vi "Main.vi"() -> ()   [LabVIEW 2014]
uses:
  <vilib>/Utility/config.llb/Write Key (String).vi
  <vilib>/Utility/config.llb/Write Key (Path).vi
  <vilib>/Utility/file.llb/Write To Spreadsheet File (string).vi
  <vilib>/Utility/config.llb/Read Key (String).vi
  <vilib>/Utility/config.llb/Read Key (Path).vi
  <vilib>/Utility/config.llb/NI_LVConfig.lvlib
panel:
  out "错误输出 2":errorcluster caption="错误输出"
  out "B结果信号":bool
  out "A结果信号":bool
  in  "scan A":bool
  in  "scan B":bool
  out "error out 4":errorcluster caption="错误输出"
  out "error out":errorcluster caption="错误输出"
  in  "打印标签路径B/Print label path B/Imprimer le chemin d’accès de l’étiquette B":path=path "D:/序列号B.txt"
  in  "打印标签路径A/Print label path A/Imprimer le chemin d’accès de l’étiquette A":path=path "D:/岚图A.btw"
  in  "3th Shift":timestamp format="%<%H:%M>T"
  in  "2nd Shift":timestamp format="%<%H:%M>T"
  in  "A启动信号":bool
  in  "B启动信号":bool
  in  "扫码在线过程":dbl
  in  "校准时间过程":i8
  out "错误输出  2":errorcluster caption="错误输出"
  out "error out 3":errorcluster
  out "error out 2":errorcluster
  in  "B复位":bool
  in  "A复位":bool
  out "Scan OK B":bool
  out "Scan OK A":bool
  out "错误输出":errorcluster
  in  "错误输入（无错误）":errorcluster
  out "结果 2":string
  in  "合格次数B":u16
  out "泄漏单位 2":string
  out "压力单位 2":string
  in  "检测次数B":u16
  in  "合格状态右":u16
  out "结果压力 B":dbl
  out "结果漏率 B":dbl
  out "合格 2":bool
  out "StepCode 2":u16
  out "Ready 2":bool
  out "StatusResults 2":u16 format="%b"
  out "实时漏率B":dbl
  out "LeakUnit 2":u16(ring) items=["ml/min"=51000, "cm3/s"=0, "cm3/min"=1000, "cm3/h"=2000, "mm3/h"=3000, "CalibartedPascal"=4000, "Pa"=6000, "Bar"=11000, "Kpa"=12000, "PSI"=13000, "Mbar"=14000, "Mpa"=15000, "Inch3/s"=46000, "Inch3/min"=47000, "Inch3/hour"=48000]
  out "PressureUnit 2":u16(ring) items=["cm3/s"=0, "cm3/min"=1000, "cm3/h"=2000, "mm3/h"=3000, "CalibartedPascal"=4000, "Pa"=6000, "Bar"=11000, "Kpa"=12000, "PSI"=13000, "Mbar"=14000, "Mpa"=15000, "Inch3/s"=46000, "Inch3/min"=47000, "Inch3/hour"=48000]
  out "ProgramNumber 2":u16
  out "实时压力B":dbl
  out "读取程序号B":bool
  out "读取程序号A":bool
  out "合格":bool
  out "StepCode":u16
  out "Ready":bool
  out "结果":string
  in  "合格次数A":u16
  out "泄漏单位":string
  out "压力单位":string
  in  "检测次数A":u16
  in  "合格状态左":u16
  out "StatusResults":u16 format="%b"
  out "实时漏率A":dbl
  out "LeakUnit":u16(ring) items=["ml/min"=51000, "cm3/s"=0, "cm3/min"=1000, "cm3/h"=2000, "mm3/h"=3000, "CalibartedPascal"=4000, "Pa"=6000, "Bar"=11000, "Kpa"=12000, "PSI"=13000, "Mbar"=14000, "Mpa"=15000, "Inch3/s"=46000, "Inch3/min"=47000, "Inch3/hour"=48000]
  out "PressureUnit":u16(ring) items=["cm3/s"=0, "cm3/min"=1000, "cm3/h"=2000, "mm3/h"=3000, "CalibartedPascal"=4000, "Pa"=6000, "Bar"=11000, "Kpa"=12000, "PSI"=13000, "Mbar"=14000, "Mpa"=15000, "Inch3/s"=46000, "Inch3/min"=47000, "Inch3/hour"=48000]
  out "ProgramNumber":u16
  out "实时压力A":dbl
  out "结果压力":dbl
  out "结果漏率":dbl
  in  "选项卡控件":T1(tab)
  out "校准倒计时":string
  out "B OK/NG":bool
  out "A OK/NG":bool
  in  "B标签重打":bool
  in  "A标签重打":bool
  in  "扫描枪重连":bool
  out "数字不跳动，表示软件死机 A":i32
  out "Scanner":bool
  out "ATEQ No. B":string
  out "ATEQ No. A":string
  in  "2D Code_B":string
  in  "Single/Dual B":bool
  in  "Total Today B":dbl
  in  "OK Today B":dbl
  in  "Staff B":u16(ring) items=["", "System", "复检", "谌春花", "辛飞琴", "周太珍", "周莎", "焦艳", "李腾", "吴有芳", "", "", "", "", "", "", "", "", "", "", "", "", "", "", ""]
  in  "Part No. B":u16(ring) items=["", "E113015200", "E113015300", "E122015400", "", "", "", "", "", "", "", "", "", "", "", "", "", "", "", "", "", "", "", "", ""]
  in  "B List":string[][](table)
  in  "2D Code_A":string
  in  "Single/Dual A":bool
  in  "Total Today A":dbl
  in  "OK Today A":dbl
  in  "Staff A":u16(ring) items=["", "System", "复检", "谌春花", "辛飞琴", "周太珍", "周莎", "焦艳", "李腾", "吴有芳", "", "", "", "", "", "", "", "", "", "", "", "", "", "", ""]
  in  "Part No. A":u16(ring) items=["", "E113015200", "E113015300", "E122015400", "", "", "", "", "", "", "", "", "", "", "", "", "", "", "", "", "", "", "", "", ""]
  in  "A List":string[][](table)
  out "数字不跳动，表示软件死机B":i32
  out "A Cal. Time":bool caption="A校准时间到"
  out "A OK Sample Req. (2nd)":bool caption="A校准时间到"
  out "A NG Sample Req.（1st)":bool caption="A校准时间到"
  in  "A Start Validation":bool
  out "B Cal. Time":bool caption="A校准时间到"
  out "B OK Sample Req. (2nd)":bool caption="A校准时间到"
  out "B NG Sample Req.（1st)":bool caption="A校准时间到"
  in  "B Start Validation":bool
  in  "密码":string
  in  "Confirm":bool
  in  "Cancel":bool
  in  "登录":u16(ring) items=["管理员", "作业员"]
  in  "A Cancel Validation":bool
  in  "B Cancel Validation":bool
  in  "Calitration Period (Hours)":timestamp format="%<%H:%M>T"
  in  "ATEQ F620 B (Restart Software to Active)":refnum<visa-resource-name>="COM6"
  in  "Language":u16(ring) items=["中文", "English", "Francais"]
  in  "保存确定":bool
  in  "参数设置/Setup/Coup monté":string[][](table) caption="参数设置"
  in  "ATEQ F620 A (Restart Software to Active)":refnum<visa-resource-name>="COM4"
  out "Scanner":bool
  in  "Download B":bool
  in  "Search B":bool
  in  "Finish Time B":timestamp format="%<%H:%M:%S\n%Y/%m/%d>T"
  in  "Result B":u16(ring) items=["", "OK", "NG"]
  in  "2D Code B":string
  in  "Start Time B":timestamp format="%<%H:%M:%S\n%Y/%m/%d>T"
  in  "Download A":bool
  in  "Search A":bool
  in  "Finish Time A":timestamp format="%<%H:%M:%S\n%Y/%m/%d>T"
  in  "Result A":u16(ring) items=["", "OK", "NG"]
  in  "2D Code A":string
  in  "Start Time A":timestamp format="%<%H:%M:%S\n%Y/%m/%d>T"
  in  "A List Search":string[][](table)
  in  "B List Search":string[][](table)
  in  "B自动/手动_Automatic/Manual_Automatique/Manual":bool
  in  "A自动/手动_Automatic/Manual_Automatique/Manual":bool
  in  "B门_Door_Porte：使能_Active_Activer/禁用_Deactive_Désactiver":bool
  in  "B盖章_Stamp_Timbre：后退_Back_Arrière/前进_forward_avant":bool
  in  "B封堵_Blocking_Bloquant：后退_Back_Arrière/前进_forward_avant":bool
  in  "B移载_Transfer_Transfert：后退_Back_Arrière/前进_forward_avant":bool
  in  "B夹紧_Clamping_Serrage：后退_Back_Arrière/前进_forward_avant":bool
  in  "A门_Door_Porte：使能_Active_Activer/禁用_Deactive_Désactiver":bool
  in  "A盖章_Stamp_Timbre：后退_Back_Arrière/前进_forward_avant":bool
  in  "A封堵_Blocking_Bloquant：后退_Back_Arrière/前进_forward_avant":bool
  in  "A移载_Transfer_Transfert：后退_Back_Arrière/前进_forward_avant":bool
  in  "A夹紧_Clamping_Serrage：后退_Back_Arrière/前进_forward_avant":bool
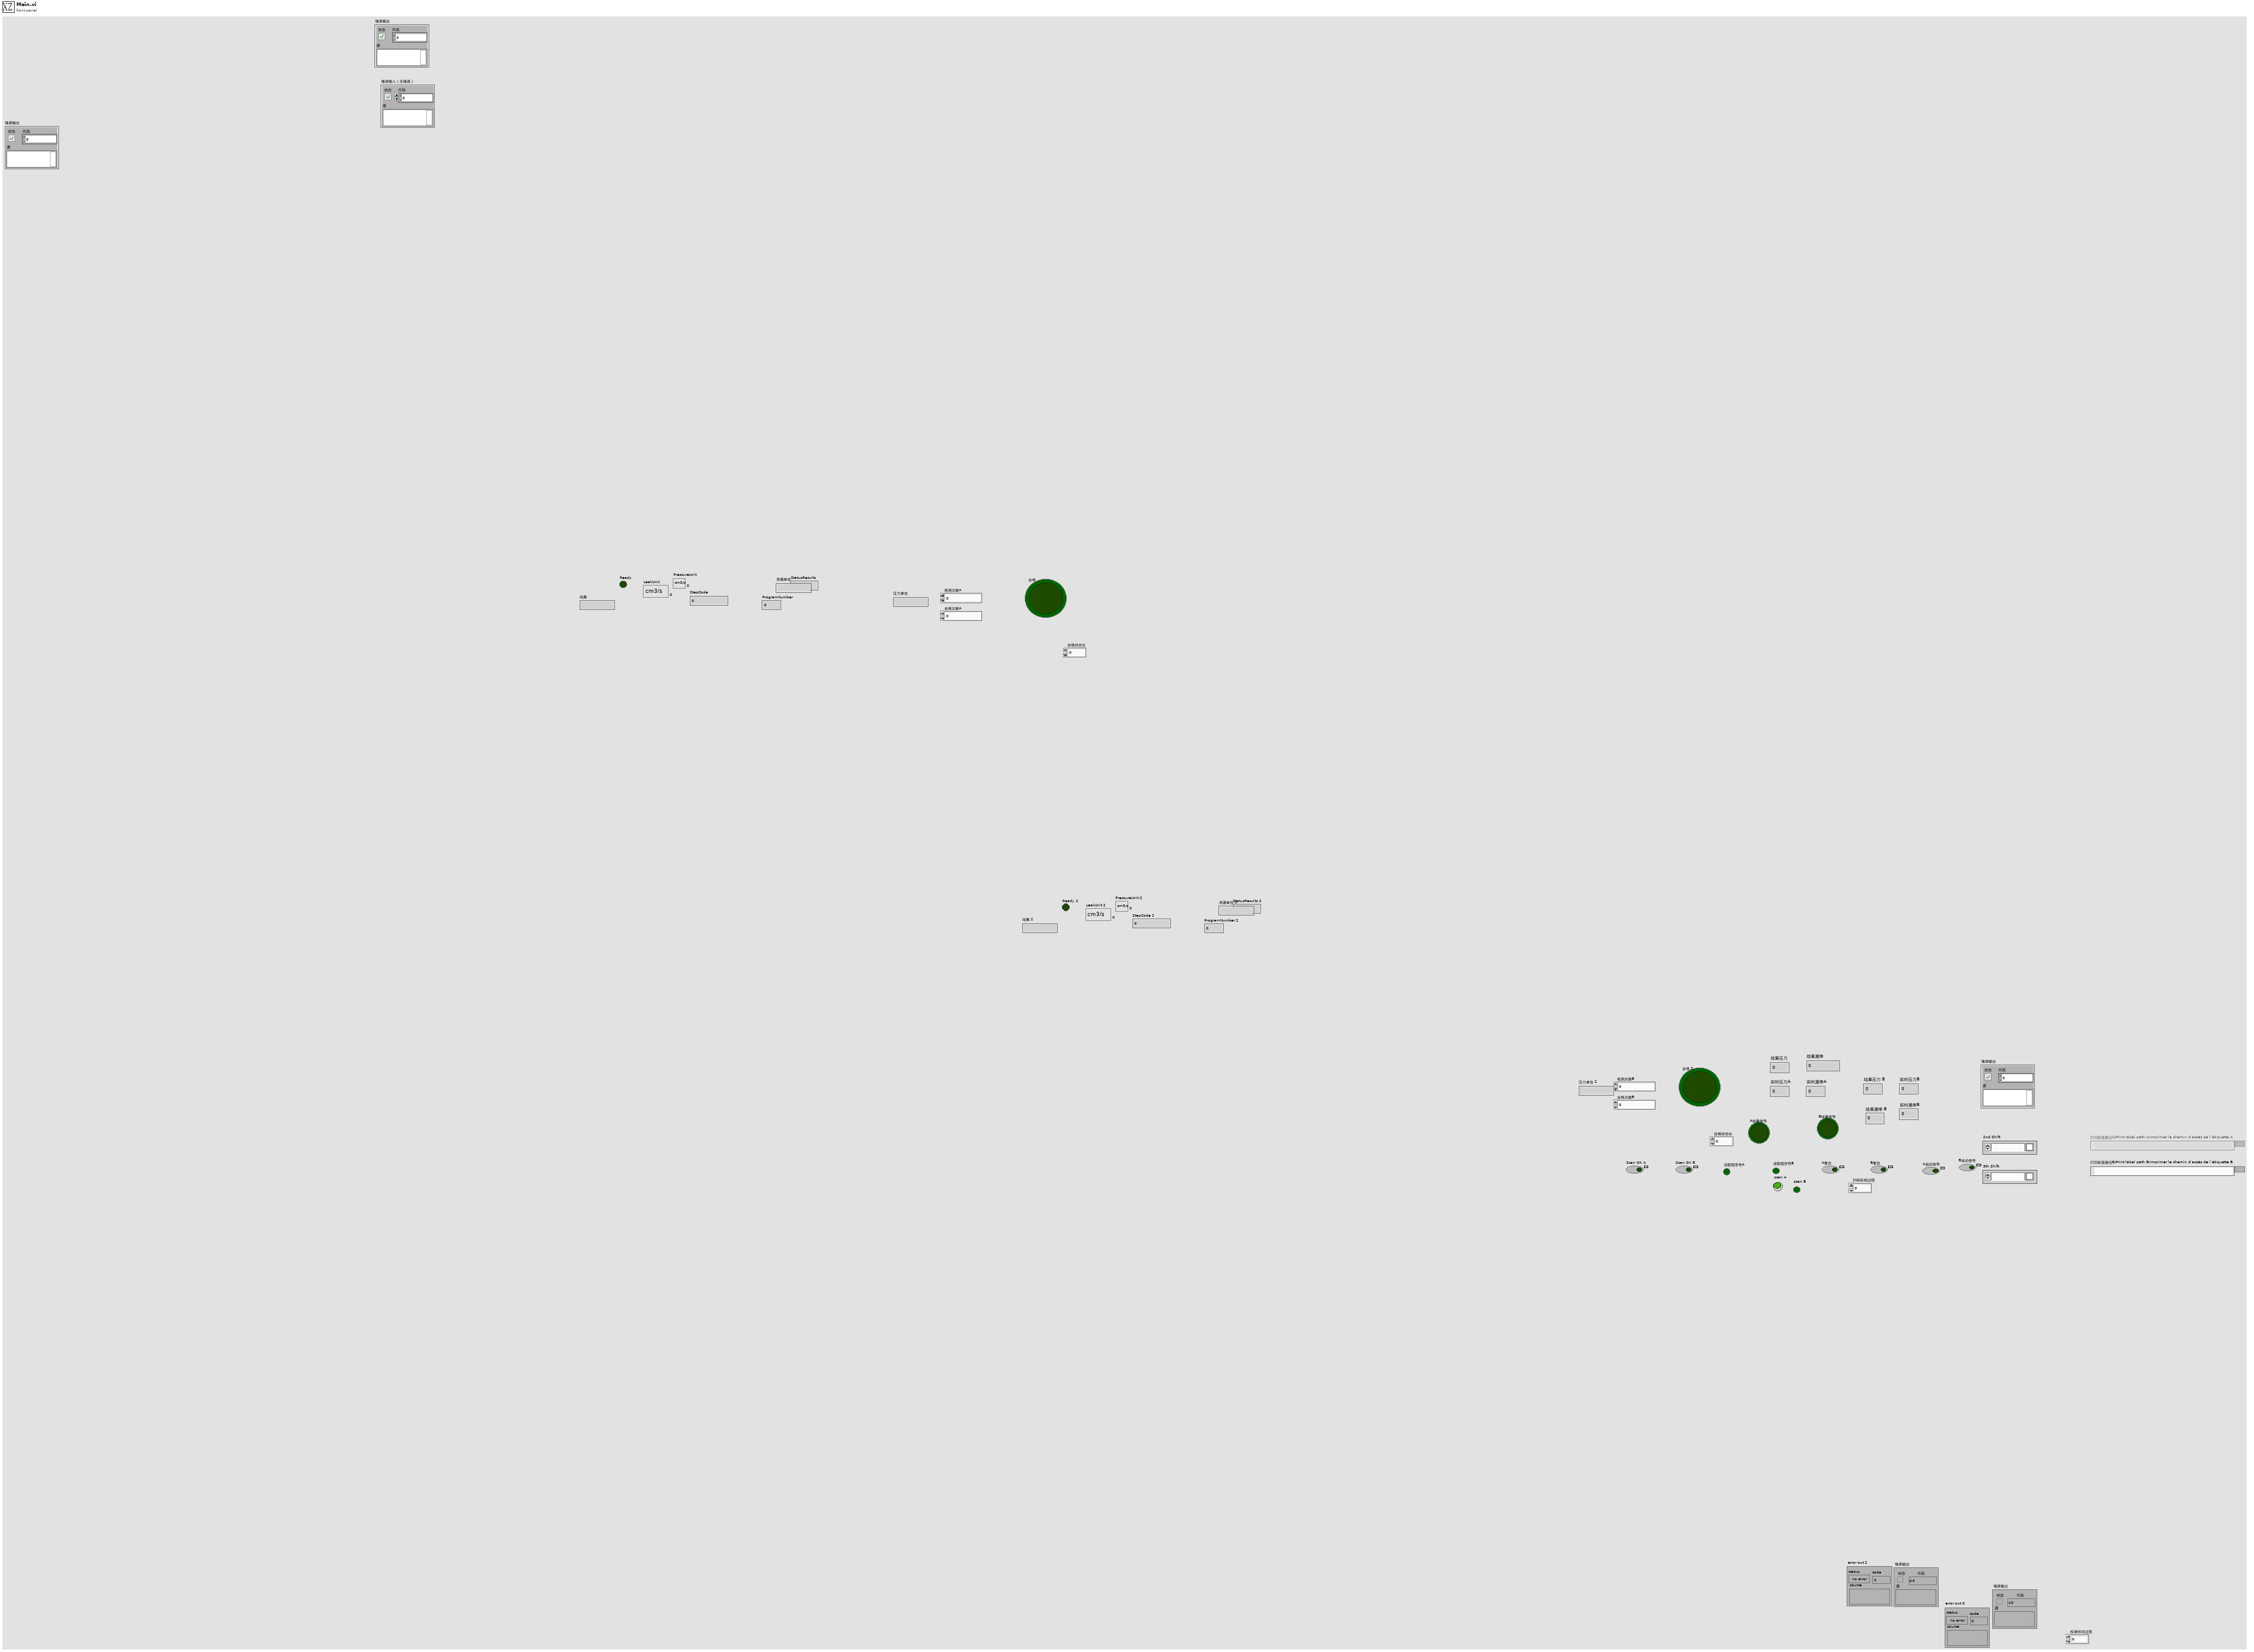
[diagram p1: front panel]
types:
  T1 = enum32{"测试/Main/Principale", "设置/Setup/Coup Monté", "查询/Query/Requête", "手动/Manual/Manuelle"}
  T2 = enum8{"Enabled", "Disabled", "Disabled and Grayed Out"}
  T3 = typedef "NI_LVConfig.lvlib/Config Data RefNum.ctl" = refnum<k1>
  T4 = enum16{"Init", "Loop", "Write LOFF", "Write LON", "Read", "Exit", "Open", "Close"}
  T5 = enum16{"Standard", "Buffered", "CRLF", "Immediate"}
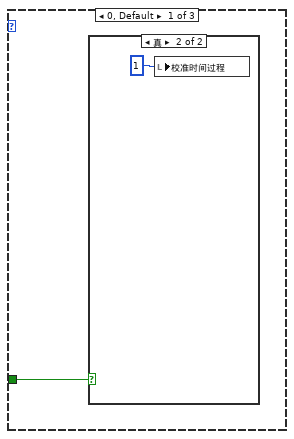
[diagram p3: hidden frame]
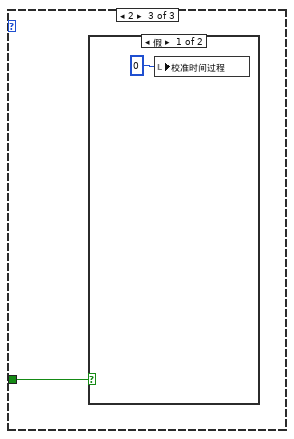
[diagram p6: hidden frame]
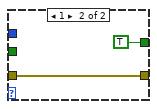
[diagram p8: hidden frame]
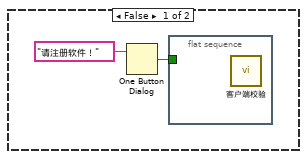
[diagram p9: hidden frame]
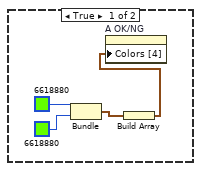
[diagram p10: hidden frame]
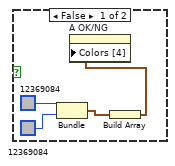
[diagram p11: hidden frame]
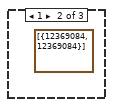
[diagram p13: hidden frame]
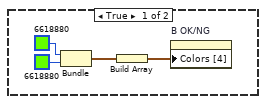
[diagram p15: hidden frame]
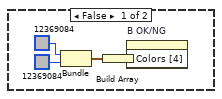
[diagram p16: hidden frame]
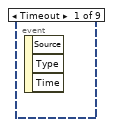
[diagram p20: hidden frame]
diagram:
  n1 = call "读写注册表.vi"("键名称"="license", "读/写"=enum16{"读", "写"}."读") -> ("error out"=w13:errorcluster, "键内容"=w10:string)  [unwired: 8 in]
  n2 = call "校验license.vi"("error in (no error)"=w13, "license"=w10) -> ("error out"=w9:errorcluster, "license正确"=w4:bool, "授权类型"=w8:i32, "T"=w7:u32)  [unwired: 6 in]
  n3 = call "判断时间正常.vi"("error in (no error)"=w9) -> ("error out"=w6:errorcluster, "时间正常"=w3:bool)  [unwired: 9 in]
  n4 = case shown="0, 默认" w8 {
    tunnel: w7 -> [w38 _]
    tunnel: [w33 TRUE ("试用期内")] -> w5
    tunnel: w6 -> [w37 w39]
    tunnel: w3 -> [w36 _]
    tunnel: [w32 w39] -> w2
    frame 0, Default {
      n5 = call "判断试用期.vi"("error in (no error)"=w37, "T"=w38) -> ("error out"=w32:errorcluster, "试用期内"=w35:bool)  [unwired: 8 in]
      n6 = Select(t=w35, s=w36, f=FALSE) -> (s? t:f=w33:bool)
    }
    frame 1 {
    }
  }
  n7 = flat-sequence {
    frame #0 {
      n8 = call <vilib>:"System Exec.vi"("run minimized? (F)"=TRUE, "wait until completion? (T)"=FALSE, "command line"="taskkill /f /im python.exe") -> ()  [unwired: 5 in, 4 out]
    }
    frame #1 {
      n9 = Wait (ms)(milliseconds to wait=u32 1000 ("等待时间（毫秒）")) -> ()  [unwired: 1 out]
    }
    frame #2 {
      n10 = call <vilib>:"System Exec.vi"("run minimized? (F)"=TRUE, "wait until completion? (T)"=TRUE, "command line"="\"d:\\miniconda3\\python.exe\" D:\\Data\\calibration.py ") -> ()  [unwired: 5 in, 4 out]
    }
  }
  n11 = And(x=w4, y=w5) -> (x .and. y?=w1:bool)
  n12 = call <vilib>:"Clear Errors.vi"("error in (no error)"=w2) -> ()  [unwired: 5 in, 2 out]
  n13 = case shown="真" w1 {
    frame False {
      n14 = One Button Dialog(message="请注册软件！" ("消息")) -> (true=w48:bool)  [unwired: 1 in]
      n15 = flat-sequence {
        tunnel: w48 -> [_]
        frame #0 {
          n16 = call "客户端校验.vi"() -> ()  [unwired: 12 in]
        }
      }
    }
    frame True {
      n17 = while {
        stop <- FALSE stop-if-true
        n18 = local read "读取程序号B"() -> (w89:bool)
        n19 = Wait (ms)(milliseconds to wait=u32 10 ("等待时间（毫秒）")) -> ()  [unwired: 1 out]
        n20 = case shown="假" w89 {
          tunnel: [w108 _] -> w87
          frame False {
            n21 = call "ReadRealStatus气密机一.vi"("从站地址"=u8 255, "VISA"="ATEQ F620 B (Restart Software to Active)", "baud rate"=u32 9600) -> ("Ready"=w91:bool, "Pass"=w92:bool, "StepCode"=w103:u16, "ProgramNumber"=→"ProgramNumber 2":u16, "Pressure"=w101:dbl, "PressureUnit"=→"PressureUnit 2":u16, "AL"=w105:bool, "Leak"=w102:dbl, "PressureAL"=w106:bool, "RD"=w107:bool, "TD"=w104:bool, "StatusResults"=→"StatusResults 2":u16, "LeakUnit"=→"LeakUnit 2":u16)
            "合格 2" <- w92
            "StepCode 2" <- w103
            "Ready 2" <- w91
            "实时漏率B" <- w102
            "实时压力B" <- w101
            n22 = And(x=w92, y=w91) -> (x .and. y?=w93:bool)
            n23 = case shown="6" w103 {
              tunnel: w102 -> [_ _ w123]
              tunnel: w101 -> [_ _ w122]
              frame 0, Default {
              }
              frame 1 {
              }
              frame 6 {
                "结果压力 B" <- w122
                "结果漏率 B" <- w123
              }
            }
            n24 = Compound Arithmetic op=OR ("复合运算")(w104, w107, w106, w105, w92) -> (w108:bool)
            n25 = case shown="假" w93 {
              tunnel: w91 -> [_ w113]
              frame True {
                n26 = Bundle(u32 6618880, u32 6618880) -> (w110:cluster{u32, u32})  [unwired: 1 in]
                n27 = Build Array(w110) -> (w109:cluster{u32, u32}[])
                n28 = property on="B OK/NG" class="Bool (严格)"("Colors [4]"=w109) -> ()  [unwired: 2 in, 2 out]
              }
              frame False {
                n29 = case shown="真" w113 {
                  frame False {
                    n30 = Bundle(u32 12369084, u32 12369084) -> (w115:cluster{u32, u32})  [unwired: 1 in]
                    n31 = Build Array(w115) -> (w114:cluster{u32, u32}[])
                    n32 = property on="B OK/NG" class="Bool (严格)"("Colors [4]"=w114) -> ()  [unwired: 2 in, 2 out]
                  }
                  frame True {
                    n33 = Bundle(u32 16711680, u32 16711680) -> (w119:cluster{u32, u32})  [unwired: 1 in]
                    n34 = Build Array(w119) -> (w118:cluster{u32, u32}[])
                    n35 = property on="B OK/NG" class="Bool (严格)"("Colors [4]"=w118) -> ()  [unwired: 2 in, 2 out]
                  }
                }
              }
            }
          }
          frame True {
          }
        }
        "B结果信号" <- w87
      }
      n36 = while {
        stop <- FALSE stop-if-true
        n37 = local read "读取程序号A"() -> (w51:bool)
        n38 = Wait (ms)(milliseconds to wait=u32 10 ("等待时间（毫秒）")) -> ()  [unwired: 1 out]
        n39 = case shown="假" w51 {
          tunnel: [w71 _] -> w50
          frame False {
            n40 = call "ReadRealStatus气密机一.vi"("从站地址"=u8 1, "VISA"="ATEQ F620 A (Restart Software to Active)", "baud rate"=u32 9600) -> ("Ready"=w54:bool, "Pass"=w56:bool, "StepCode"=w66:u16, "ProgramNumber"=→"ProgramNumber":u16, "Pressure"=w64:dbl, "PressureUnit"=→"PressureUnit":u16, "AL"=w68:bool, "Leak"=w65:dbl, "PressureAL"=w69:bool, "RD"=w70:bool, "TD"=w67:bool, "StatusResults"=→"StatusResults":u16, "LeakUnit"=→"LeakUnit":u16)
            "合格" <- w56
            "StepCode" <- w66
            "Ready" <- w54
            "实时漏率A" <- w65
            "实时压力A" <- w64
            n41 = And(x=w54, y=w56) -> (x .and. y?=w55:bool)
            n42 = case shown="假" w55 {
              tunnel: w54 -> [_ w76]
              frame True {
                n43 = Bundle(u32 6618880, u32 6618880) -> (w73:cluster{u32, u32})  [unwired: 1 in]
                n44 = Build Array(w73) -> (w72:cluster{u32, u32}[])
                n45 = property on="A OK/NG" class="Bool (严格)"("Colors [4]"=w72) -> ()  [unwired: 2 in, 2 out]
              }
              frame False {
                n46 = case shown="真" w76 {
                  frame False {
                    n47 = Bundle(u32 12369084, u32 12369084) -> (w78:cluster{u32, u32})  [unwired: 1 in]
                    n48 = Build Array(w78) -> (w77:cluster{u32, u32}[])
                    n49 = property on="A OK/NG" class="Bool (严格)"("Colors [4]"=w77) -> ()  [unwired: 2 in, 2 out]
                  }
                  frame True {
                    n50 = Bundle(u32 16711680, u32 16711680) -> (w82:cluster{u32, u32})  [unwired: 1 in]
                    n51 = Build Array(w82) -> (w81:cluster{u32, u32}[])
                    n52 = property on="A OK/NG" class="Bool (严格)"("Colors [4]"=w81) -> ()  [unwired: 2 in, 2 out]
                  }
                }
              }
            }
            n53 = case shown="6" w66 {
              tunnel: w65 -> [_ _ w86]
              tunnel: w64 -> [_ _ w85]
              frame 0, Default {
              }
              frame 1 {
                (unwired) cluster{u32, u32}[] [{12369084, 12369084}] ("颜色[4]")
              }
              frame 6 {
                "结果压力" <- w85
                "结果漏率" <- w86
              }
            }
            n54 = Compound Arithmetic op=OR ("复合运算")(w67, w70, w69, w68, w56) -> (w71:bool)
          }
          frame True {
          }
        }
        "A结果信号" <- w50
      }
    }
  }
  n55 = flat-sequence {
    frame #0 {
    }
    frame #1 {
    }
    frame #2 {
      n56 = Wait (ms)(milliseconds to wait=u32 1000 ("等待时间（毫秒）")) -> ()  [unwired: 1 out]
    }
    frame #3 {
      n57 = while {
        stop <- FALSE stop-if-true
        n58 = disable-structure shown="禁用" {
          frame Disabled {
            n59 = Format Date/Time String(time format string (%c)="%H:%M" ("时间格式字符串(%c)")) -> (date/time string=w163:string)  [unwired: 2 in]
            n60 = Get Date/Time String() -> (time string=w165:string)  [unwired: 3 in, 1 out]
            n61 = Format Date/Time String(time format string (%c)="%H:%M" ("时间格式字符串(%c)")) -> (date/time string=w160:string)  [unwired: 2 in]
            n62 = Get Date/Time String(seconds (now)="2nd Shift") -> (time string=w158:string)  [unwired: 2 in, 1 out]
            n63 = Format Date/Time String(time format string (%c)="%H:%M" ("时间格式字符串(%c)")) -> (date/time string=w153:string)  [unwired: 2 in]
            n64 = Get Date/Time String(seconds (now)="3th Shift") -> (time string=w155:string)  [unwired: 2 in, 1 out]
            n65 = Search and Replace String(input string=w163, search string=w165) -> (number of replacements=w162:i32)  [unwired: 6 in, 3 out]
            n66 = Search and Replace String(input string=w160, search string=w158) -> (number of replacements=w161:i32)  [unwired: 6 in, 3 out]
            n67 = Search and Replace String(input string=w153, search string=w155) -> (number of replacements=w152:i32)  [unwired: 6 in, 3 out]
            n68 = Equal?(x=w162, y=1) -> (x = y?=w151:bool)
            n69 = Equal?(x=w161, y=1) -> (x = y?=w150:bool)
            n70 = Equal?(x=w152, y=1) -> (x = y?=w149:bool)
            n71 = Compound Arithmetic op=OR(w151, w150, w149) -> ()  [unwired: 1 out]
          }
          frame Enabled {
          }
        }
        n72 = Read from Text File(file (use dialog)=path "D:/data/开始校准1.txt" ("文件（使用对话框）")) -> (text=w136:string)  [unwired: 3 in, 3 out]
        n73 = Format Date/Time String(time format string (%c)="%H:%M:%S" ("时间格式字符串(%c)"), seconds (now)="Calitration Period (Hours)") -> (date/time string=w130:string)  [unwired: 1 in]
        n74 = local read "合格状态右"() -> (w138:u16)
        n75 = local read "合格状态左"() -> (w144:u16)
        n76 = Decimal String To Number(string=w136) -> (number=w135:i32)  [unwired: 2 in, 1 out]
        n77 = Write to Text File(file (use dialog)=path "D:/data/校准间隔.txt" ("文件（使用对话框）"), text=w130) -> ()  [unwired: 2 in, 3 out]
        n78 = Equal?(x=w135, y=1) -> (x = y?=w133:bool)
        n79 = Not Equal?(x=w138, y=u16 1) -> (x != y?=w137:bool)
        n80 = Not Equal?(x=w144, y=u16 1) -> (x != y?=w142:bool)
        n81 = Read from Text File(file (use dialog)=path "D:/data/Time_Count.txt" ("文件（使用对话框）")) -> (text=→"校准倒计时":string, error out=→"错误输出 2":errorcluster)  [unwired: 3 in, 2 out]
        n82 = Compound Arithmetic op=AND(w133, w137, w142) -> (w141:bool)
        n83 = case shown="1" "校准时间过程" {
          tunnel: w141 -> [w167 _ w175]
          frame 0, Default {
            n84 = case shown="真" w167 {
              frame False {
              }
              frame True {
                n85 = local write "校准时间过程"(i8 1 ("校准时间过程")) -> ()
              }
            }
          }
          frame 1 {
            n86 = flat-sequence {
              frame #0 {
                w169 = TRUE ("确定")
                n87 = call "显示对话框信息"() -> ("OK"=w170:bool)  [unwired: 10 in, 1 out]
                n88 = case shown="真" w170 {
                  frame False {
                  }
                  frame True {
                    n89 = property on="选项卡控件" class="TabCtl (严格)"("Value"=T1."测试/Main/Principale" ("选项卡控件")) -> ()  [unwired: 2 in, 2 out]
                  }
                }
                "A Cal. Time" <- w169
                "B Cal. Time" <- w169
              }
              frame #1 {
                n90 = Write to Text File(file (use dialog)=path "D:/data/开始校准1.txt" ("文件（使用对话框）"), text="0" ("文本")) -> ()  [unwired: 2 in, 3 out]
              }
              frame #2 {
                n91 = local write "校准时间过程"(i8 2 ("校准时间过程")) -> ()
              }
            }
          }
          frame 2 {
            n92 = case shown="假" w175 {
              frame False {
                n93 = local write "校准时间过程"(i8 0 ("校准时间过程")) -> ()
              }
              frame True {
              }
            }
          }
        }
        n94 = Wait (ms)(milliseconds to wait=u32 100 ("等待时间（毫秒）")) -> ()  [unwired: 1 out]
      }
    }
  }
  n95 = flat-sequence {
    frame #0 {
      n96 = local write "读取程序号B"(TRUE ("读取程序号A")) -> ()
    }
    frame #1 {
      n97 = Wait (ms)(milliseconds to wait=u32 1000 ("等待时间（毫秒）")) -> ()  [unwired: 1 out]
    }
    frame #2 {
      n98 = property on="参数设置/Setup/Coup monté" class="Tbl (严格)"() -> ("Value"=w184:string[][])  [unwired: 2 in, 2 out]
      n99 = property on="ATEQ F620 B (Restart Software to Active)" class="VISAName"() -> ("Value"=w186:refnum<visa-resource-name>)  [unwired: 2 in, 2 out]
      n100 = property on="Part No. B" class="Ring (严格)"() -> ("Value"=w185:u16)  [unwired: 2 in, 2 out]
      n101 = Index Array(array=w184, index (row)=w185, index (col)=2 ("禁用的索引 (列)")) -> (element=w187:string)
      n102 = local write "ATEQ No. B"(w187) -> ()
      n103 = Decimal String To Number(string=w187) -> (number=w181:i32)  [unwired: 2 in, 1 out]
      n104 = Decrement(x=w181) -> (x-1=w191:i32)
      n105 = Quotient & Remainder(x=w181, y=2) -> (floor(x/y)=w179:i32)  [unwired: 1 out]
      n106 = case shown="1" w179 {
        frame 0, Default {
          n107 = local write "Single/Dual B"(FALSE) -> ()
        }
        frame 1 {
          n108 = local write "Single/Dual B"(FALSE) -> ()
        }
      }
      n109 = call "ATEQwrite程序选择.vi"("VISA resource name"=w186, "从站地址"=u8 255, "baud rate (9600)"=u32 9600, "The number of write"=u16 1, "实际程序号-1"=w191, "Write Address"=u16 2) -> ()  [unwired: 5 in, 1 out]
    }
    frame #3 {
      n110 = Wait (ms)(milliseconds to wait=u32 200 ("等待时间（毫秒）")) -> ()  [unwired: 1 out]
    }
    frame #4 {
      n111 = local write "读取程序号B"(FALSE ("读取程序号A")) -> ()
    }
  }
  n112 = flat-sequence {
    frame #0 {
      n113 = local write "读取程序号A"(TRUE ("读取程序号A")) -> ()
    }
    frame #1 {
      n114 = Wait (ms)(milliseconds to wait=u32 1010 ("等待时间（毫秒）")) -> ()  [unwired: 1 out]
    }
    frame #2 {
      n115 = property on="参数设置/Setup/Coup monté" class="Tbl (严格)"() -> ("Value"=w203:string[][])  [unwired: 2 in, 2 out]
      n116 = property on="ATEQ F620 A (Restart Software to Active)" class="VISAName"() -> ("Value"=w205:refnum<visa-resource-name>)  [unwired: 2 in, 2 out]
      n117 = property on="Part No. A" class="Ring (严格)"() -> ("Value"=w204:u16)  [unwired: 2 in, 2 out]
      n118 = Index Array(array=w203, index (row)=w204, index (col)=2 ("禁用的索引 (列)")) -> (element=w206:string)
      n119 = local write "ATEQ No. A"(w206) -> ()
      n120 = Decimal String To Number(string=w206) -> (number=w199:i32)  [unwired: 2 in, 1 out]
      n121 = Decrement(x=w199) -> (x-1=w210:i32)
      n122 = Quotient & Remainder(x=w199, y=2) -> (floor(x/y)=w198:i32)  [unwired: 1 out]
      n123 = case shown="1" w198 {
        frame 0, Default {
          n124 = local write "Single/Dual A"(FALSE) -> ()
        }
        frame 1 {
          n125 = local write "Single/Dual A"(FALSE) -> ()
        }
      }
      n126 = call "ATEQwrite程序选择.vi"("VISA resource name"=w205, "从站地址"=u8 1, "baud rate (9600)"=u32 9600, "The number of write"=u16 1, "实际程序号-1"=w210, "Write Address"=u16 2) -> ()  [unwired: 5 in, 1 out]
    }
    frame #3 {
      n127 = Wait (ms)(milliseconds to wait=u32 200 ("等待时间（毫秒）")) -> ()  [unwired: 1 out]
    }
    frame #4 {
      n128 = local write "读取程序号A"(FALSE ("读取程序号A")) -> ()
    }
  }
  n129 = while {
    stop <- FALSE stop-if-true
    n130 = event shown="[2] \"Part No. B\": 值改变" {
      selector: _ -> [_ _ _ _ _]
      dyn-events: _ -> [_ _ _ _ _]
      timeout: _ -> [_ _ _ _ _]
      event Timeout {
        n131 = event-data() -> ()  [unwired: 1 in, 3 out]
      }
      event "Part No. A": Value Change {
        n132 = event-data() -> ()  [unwired: 1 in, 6 out]
        n133 = flat-sequence {
          frame #0 {
            "读取程序号A" <- TRUE ("读取程序号A")
          }
          frame #1 {
            n134 = Wait (ms)(milliseconds to wait=u32 200 ("等待时间（毫秒）")) -> ()  [unwired: 1 out]
          }
          frame #2 {
            n135 = local write "合格次数A"(u16 0 ("检测次数B")) -> ()
            n136 = local write "检测次数A"(u16 0 ("检测次数B")) -> ()
            n137 = local write "A Cal. Time"(TRUE ("确定")) -> ()
            n138 = property on="参数设置/Setup/Coup monté" class="Tbl (严格)"() -> ("Value"=w227:string[][])  [unwired: 2 in, 2 out]
            n139 = call "显示对话框信息4"() -> ("OK"=w230:bool)  [unwired: 10 in, 1 out]
            n140 = property on="Part No. A" class="Ring (严格)"() -> ("Value"=w226:u16, "Strings []"=w228:string[])  [unwired: 2 in, 2 out]
            n141 = property on="ATEQ F620 A (Restart Software to Active)" class="VISAName"() -> ("Value"=w237:refnum<visa-resource-name>)  [unwired: 2 in, 2 out]
            n142 = case shown="真" w230 {
              frame False {
              }
              frame True {
                n143 = property on="选项卡控件" class="TabCtl (严格)"("Value"=T1."测试/Main/Principale" ("选项卡控件")) -> ()  [unwired: 2 in, 2 out]
              }
            }
            n144 = Index Array(array=w228, index=w226) -> (element=w224:string)
            n145 = Index Array(array=w227, index (row)=w226, index (col)=2 ("禁用的索引 (列)")) -> (element=w236:string)
            "ATEQ No. A" <- w236
            n146 = Index Array(array=w227, index (row)=w226, index (col)=1 ("禁用的索引 (列)")) -> (element=w221:string)
            n147 = Decimal String To Number(string=w236) -> (number=w233:i32)  [unwired: 2 in, 1 out]
            n148 = Write to Text File(file (use dialog)=path "d:/data/客户产品号A.txt" ("文件（使用对话框）"), text=w221) -> ()  [unwired: 2 in, 3 out]
            n149 = Write to Text File(file (use dialog)=path "d:/data/协众产品号A.txt" ("文件（使用对话框）"), text=w224) -> ()  [unwired: 2 in, 3 out]
            n150 = Decrement(x=w233) -> (x-1=w241:i32)
            n151 = Quotient & Remainder(x=w233, y=2) -> (x-y*floor(x/y)=w234:i32)  [unwired: 1 out]
            n152 = case shown="10, 默认" w234 {
              frame 1 {
                n153 = local write "Single/Dual A"(TRUE ("读取程序号A")) -> ()
              }
              frame 10, Default {
                n154 = local write "Single/Dual A"(FALSE ("读取程序号A")) -> ()
              }
            }
            n155 = call "ATEQwrite程序选择.vi"("VISA resource name"=w237, "从站地址"=u8 1, "baud rate (9600)"=u32 9600, "The number of write"=u16 1, "实际程序号-1"=w241, "Write Address"=u16 2) -> ()  [unwired: 5 in, 1 out]
          }
          frame #3 {
            n156 = Wait (ms)(milliseconds to wait=u32 200 ("等待时间（毫秒）")) -> ()  [unwired: 1 out]
          }
          frame #4 {
            n157 = local write "读取程序号A"(FALSE ("读取程序号A")) -> ()
          }
        }
      }
      event "Part No. B": Value Change {
        n158 = event-data() -> ()  [unwired: 1 in, 6 out]
        n159 = flat-sequence {
          frame #0 {
            "读取程序号B" <- TRUE ("读取程序号A")
          }
          frame #1 {
            n160 = Wait (ms)(milliseconds to wait=u32 200 ("等待时间（毫秒）")) -> ()  [unwired: 1 out]
          }
          frame #2 {
            n161 = local write "合格次数B"(u16 0 ("检测次数B")) -> ()
            n162 = local write "检测次数B"(u16 0 ("检测次数B")) -> ()
            n163 = local write "B Cal. Time"(TRUE ("确定")) -> ()
            n164 = property on="参数设置/Setup/Coup monté" class="Tbl (严格)"() -> ("Value"=w253:string[][])  [unwired: 2 in, 2 out]
            n165 = call "显示对话框信息3"() -> ("OK"=w260:bool)  [unwired: 10 in, 1 out]
            n166 = case shown="真" w260 {
              frame False {
              }
              frame True {
                n167 = property on="选项卡控件" class="TabCtl (严格)"("Value"=T1."测试/Main/Principale" ("选项卡控件")) -> ()  [unwired: 2 in, 2 out]
              }
            }
            n168 = property on="Part No. B" class="Ring (严格)"() -> ("Value"=w252:u16, "Strings []"=w257:string[])  [unwired: 2 in, 2 out]
            n169 = property on="ATEQ F620 B (Restart Software to Active)" class="VISAName"() -> ("Value"=w267:refnum<visa-resource-name>)  [unwired: 2 in, 2 out]
            n170 = Index Array(array=w257, index=w252) -> (element=w256:string)
            n171 = Index Array(array=w253, index (row)=w252, index (col)=2 ("禁用的索引 (列)")) -> (element=w265:string)
            "ATEQ No. B" <- w265
            n172 = Index Array(array=w253, index (row)=w252, index (col)=1 ("禁用的索引 (列)")) -> (element=w255:string)
            n173 = Decimal String To Number(string=w265) -> (number=w263:i32)  [unwired: 2 in, 1 out]
            n174 = Write to Text File(file (use dialog)=path "d:/data/客户产品号B.txt" ("文件（使用对话框）"), text=w255) -> ()  [unwired: 2 in, 3 out]
            n175 = Write to Text File(file (use dialog)=path "d:/data/协众产品号B.txt" ("文件（使用对话框）"), text=w256) -> ()  [unwired: 2 in, 3 out]
            n176 = Decrement(x=w263) -> (x-1=w271:i32)
            n177 = Quotient & Remainder(x=w263, y=2) -> (x-y*floor(x/y)=w264:i32)  [unwired: 1 out]
            n178 = case shown="10, 默认" w264 {
              frame 1 {
                n179 = local write "Single/Dual B"(TRUE ("读取程序号A")) -> ()
              }
              frame 10, Default {
                n180 = local write "Single/Dual B"(FALSE ("读取程序号A")) -> ()
              }
            }
            n181 = call "ATEQwrite程序选择.vi"("VISA resource name"=w267, "从站地址"=u8 255, "baud rate (9600)"=u32 9600, "The number of write"=u16 1, "实际程序号-1"=w271, "Write Address"=u16 2) -> ()  [unwired: 5 in, 1 out]
          }
          frame #3 {
            n182 = Wait (ms)(milliseconds to wait=u32 200 ("等待时间（毫秒）")) -> ()  [unwired: 1 out]
          }
          frame #4 {
            n183 = local write "读取程序号B"(FALSE ("读取程序号A")) -> ()
          }
        }
      }
      event "Single/Dual A": Value Change {
        n184 = event-data() -> ()  [unwired: 1 in, 6 out]
        n185 = local read "Single/Dual A"() -> (w279:bool)
        n186 = local write "检测次数A"(u16 0 ("检测次数B")) -> ()
        n187 = local write "合格次数A"(u16 0 ("检测次数B")) -> ()
        n188 = case shown="假" w279 {
          frame True {
            n189 = property on="Language" class="Ring (严格)"() -> ("Value"=w280:u16)  [unwired: 2 in, 2 out]
            n190 = case shown="2" w280 {
              frame 0, Default {
                n191 = property on="Single/Dual A" class="Bool (严格)"("BoolText.Text"="双腔测试" ("布尔文本.文本")) -> ()  [unwired: 2 in, 2 out]
              }
              frame 1 {
                n192 = property on="Single/Dual A" class="Bool (严格)"("BoolText.Text"="Dual Tests" ("布尔文本.文本")) -> ()  [unwired: 2 in, 2 out]
              }
              frame 2 {
                n193 = property on="Single/Dual A" class="Bool (严格)"("BoolText.Text"="Double Tests" ("布尔文本.文本")) -> ()  [unwired: 2 in, 2 out]
              }
            }
          }
          frame False {
            n194 = property on="Language" class="Ring (严格)"() -> ("Value"=w284:u16)  [unwired: 2 in, 2 out]
            n195 = case shown="1" w284 {
              frame 0, Default {
                n196 = property on="Single/Dual A" class="Bool (严格)"("BoolText.Text"="单腔测试" ("布尔文本.文本")) -> ()  [unwired: 2 in, 2 out]
              }
              frame 1 {
                n197 = property on="Single/Dual A" class="Bool (严格)"("BoolText.Text"="Single Test" ("布尔文本.文本")) -> ()  [unwired: 2 in, 2 out]
              }
              frame 2 {
                n198 = property on="Single/Dual A" class="Bool (严格)"("BoolText.Text"="Unique Test" ("布尔文本.文本")) -> ()  [unwired: 2 in, 2 out]
              }
            }
          }
        }
      }
      event "Single/Dual B": Value Change {
        n199 = event-data() -> ()  [unwired: 1 in, 6 out]
        n200 = local read "Single/Dual B"() -> (w290:bool)
        n201 = local write "检测次数B"(u16 0 ("检测次数B")) -> ()
        n202 = local write "合格次数B"(u16 0 ("检测次数B")) -> ()
        n203 = case shown="真" w290 {
          frame True {
            n204 = property on="Language" class="Ring (严格)"() -> ("Value"=w291:u16)  [unwired: 2 in, 2 out]
            n205 = case shown="1" w291 {
              frame 0, Default {
                n206 = property on="Single/Dual B" class="Bool (严格)"("BoolText.Text"="双腔测试" ("布尔文本.文本")) -> ()  [unwired: 2 in, 2 out]
              }
              frame 1 {
                n207 = property on="Single/Dual B" class="Bool (严格)"("BoolText.Text"="Dual Tests" ("布尔文本.文本")) -> ()  [unwired: 2 in, 2 out]
              }
              frame 2 {
                n208 = property on="Single/Dual B" class="Bool (严格)"("BoolText.Text"="Double Tests" ("布尔文本.文本")) -> ()  [unwired: 2 in, 2 out]
              }
            }
          }
          frame False {
            n209 = property on="Language" class="Ring (严格)"() -> ("Value"=w295:u16)  [unwired: 2 in, 2 out]
            n210 = case shown="2" w295 {
              frame 0, Default {
                n211 = property on="Single/Dual B" class="Bool (严格)"("BoolText.Text"="单腔测试" ("布尔文本.文本")) -> ()  [unwired: 2 in, 2 out]
              }
              frame 1 {
                n212 = property on="Single/Dual B" class="Bool (严格)"("BoolText.Text"="Single Test" ("布尔文本.文本")) -> ()  [unwired: 2 in, 2 out]
              }
              frame 2 {
                n213 = property on="Single/Dual B" class="Bool (严格)"("BoolText.Text"="Unique Test" ("布尔文本.文本")) -> ()  [unwired: 2 in, 2 out]
              }
            }
          }
        }
      }
    }
    n214 = Wait (ms)(milliseconds to wait=u32 100 ("等待时间（毫秒）")) -> ()  [unwired: 1 out]
  }
  n215 = while {
    stop <- FALSE stop-if-true
    n216 = event shown="[4] \"Cancel\": 鼠标释放" {
      selector: _ -> [_ _ _ _ _ _ _ _ _]
      dyn-events: _ -> [_ _ _ _ _ _ _ _ _]
      timeout: _ -> [_ _ _ _ _ _ _ _ _]
      event Timeout {
        n217 = event-data() -> ()  [unwired: 1 in, 3 out]
      }
      event "A Start Validation": Mouse Up {
        w303 = TRUE
        n218 = event-data() -> ()  [unwired: 1 in, 8 out]
        n219 = local write "检测次数A"(u16 0 ("检测次数B")) -> ()
        n220 = local write "合格次数A"(u16 0 ("检测次数B")) -> ()
        n221 = local write "A NG Sample Req.（1st)"(w303) -> ()
        n222 = local write "A OK Sample Req. (2nd)"(w303) -> ()
        n223 = local write "A Cal. Time"(w303) -> ()
      }
      event "B Start Validation": Mouse Up {
        w306 = TRUE
        n224 = event-data() -> ()  [unwired: 1 in, 8 out]
        n225 = local write "检测次数B"(u16 0 ("检测次数B")) -> ()
        n226 = local write "合格次数B"(u16 0 ("检测次数B")) -> ()
        n227 = local write "B NG Sample Req.（1st)"(w306) -> ()
        n228 = local write "B Cal. Time"(w306) -> ()
        n229 = local write "B OK Sample Req. (2nd)"(w306) -> ()
      }
      event "Confirm": Mouse Up {
        n230 = property on="密码" class="Str"() -> ("Value"=w320:string)  [unwired: 2 in, 2 out]
        n231 = event-data() -> ()  [unwired: 1 in, 8 out]
        n232 = property on="登录" class="Ring (严格)"() -> ("Strings []"=w330:string[], "Value"=w329:u16)  [unwired: 2 in, 2 out]
        n233 = Index Array(array=w330, index=w329) -> (element=w322:string)
        n234 = Search and Replace String(input string=w322, search string="管理员") -> (number of replacements=w327:i32)  [unwired: 6 in, 3 out]
        n235 = Search and Replace String(input string=w322, search string="作业员") -> (number of replacements=w324:i32)  [unwired: 6 in, 3 out]
        n236 = Equal?(x=w324, y=1) -> (x = y?=w313:bool)
        n237 = Read from Text File(file (use dialog)=path "d:/data/管理员.txt" ("文件（使用对话框）")) -> (text=w308:string)  [unwired: 3 in, 3 out]
        n238 = Read from Text File(file (use dialog)=path "d:/data/作业员.txt" ("文件（使用对话框）")) -> (text=w307:string)  [unwired: 3 in, 3 out]
        n239 = Equal?(x=w327, y=1) -> (x = y?=w315:bool)
        n240 = Search and Replace String(input string=w320, search string=w308) -> (number of replacements=w319:i32)  [unwired: 6 in, 3 out]
        n241 = Search and Replace String(input string=w320, search string=w307) -> (number of replacements=w317:i32)  [unwired: 6 in, 3 out]
        n242 = Equal?(x=w319, y=1) -> (x = y?=w316:bool)
        n243 = Equal?(x=w317, y=1) -> (x = y?=w314:bool)
        n244 = And(x=w316, y=w315) -> (x .and. y?=w312:bool)
        n245 = And(x=w314, y=w313) -> (x .and. y?=w311:bool)
        n246 = case shown="真" w312 {
          frame False {
          }
          frame True {
            w336 = TRUE
            w334 = T2."Enabled" ("禁用")
            n247 = property on="A Cancel Validation" class="Bool"("Visible"=w336) -> ()  [unwired: 2 in, 2 out]
            n248 = property on="B Cancel Validation" class="Bool"("Visible"=w336) -> ()  [unwired: 2 in, 2 out]
            n249 = local write "密码"("") -> ()
            n250 = property on="Staff B" class="Ring (严格)"("DisabledEnum"=w334) -> ()  [unwired: 2 in, 2 out]
            n251 = property on="A Cancel Validation" class="Bool"("DisabledEnum"=w334) -> ()  [unwired: 2 in, 2 out]
            n252 = property on="2nd Shift" class="AbsTime (严格)"("DisabledEnum"=w334) -> ()  [unwired: 2 in, 2 out]
            n253 = property on="Part No. B" class="Ring (严格)"("DisabledEnum"=w334) -> ()  [unwired: 2 in, 2 out]
            n254 = property on="参数设置/Setup/Coup monté" class="Tbl (严格)"("DisabledEnum"=w334) -> ()  [unwired: 2 in, 2 out]
            n255 = property on="Staff A" class="Ring (严格)"("DisabledEnum"=w334) -> ()  [unwired: 2 in, 2 out]
            n256 = property on="打印标签路径B/Print label path B/Imprimer le chemin d’accès de l’étiquette B" class="Path"("DisabledEnum"=w334) -> ()  [unwired: 2 in, 2 out]
            n257 = property on="Part No. A" class="Ring (严格)"("DisabledEnum"=w334) -> ()  [unwired: 2 in, 2 out]
            n258 = property on="Calitration Period (Hours)" class="AbsTime (严格)"("DisabledEnum"=w334) -> ()  [unwired: 2 in, 2 out]
            n259 = property on="B Cancel Validation" class="Bool"("DisabledEnum"=w334) -> ()  [unwired: 2 in, 2 out]
            n260 = property on="3th Shift" class="AbsTime (严格)"("DisabledEnum"=w334) -> ()  [unwired: 2 in, 2 out]
            n261 = property on="打印标签路径A/Print label path A/Imprimer le chemin d’accès de l’étiquette A" class="Path"("DisabledEnum"=w334) -> ()  [unwired: 2 in, 2 out]
            n262 = property on="ATEQ F620 A (Restart Software to Active)" class="VISAName"("DisabledEnum"=w334) -> ()  [unwired: 2 in, 2 out]
            n263 = property on="ATEQ F620 B (Restart Software to Active)" class="VISAName"("DisabledEnum"=w334) -> ()  [unwired: 2 in, 2 out]
            n264 = property on="保存确定" class="Bool"("DisabledEnum"=w334) -> ()  [unwired: 2 in, 2 out]
          }
        }
        n265 = case shown="真" w311 {
          frame False {
          }
          frame True {
            n266 = disable-structure shown="禁用" {
              frame Disabled {
                w332 = TRUE
                w333 = T2."Enabled" ("禁用")
                n267 = property on="A Cancel Validation" class="Bool"("Visible"=w332) -> ()  [unwired: 2 in, 2 out]
                n268 = property on="B Cancel Validation" class="Bool"("Visible"=w332) -> ()  [unwired: 2 in, 2 out]
                n269 = property on="Staff B" class="Ring (严格)"("DisabledEnum"=w333) -> ()  [unwired: 2 in, 2 out]
                n270 = property on="A Cancel Validation" class="Bool"("DisabledEnum"=w333) -> ()  [unwired: 2 in, 2 out]
                n271 = property on="Part No. B" class="Ring (严格)"("DisabledEnum"=w333) -> ()  [unwired: 2 in, 2 out]
                n272 = property on="Staff A" class="Ring (严格)"("DisabledEnum"=w333) -> ()  [unwired: 2 in, 2 out]
                n273 = property on="打印标签路径B/Print label path B/Imprimer le chemin d’accès de l’étiquette B" class="Path"("DisabledEnum"=w333) -> ()  [unwired: 2 in, 2 out]
                n274 = property on="Part No. A" class="Ring (严格)"("DisabledEnum"=w333) -> ()  [unwired: 2 in, 2 out]
                n275 = property on="Calitration Period (Hours)" class="AbsTime (严格)"("DisabledEnum"=w333) -> ()  [unwired: 2 in, 2 out]
                n276 = property on="B Cancel Validation" class="Bool"("DisabledEnum"=w333) -> ()  [unwired: 2 in, 2 out]
                n277 = property on="3th Shift" class="AbsTime (严格)"("DisabledEnum"=w333) -> ()  [unwired: 2 in, 2 out]
                n278 = property on="2nd Shift" class="AbsTime (严格)"("DisabledEnum"=w333) -> ()  [unwired: 2 in, 2 out]
                n279 = property on="打印标签路径A/Print label path A/Imprimer le chemin d’accès de l’étiquette A" class="Path"("DisabledEnum"=w333) -> ()  [unwired: 2 in, 2 out]
              }
              frame Enabled {
              }
            }
            n280 = local write "密码"("") -> ()
          }
        }
      }
      event "Cancel": Mouse Up {
        w338 = FALSE
        w337 = T2."Disabled and Grayed Out" ("禁用")
        n281 = event-data() -> ()  [unwired: 1 in, 8 out]
        n282 = local write "密码"("") -> ()
        n283 = property on="A Cancel Validation" class="Bool"("Visible"=w338) -> ()  [unwired: 2 in, 2 out]
        n284 = property on="B Cancel Validation" class="Bool"("Visible"=w338) -> ()  [unwired: 2 in, 2 out]
        n285 = property on="A Cancel Validation" class="Bool"("DisabledEnum"=w337) -> ()  [unwired: 2 in, 2 out]
        n286 = property on="参数设置/Setup/Coup monté" class="Tbl (严格)"("DisabledEnum"=w337) -> ()  [unwired: 2 in, 2 out]
        n287 = property on="2nd Shift" class="AbsTime (严格)"("DisabledEnum"=w337) -> ()  [unwired: 2 in, 2 out]
        n288 = property on="打印标签路径B/Print label path B/Imprimer le chemin d’accès de l’étiquette B" class="Path"("DisabledEnum"=w337) -> ()  [unwired: 2 in, 2 out]
        n289 = property on="Calitration Period (Hours)" class="AbsTime (严格)"("DisabledEnum"=w337) -> ()  [unwired: 2 in, 2 out]
        n290 = property on="B Cancel Validation" class="Bool"("DisabledEnum"=w337) -> ()  [unwired: 2 in, 2 out]
        n291 = property on="打印标签路径A/Print label path A/Imprimer le chemin d’accès de l’étiquette A" class="Path"("DisabledEnum"=w337) -> ()  [unwired: 2 in, 2 out]
        n292 = property on="3th Shift" class="AbsTime (严格)"("DisabledEnum"=w337) -> ()  [unwired: 2 in, 2 out]
        n293 = property on="ATEQ F620 A (Restart Software to Active)" class="VISAName"("DisabledEnum"=w337) -> ()  [unwired: 2 in, 2 out]
        n294 = property on="ATEQ F620 B (Restart Software to Active)" class="VISAName"("DisabledEnum"=w337) -> ()  [unwired: 2 in, 2 out]
        n295 = property on="保存确定" class="Bool"("DisabledEnum"=w337) -> ()  [unwired: 2 in, 2 out]
      }
      event "A标签重打": Mouse Up {
        n296 = event-data() -> ()  [unwired: 1 in, 8 out]
        n297 = Read from Text File(file (use dialog)=path "d:/data/打印路径A.txt" ("文件（使用对话框）")) -> (text=w345:string)  [unwired: 3 in, 3 out]
        n298 = Concatenate Strings("\"C:\\Program Files\\Seagull\\BarTender Suite\\bartend.exe\" " ("command line"), w345, " /P/min=SystemTray" ("command line")) -> (w342:string)
        n299 = call <vilib>:"System Exec.vi"("run minimized? (F)"=TRUE, "wait until completion? (T)"=FALSE, "command line"=w342) -> ()  [unwired: 5 in, 4 out]
      }
      event "B标签重打": Mouse Up {
        n300 = event-data() -> ()  [unwired: 1 in, 8 out]
        n301 = Read from Text File(file (use dialog)=path "d:/data/打印路径B.txt" ("文件（使用对话框）")) -> (text=w352:string)  [unwired: 3 in, 3 out]
        n302 = Concatenate Strings("\"C:\\Program Files\\Seagull\\BarTender Suite\\bartend.exe\" " ("command line"), w352, " /P/min=SystemTray" ("command line")) -> (w349:string)
        n303 = call <vilib>:"System Exec.vi"("run minimized? (F)"=TRUE, "wait until completion? (T)"=FALSE, "command line"=w349) -> ()  [unwired: 5 in, 4 out]
      }
      event "A Cancel Validation": Value Change {
        w356 = FALSE
        n304 = event-data() -> ()  [unwired: 1 in, 6 out]
        n305 = local write "检测次数A"(u16 0 ("检测次数B")) -> ()
        n306 = local write "合格次数A"(u16 0 ("检测次数B")) -> ()
        n307 = local write "A Cal. Time"(w356) -> ()
        n308 = local write "A OK Sample Req. (2nd)"(w356) -> ()
        n309 = local write "A NG Sample Req.（1st)"(w356) -> ()
      }
      event "B Cancel Validation": Value Change {
        w359 = FALSE
        n310 = event-data() -> ()  [unwired: 1 in, 6 out]
        n311 = local write "检测次数B"(u16 0 ("检测次数B")) -> ()
        n312 = local write "合格次数B"(u16 0 ("检测次数B")) -> ()
        n313 = local write "B Cal. Time"(w359) -> ()
        n314 = local write "B OK Sample Req. (2nd)"(w359) -> ()
        n315 = local write "B NG Sample Req.（1st)"(w359) -> ()
      }
    }
    n316 = Wait (ms)(milliseconds to wait=u32 100 ("等待时间（毫秒）")) -> ()  [unwired: 1 out]
  }
  n317 = while {
    stop <- FALSE stop-if-true
    n318 = event shown="[2] \"A Start Validation\": 鼠标释放" {
      selector: _ -> [_ _ _ _]
      dyn-events: _ -> [_ _ _ _]
      timeout: _ -> [_ _ _ _]
      event Timeout {
        n319 = event-data() -> ()  [unwired: 1 in, 3 out]
      }
      event "Language": Value Change {
        n320 = event-data() -> ("NewVal"=w361:u16)  [unwired: 1 in, 5 out]
        n321 = case shown="2" w361 {
          frame 0, Default {
            n322 = for {
              N: 1000 -> [_]
              shift-right: [w419] -> _
              shift-left: _ -> [_]
              tunnel: [w418] -> w363 mode=indexing
              i -> [w420]
              n323 = Add(x=1, y=w420) -> (x+y=w419:i32)
              n324 = Number To Decimal String(number=w419) -> (decimal integer string=w418:string)  [unwired: 1 in]
            }
            n325 = Build Array("时间", "序列号", "二维码", "#1 压力", "#1 漏率", "#2 压力", "#2 漏率", "结果", "产品型号" ("元素"), "人员") -> (w362:string[])
            n326 = property on="A List" class="Tbl (严格)"("Number of Rows"=u32 1000 ("行数"), "Number of Columns"=u32 10 ("列数"), "Row Headers[]"=w363, "Column Headers[]"=w362, "Height"=u32 840 ("大小:高度"), "Width"=u32 900 ("大小:宽度")) -> ("Number of Rows"=w389:u32, "Number of Columns"=w386:u32, "Value"=w391:string[][])  [unwired: 2 in, 2 out]
            n327 = property on="B List" class="Tbl (严格)"("Number of Rows"=u32 1000 ("行数"), "Number of Columns"=u32 10 ("列数"), "Row Headers[]"=w363, "Column Headers[]"=w362, "Height"=u32 840 ("大小:高度"), "Width"=u32 900 ("大小:宽度")) -> ("Number of Rows"=w368:u32, "Number of Columns"=w371:u32, "Value"=w366:string[][])  [unwired: 2 in, 2 out]
            n328 = Array Size(array=w391) -> (size(s)=w390:i32[])
            n329 = Array Size(array=w366) -> (size(s)=w367:i32[])
            n330 = Index Array(array=w390) -> (element #1=w388:i32, element #2=w387:i32)  [unwired: 2 in]
            n331 = Index Array(array=w367) -> (element #1=w369:i32, element #2=w370:i32)  [unwired: 2 in]
            n332 = Max & Min(x=w389, y=w388) -> (max(x,y)=w385:u32)  [unwired: 1 out]
            n333 = Max & Min(x=w386, y=w387) -> (max(x,y)=w384:u32)  [unwired: 1 out]
            n334 = Max & Min(x=w368, y=w369) -> (max(x,y)=w372:u32)  [unwired: 1 out]
            n335 = Max & Min(x=w371, y=w370) -> (max(x,y)=w373:u32)  [unwired: 1 out]
            n336 = for {
              N: w385 -> [_]
              tunnel: w384 -> [w406]
              tunnel: u32 16448250 -> [w405]
              tunnel: u32 13816530 -> [w404]
              i -> [w403]
              n337 = for {
                N: w406 -> [_]
                tunnel: w403 -> [w417]
                tunnel: w405 -> [w411]
                tunnel: w404 -> [w410]
                tunnel: w403 -> [w408]
                i -> [w416]
                n338 = Quotient & Remainder(x=w408, y=u32 2) -> (x-y*floor(x/y)=w414:u32)  [unwired: 1 out]
                n339 = Equal?(x=w414, y=u32 0) -> (x = y?=w412:bool)
                n340 = Select(t=w411, s=w412, f=w410) -> (s? t:f=w409:u32)
                n341 = Bundle(w417, w416) -> (w407:cluster{i32, i32})  [unwired: 1 in]
                n342 = property on="A List" class="Tbl (严格)"("Active Cell"=w407, "Cell BG Color"=w409) -> ()  [unwired: 2 in, 2 out]
              }
            }
            n343 = for {
              N: w372 -> [_]
              tunnel: w373 -> [w425]
              tunnel: u32 16448250 -> [w424]
              tunnel: u32 13816530 -> [w423]
              i -> [w422]
              n344 = for {
                N: w425 -> [_]
                tunnel: w422 -> [w436]
                tunnel: w424 -> [w430]
                tunnel: w423 -> [w429]
                tunnel: w422 -> [w427]
                i -> [w435]
                n345 = Quotient & Remainder(x=w427, y=u32 2) -> (x-y*floor(x/y)=w433:u32)  [unwired: 1 out]
                n346 = Equal?(x=w433, y=u32 0) -> (x = y?=w431:bool)
                n347 = Select(t=w430, s=w431, f=w429) -> (s? t:f=w428:u32)
                n348 = Bundle(w436, w435) -> (w426:cluster{i32, i32})  [unwired: 1 in]
                n349 = property on="B List" class="Tbl (严格)"("Active Cell"=w426, "Cell BG Color"=w428) -> ()  [unwired: 2 in, 2 out]
              }
            }
          }
          frame 1 {
            n350 = for {
              N: 1000 -> [_]
              shift-right: [w494] -> _
              shift-left: _ -> [_]
              tunnel: [w493] -> w438 mode=indexing
              i -> [w495]
              n351 = Add(x=1, y=w495) -> (x+y=w494:i32)
              n352 = Number To Decimal String(number=w494) -> (decimal integer string=w493:string)  [unwired: 1 in]
            }
            n353 = Build Array("Time", "Serial No.", "QR Code", "#1 Pressure", "#1 Leakage", "#2 Pressure", "#2 Leakage", "Result", "Part No." ("元素"), "Staff") -> (w437:string[])
            n354 = property on="A List" class="Tbl (严格)"("Number of Rows"=u32 1000 ("行数"), "Number of Columns"=u32 10 ("列数"), "Row Headers[]"=w438, "Column Headers[]"=w437, "Height"=u32 840 ("大小:高度"), "Width"=u32 900 ("大小:宽度")) -> ("Number of Rows"=w464:u32, "Number of Columns"=w461:u32, "Value"=w466:string[][])  [unwired: 2 in, 2 out]
            n355 = property on="B List" class="Tbl (严格)"("Number of Rows"=u32 1000 ("行数"), "Number of Columns"=u32 10 ("列数"), "Row Headers[]"=w438, "Column Headers[]"=w437, "Height"=u32 840 ("大小:高度"), "Width"=u32 900 ("大小:宽度")) -> ("Number of Rows"=w443:u32, "Number of Columns"=w446:u32, "Value"=w441:string[][])  [unwired: 2 in, 2 out]
            n356 = Array Size(array=w466) -> (size(s)=w465:i32[])
            n357 = Array Size(array=w441) -> (size(s)=w442:i32[])
            n358 = Index Array(array=w465) -> (element #1=w463:i32, element #2=w462:i32)  [unwired: 2 in]
            n359 = Index Array(array=w442) -> (element #1=w444:i32, element #2=w445:i32)  [unwired: 2 in]
            n360 = Max & Min(x=w464, y=w463) -> (max(x,y)=w460:u32)  [unwired: 1 out]
            n361 = Max & Min(x=w461, y=w462) -> (max(x,y)=w459:u32)  [unwired: 1 out]
            n362 = Max & Min(x=w443, y=w444) -> (max(x,y)=w447:u32)  [unwired: 1 out]
            n363 = Max & Min(x=w446, y=w445) -> (max(x,y)=w448:u32)  [unwired: 1 out]
            n364 = for {
              N: w460 -> [_]
              tunnel: w459 -> [w481]
              tunnel: u32 16448250 -> [w480]
              tunnel: u32 13816530 -> [w479]
              i -> [w478]
              n365 = for {
                N: w481 -> [_]
                tunnel: w478 -> [w492]
                tunnel: w480 -> [w486]
                tunnel: w479 -> [w485]
                tunnel: w478 -> [w483]
                i -> [w491]
                n366 = Quotient & Remainder(x=w483, y=u32 2) -> (x-y*floor(x/y)=w489:u32)  [unwired: 1 out]
                n367 = Equal?(x=w489, y=u32 0) -> (x = y?=w487:bool)
                n368 = Select(t=w486, s=w487, f=w485) -> (s? t:f=w484:u32)
                n369 = Bundle(w492, w491) -> (w482:cluster{i32, i32})  [unwired: 1 in]
                n370 = property on="A List" class="Tbl (严格)"("Active Cell"=w482, "Cell BG Color"=w484) -> ()  [unwired: 2 in, 2 out]
              }
            }
            n371 = for {
              N: w447 -> [_]
              tunnel: w448 -> [w500]
              tunnel: u32 16448250 -> [w499]
              tunnel: u32 13816530 -> [w498]
              i -> [w497]
              n372 = for {
                N: w500 -> [_]
                tunnel: w497 -> [w511]
                tunnel: w499 -> [w505]
                tunnel: w498 -> [w504]
                tunnel: w497 -> [w502]
                i -> [w510]
                n373 = Quotient & Remainder(x=w502, y=u32 2) -> (x-y*floor(x/y)=w508:u32)  [unwired: 1 out]
                n374 = Equal?(x=w508, y=u32 0) -> (x = y?=w506:bool)
                n375 = Select(t=w505, s=w506, f=w504) -> (s? t:f=w503:u32)
                n376 = Bundle(w511, w510) -> (w501:cluster{i32, i32})  [unwired: 1 in]
                n377 = property on="B List" class="Tbl (严格)"("Active Cell"=w501, "Cell BG Color"=w503) -> ()  [unwired: 2 in, 2 out]
              }
            }
          }
          frame 2 {
            n378 = for {
              N: 1000 -> [_]
              shift-right: [w569] -> _
              shift-left: _ -> [_]
              tunnel: [w568] -> w513 mode=indexing
              i -> [w570]
              n379 = Add(x=1, y=w570) -> (x+y=w569:i32)
              n380 = Number To Decimal String(number=w569) -> (decimal integer string=w568:string)  [unwired: 1 in]
            }
            n381 = Build Array("Heure", "Matricule", "Code QR", "#1 Pression", "#1 Fuite", "#2 Pression", "#2 Fuite", "Résultat", "N° de pièce" ("元素"), "Personnel") -> (w512:string[])
            n382 = property on="A List" class="Tbl (严格)"("Number of Rows"=u32 1000 ("行数"), "Number of Columns"=u32 10 ("列数"), "Row Headers[]"=w513, "Column Headers[]"=w512, "Height"=u32 840 ("大小:高度"), "Width"=u32 900 ("大小:宽度")) -> ("Number of Rows"=w539:u32, "Number of Columns"=w536:u32, "Value"=w541:string[][])  [unwired: 2 in, 2 out]
            n383 = property on="B List" class="Tbl (严格)"("Number of Rows"=u32 1000 ("行数"), "Number of Columns"=u32 10 ("列数"), "Row Headers[]"=w513, "Column Headers[]"=w512, "Height"=u32 840 ("大小:高度"), "Width"=u32 900 ("大小:宽度")) -> ("Number of Rows"=w518:u32, "Number of Columns"=w521:u32, "Value"=w516:string[][])  [unwired: 2 in, 2 out]
            n384 = Array Size(array=w541) -> (size(s)=w540:i32[])
            n385 = Array Size(array=w516) -> (size(s)=w517:i32[])
            n386 = Index Array(array=w540) -> (element #1=w538:i32, element #2=w537:i32)  [unwired: 2 in]
            n387 = Index Array(array=w517) -> (element #1=w519:i32, element #2=w520:i32)  [unwired: 2 in]
            n388 = Max & Min(x=w539, y=w538) -> (max(x,y)=w535:u32)  [unwired: 1 out]
            n389 = Max & Min(x=w536, y=w537) -> (max(x,y)=w534:u32)  [unwired: 1 out]
            n390 = Max & Min(x=w518, y=w519) -> (max(x,y)=w522:u32)  [unwired: 1 out]
            n391 = Max & Min(x=w521, y=w520) -> (max(x,y)=w523:u32)  [unwired: 1 out]
            n392 = for {
              N: w535 -> [_]
              tunnel: w534 -> [w556]
              tunnel: u32 16448250 -> [w555]
              tunnel: u32 13816530 -> [w554]
              i -> [w553]
              n393 = for {
                N: w556 -> [_]
                tunnel: w553 -> [w567]
                tunnel: w555 -> [w561]
                tunnel: w554 -> [w560]
                tunnel: w553 -> [w558]
                i -> [w566]
                n394 = Quotient & Remainder(x=w558, y=u32 2) -> (x-y*floor(x/y)=w564:u32)  [unwired: 1 out]
                n395 = Equal?(x=w564, y=u32 0) -> (x = y?=w562:bool)
                n396 = Select(t=w561, s=w562, f=w560) -> (s? t:f=w559:u32)
                n397 = Bundle(w567, w566) -> (w557:cluster{i32, i32})  [unwired: 1 in]
                n398 = property on="A List" class="Tbl (严格)"("Active Cell"=w557, "Cell BG Color"=w559) -> ()  [unwired: 2 in, 2 out]
              }
            }
            n399 = for {
              N: w522 -> [_]
              tunnel: w523 -> [w575]
              tunnel: u32 16448250 -> [w574]
              tunnel: u32 13816530 -> [w573]
              i -> [w572]
              n400 = for {
                N: w575 -> [_]
                tunnel: w572 -> [w586]
                tunnel: w574 -> [w580]
                tunnel: w573 -> [w579]
                tunnel: w572 -> [w577]
                i -> [w585]
                n401 = Quotient & Remainder(x=w577, y=u32 2) -> (x-y*floor(x/y)=w583:u32)  [unwired: 1 out]
                n402 = Equal?(x=w583, y=u32 0) -> (x = y?=w581:bool)
                n403 = Select(t=w580, s=w581, f=w579) -> (s? t:f=w578:u32)
                n404 = Bundle(w586, w585) -> (w576:cluster{i32, i32})  [unwired: 1 in]
                n405 = property on="B List" class="Tbl (严格)"("Active Cell"=w576, "Cell BG Color"=w578) -> ()  [unwired: 2 in, 2 out]
              }
            }
          }
        }
      }
      event "A Start Validation": Mouse Up {
        n406 = event-data() -> ()  [unwired: 1 in, 8 out]
        n407 = property on="Part No. A" class="Ring (严格)"() -> ("Value"=w587:u16)  [unwired: 2 in, 2 out]
        n408 = case shown="1, 默认" w587 {
          frame 1, Default {
          }
          frame 0 {
            n409 = One Button Dialog(message="请确认产品型号！" ("消息")) -> ()  [unwired: 1 in, 1 out]
          }
        }
      }
      event "B Start Validation": Mouse Up {
        n410 = event-data() -> ()  [unwired: 1 in, 8 out]
        n411 = property on="Part No. B" class="Ring (严格)"() -> ("Value"=w589:u16)  [unwired: 2 in, 2 out]
        n412 = case shown="1, 默认" w589 {
          frame 1, Default {
          }
          frame 0 {
            n413 = One Button Dialog(message="请确认产品型号！" ("消息")) -> ()  [unwired: 1 in, 1 out]
          }
        }
      }
    }
  }
  n414 = while {
    stop <- FALSE stop-if-true
    n415 = event shown="[0] \"Language\": 值改变" {
      selector: _ -> [_]
      dyn-events: _ -> [_]
      timeout: _ -> [_]
      event "Language": Value Change {
        n416 = event-data() -> ("NewVal"=w592:u16)  [unwired: 1 in, 5 out]
        n417 = case shown="0, 默认" w592 {
          frame 0, Default {
            n418 = property on="Single/Dual B" class="Bool (严格)"() -> ("Value"=w594:bool)  [unwired: 2 in, 2 out]
            n419 = property on="Single/Dual A" class="Bool (严格)"() -> ("Value"=w595:bool)  [unwired: 2 in, 2 out]
            n420 = for {
              N: 50 -> [_]
              shift-right: [w633] -> _
              shift-left: _ -> [_]
              tunnel: [w632] -> w608 mode=indexing
              i -> [w634]
              n421 = Add(x=1, y=w634) -> (x+y=w633:i32)
              n422 = Number To Decimal String(number=w633) -> (decimal integer string=w632:string)  [unwired: 1 in]
            }
            n423 = property on="保存确定" class="Bool"("BoolText.Text"="保存参数" ("布尔文本.文本")) -> ()  [unwired: 2 in, 2 out]
            n424 = case shown="真" w594 {
              frame True {
                n425 = property on="Single/Dual B" class="Bool (严格)"("BoolText.Text"="双腔测试" ("布尔文本.文本")) -> ()  [unwired: 2 in, 2 out]
              }
              frame False {
                n426 = property on="Single/Dual B" class="Bool (严格)"("BoolText.Text"="单腔测试" ("布尔文本.文本")) -> ()  [unwired: 2 in, 2 out]
              }
            }
            n427 = case shown="真" w595 {
              frame True {
                n428 = property on="Single/Dual A" class="Bool (严格)"("BoolText.Text"="双腔测试" ("布尔文本.文本")) -> ()  [unwired: 2 in, 2 out]
              }
              frame False {
                n429 = property on="Single/Dual A" class="Bool (严格)"("BoolText.Text"="单腔测试" ("布尔文本.文本")) -> ()  [unwired: 2 in, 2 out]
              }
            }
            n430 = Build Array("产品型号", "客户型号", "ATEQ程序号", "人员" ("元素")) -> (w610:string[])
            n431 = property on="参数设置/Setup/Coup monté" class="Tbl (严格)"("Row Headers[]"=w608, "Column Headers[]"=w610) -> ("Number of Rows"=w599:u32, "Number of Columns"=w598:u32, "Value"=w597:string[][])  [unwired: 2 in, 2 out]
            n432 = Array Size(array=w597) -> (size(s)=w606:i32[])
            n433 = Index Array(array=w606) -> (element #1=w605:i32, element #2=w604:i32)  [unwired: 2 in]
            n434 = Max & Min(x=w599, y=w605) -> (max(x,y)=w603:u32)  [unwired: 1 out]
            n435 = Max & Min(x=w598, y=w604) -> (max(x,y)=w602:u32)  [unwired: 1 out]
            n436 = for {
              N: w603 -> [_]
              tunnel: w602 -> [w620]
              tunnel: u32 16448250 -> [w619]
              tunnel: u32 13816530 -> [w618]
              i -> [w617]
              n437 = for {
                N: w620 -> [_]
                tunnel: w617 -> [w631]
                tunnel: w619 -> [w625]
                tunnel: w618 -> [w624]
                tunnel: w617 -> [w622]
                i -> [w630]
                n438 = Quotient & Remainder(x=w622, y=u32 2) -> (x-y*floor(x/y)=w628:u32)  [unwired: 1 out]
                n439 = Equal?(x=w628, y=u32 0) -> (x = y?=w626:bool)
                n440 = Select(t=w625, s=w626, f=w624) -> (s? t:f=w623:u32)
                n441 = Bundle(w631, w630) -> (w621:cluster{i32, i32})  [unwired: 1 in]
                n442 = property on="参数设置/Setup/Coup monté" class="Tbl (严格)"("Active Cell"=w621, "Cell BG Color"=w623) -> ()  [unwired: 2 in, 2 out]
              }
            }
          }
          frame 1 {
            n443 = property on="Single/Dual A" class="Bool (严格)"() -> ("Value"=w639:bool)  [unwired: 2 in, 2 out]
            n444 = property on="Single/Dual B" class="Bool (严格)"() -> ("Value"=w638:bool)  [unwired: 2 in, 2 out]
            n445 = for {
              N: 50 -> [_]
              shift-right: [w676] -> _
              shift-left: _ -> [_]
              tunnel: [w675] -> w652 mode=indexing
              i -> [w677]
              n446 = Add(x=1, y=w677) -> (x+y=w676:i32)
              n447 = Number To Decimal String(number=w676) -> (decimal integer string=w675:string)  [unwired: 1 in]
            }
            n448 = case shown="假" w639 {
              frame True {
                n449 = property on="Single/Dual A" class="Bool (严格)"("BoolText.Text"="Dual Tests" ("布尔文本.文本")) -> ()  [unwired: 2 in, 2 out]
              }
              frame False {
                n450 = property on="Single/Dual A" class="Bool (严格)"("BoolText.Text"="Single Test" ("布尔文本.文本")) -> ()  [unwired: 2 in, 2 out]
              }
            }
            n451 = case shown="真" w638 {
              frame True {
                n452 = property on="Single/Dual B" class="Bool (严格)"("BoolText.Text"="Dual Tests" ("布尔文本.文本")) -> ()  [unwired: 2 in, 2 out]
              }
              frame False {
                n453 = property on="Single/Dual B" class="Bool (严格)"("BoolText.Text"="Single Test" ("布尔文本.文本")) -> ()  [unwired: 2 in, 2 out]
              }
            }
            n454 = property on="保存确定" class="Bool"("BoolText.Text"="Save Parameters" ("布尔文本.文本")) -> ()  [unwired: 2 in, 2 out]
            n455 = Build Array("Part No.", "Customer No." ("元素"), "ATEQ No.", "Staff" ("元素")) -> (w654:string[])
            n456 = property on="参数设置/Setup/Coup monté" class="Tbl (严格)"("Row Headers[]"=w652, "Column Headers[]"=w654) -> ("Number of Rows"=w643:u32, "Number of Columns"=w642:u32, "Value"=w641:string[][])  [unwired: 2 in, 2 out]
            n457 = Array Size(array=w641) -> (size(s)=w650:i32[])
            n458 = Index Array(array=w650) -> (element #1=w649:i32, element #2=w648:i32)  [unwired: 2 in]
            n459 = Max & Min(x=w643, y=w649) -> (max(x,y)=w647:u32)  [unwired: 1 out]
            n460 = Max & Min(x=w642, y=w648) -> (max(x,y)=w646:u32)  [unwired: 1 out]
            n461 = for {
              N: w647 -> [_]
              tunnel: w646 -> [w663]
              tunnel: u32 16448250 -> [w662]
              tunnel: u32 13816530 -> [w661]
              i -> [w660]
              n462 = for {
                N: w663 -> [_]
                tunnel: w660 -> [w674]
                tunnel: w662 -> [w668]
                tunnel: w661 -> [w667]
                tunnel: w660 -> [w665]
                i -> [w673]
                n463 = Quotient & Remainder(x=w665, y=u32 2) -> (x-y*floor(x/y)=w671:u32)  [unwired: 1 out]
                n464 = Equal?(x=w671, y=u32 0) -> (x = y?=w669:bool)
                n465 = Select(t=w668, s=w669, f=w667) -> (s? t:f=w666:u32)
                n466 = Bundle(w674, w673) -> (w664:cluster{i32, i32})  [unwired: 1 in]
                n467 = property on="参数设置/Setup/Coup monté" class="Tbl (严格)"("Active Cell"=w664, "Cell BG Color"=w666) -> ()  [unwired: 2 in, 2 out]
              }
            }
          }
          frame 2 {
            w679 = "N° de client"  # N° de client
            n468 = property on="Single/Dual A" class="Bool (严格)"() -> ("Value"=w681:bool)  [unwired: 2 in, 2 out]
            n469 = property on="Single/Dual B" class="Bool (严格)"() -> ("Value"=w680:bool)  [unwired: 2 in, 2 out]
            n470 = for {
              N: 50 -> [_]
              shift-right: [w718] -> _
              shift-left: _ -> [_]
              tunnel: [w717] -> w693 mode=indexing
              i -> [w719]
              n471 = Add(x=1, y=w719) -> (x+y=w718:i32)
              n472 = Number To Decimal String(number=w718) -> (decimal integer string=w717:string)  [unwired: 1 in]
            }
            n473 = case shown="假" w681 {
              frame True {
                n474 = property on="Single/Dual A" class="Bool (严格)"("BoolText.Text"="Double Tests" ("布尔文本.文本")) -> ()  [unwired: 2 in, 2 out]
              }
              frame False {
                n475 = property on="Single/Dual A" class="Bool (严格)"("BoolText.Text"="Unique Test" ("布尔文本.文本")) -> ()  [unwired: 2 in, 2 out]
              }
            }
            n476 = case shown="真" w680 {
              frame True {
                n477 = property on="Single/Dual B" class="Bool (严格)"("BoolText.Text"="Double Tests" ("布尔文本.文本")) -> ()  [unwired: 2 in, 2 out]
              }
              frame False {
                n478 = property on="Single/Dual B" class="Bool (严格)"("BoolText.Text"="Unique Test" ("布尔文本.文本")) -> ()  [unwired: 2 in, 2 out]
              }
            }
            n479 = Build Array("N° de pièce", w679, "N° de ATEQ", "Personnel" ("元素")) -> (w695:string[])
            n480 = property on="参数设置/Setup/Coup monté" class="Tbl (严格)"("Row Headers[]"=w693, "Column Headers[]"=w695) -> ("Number of Rows"=w684:u32, "Number of Columns"=w683:u32, "Value"=w682:string[][])  [unwired: 2 in, 2 out]
            n481 = Array Size(array=w682) -> (size(s)=w691:i32[])
            n482 = Index Array(array=w691) -> (element #1=w690:i32, element #2=w689:i32)  [unwired: 2 in]
            n483 = Max & Min(x=w684, y=w690) -> (max(x,y)=w688:u32)  [unwired: 1 out]
            n484 = Max & Min(x=w683, y=w689) -> (max(x,y)=w687:u32)  [unwired: 1 out]
            n485 = for {
              N: w688 -> [_]
              tunnel: w687 -> [w705]
              tunnel: u32 16448250 -> [w704]
              tunnel: u32 13816530 -> [w703]
              i -> [w702]
              n486 = for {
                N: w705 -> [_]
                tunnel: w702 -> [w716]
                tunnel: w704 -> [w710]
                tunnel: w703 -> [w709]
                tunnel: w702 -> [w707]
                i -> [w715]
                n487 = Quotient & Remainder(x=w707, y=u32 2) -> (x-y*floor(x/y)=w713:u32)  [unwired: 1 out]
                n488 = Equal?(x=w713, y=u32 0) -> (x = y?=w711:bool)
                n489 = Select(t=w710, s=w711, f=w709) -> (s? t:f=w708:u32)
                n490 = Bundle(w716, w715) -> (w706:cluster{i32, i32})  [unwired: 1 in]
                n491 = property on="参数设置/Setup/Coup monté" class="Tbl (严格)"("Active Cell"=w706, "Cell BG Color"=w708) -> ()  [unwired: 2 in, 2 out]
              }
            }
          }
        }
      }
    }
  }
  n492 = while {
    stop <- FALSE stop-if-true
    n493 = property on="打印标签路径B/Print label path B/Imprimer le chemin d’accès de l’étiquette B" class="Path"() -> ("Value"=w735:path)  [unwired: 2 in, 2 out]
    n494 = property on="打印标签路径A/Print label path A/Imprimer le chemin d’accès de l’étiquette A" class="Path"() -> ("Value"=w733:path)  [unwired: 2 in, 2 out]
    n495 = Wait (ms)(milliseconds to wait=u32 100 ("等待时间（毫秒）")) -> ()  [unwired: 1 out]
    n496 = Path To String(path=w735) -> (string=w736:string)
    n497 = Path To String(path=w733) -> (string=w734:string)
    n498 = Match Pattern(string=w736, regular expression="\\") -> (after substring=w726:string)  [unwired: 1 in, 3 out]
    n499 = Match Pattern(string=w734, regular expression="\\") -> (after substring=w727:string)  [unwired: 1 in, 3 out]
    n500 = Concatenate Strings("BarTender Enterprise Automation - [" ("lpszWindowName"), w726, "]" ("lpszWindowName")) -> (w732:string)
    n501 = Concatenate Strings("BarTender Enterprise Automation - [" ("lpszWindowName"), w727, "]" ("lpszWindowName")) -> (w731:string)
    n502 = call "Move Window to Bottom v1.vi"("window name (\"\")"=w732) -> ("error out"=→"error out 3":errorcluster)  [unwired: 5 in, 1 out]
    n503 = call "Move Window to Bottom v1.vi"("window name (\"\")"=w731) -> ("error out"=→"error out 2":errorcluster)  [unwired: 5 in, 1 out]
  }
  n504 = while {
    stop <- FALSE stop-if-true
    n505 = event shown="[3] \"Download A\": 鼠标按下" {
      selector: _ -> [_ _ _ _ _]
      dyn-events: _ -> [_ _ _ _ _]
      timeout: _ -> [_ _ _ _ _]
      event Timeout {
        n506 = event-data() -> ()  [unwired: 1 in, 3 out]
      }
      event "Search A": Mouse Down {
        n507 = event-data() -> ()  [unwired: 1 in, 8 out]
        n508 = property on="Result A" class="Ring (严格)"() -> ("Strings []"=w744:string[], "Value"=w743:u16)  [unwired: 2 in, 2 out]
        n509 = Index Array(array=w744, index=w743) -> (element=w742:string)
        n510 = call "数据查询.vi"("Result"=w742, "2D_Code"="2D Code A", "结束时间"="Finish Time A", "开始时间"="Start Time A") -> ("Data"=w741:string[][])  [unwired: 7 in]
        n511 = property on="A List Search" class="Tbl (严格)"("Value"=w741) -> ()  [unwired: 2 in, 2 out]
      }
      event "Search B": Mouse Down {
        n512 = event-data() -> ()  [unwired: 1 in, 8 out]
        n513 = property on="Result B" class="Ring (严格)"() -> ("Strings []"=w754:string[], "Value"=w753:u16)  [unwired: 2 in, 2 out]
        n514 = Index Array(array=w754, index=w753) -> (element=w752:string)
        n515 = call "数据查询B.vi"("Result"=w752, "2D_Code"="2D Code B", "结束时间"="Finish Time B", "开始时间"="Start Time B") -> ("Data"=w751:string[][])  [unwired: 7 in]
        n516 = property on="B List Search" class="Tbl (严格)"("Value"=w751) -> ()  [unwired: 2 in, 2 out]
      }
      event "Download A": Mouse Down {
        n517 = event-data() -> ()  [unwired: 1 in, 8 out]
        n518 = property on="A List Search" class="Tbl (严格)"() -> ("Value"=w755:string[][])  [unwired: 2 in, 2 out]
        n519 = call-poly <vilib>:"Write To Spreadsheet File.vi"("2D data"=w755) -> ()  [unwired: 7 in, 1 out]
      }
      event "Download B": Mouse Down {
        n520 = event-data() -> ()  [unwired: 1 in, 8 out]
        n521 = property on="B List Search" class="Tbl (严格)"() -> ("Value"=w756:string[][])  [unwired: 2 in, 2 out]
        n522 = call-poly <vilib>:"Write To Spreadsheet File.vi"("2D data"=w756) -> ()  [unwired: 7 in, 1 out]
      }
    }
    n523 = Wait (ms)(milliseconds to wait=u32 100 ("等待时间（毫秒）")) -> ()  [unwired: 1 out]
  }
  n524 = flat-sequence {
    frame #0 {
      w757 = u16 2 ("合格状态左")
      w759 = ""
      w766 = FALSE
      w772 = "1"
      n525 = call "数据库读取.vi"() -> ("当日合格数"=w770:i32, "当天总数"=w769:i32, "Data"=w783:string[][])  [unwired: 9 in]
      n526 = call "数据库读取B.vi"() -> ("当日合格数"=w768:i32, "当天总数"=w767:i32, "Data"=w771:string[][])  [unwired: 9 in]
      n527 = Build Array("", "OK", "NG") -> (w774:string[])
      n528 = Initialize Array("", 50 ("维数大小"), 4 ("维数大小")) -> (w775:string[][])
      n529 = Initialize Array("", 1000 ("维数大小"), 25 ("维数大小")) -> (w773:string[][])
      n530 = property on="B List" class="Tbl (严格)"("Value"=w771) -> ()  [unwired: 2 in, 2 out]
      n531 = local write "Total Today B"(w767) -> ()
      n532 = local write "OK Today B"(w768) -> ()
      n533 = local write "参数设置/Setup/Coup monté"(w775) -> ()
      n534 = property on="Result B" class="Ring (严格)"("Strings []"=w774) -> ()  [unwired: 2 in, 2 out]
      n535 = property on="Result A" class="Ring (严格)"("Strings []"=w774) -> ()  [unwired: 2 in, 2 out]
      n536 = property on="读取程序号A" class="Bool (严格)"("Value"=FALSE ("读取程序号A")) -> ()  [unwired: 2 in, 2 out]
      n537 = property on="A List" class="Tbl (严格)"("Value"=w783) -> ()  [unwired: 2 in, 2 out]
      n538 = local write "Total Today A"(w769) -> ()
      n539 = local write "OK Today A"(w770) -> ()
      n540 = property on="B List Search" class="Tbl (严格)"("Value"=w773) -> ()  [unwired: 2 in, 2 out]
      n541 = property on="A List Search" class="Tbl (严格)"("Value"=w773) -> ()  [unwired: 2 in, 2 out]
      n542 = local write "合格状态右"(w757) -> ()
      n543 = local write "合格状态左"(w757) -> ()
      n544 = local write "2D Code_B"(w759) -> ()
      n545 = local write "2D Code_A"(w759) -> ()
      n546 = local write "scan A"(w766) -> ()
      n547 = local write "scan B"(w766) -> ()
      n548 = local write "ATEQ No. B"(w772) -> ()
      n549 = local write "ATEQ No. A"(w772) -> ()
      n550 = Build Array("中文", "English", "Francais") -> (w781:string[])
      n551 = TCP Open Connection(address="192.168.2.2" ("IP"), remote port or service name=u16 9004 ("Port"), timeout ms (60000)=1000 ("超时毫秒(60000)")) -> (connection ID=w763:refnum<k5>, error out=w764:errorcluster)  [unwired: 2 in]
      n552 = property on="Language" class="Ring (严格)"("Strings []"=w781) -> ()  [unwired: 2 in, 2 out]
      n553 = TCP Close Connection(connection ID=w763, error in (no error)=w764) -> (error out=→"错误输出  2":errorcluster)  [unwired: 1 in, 1 out]
      n554 = local write "密码"("") -> ()
    }
    frame #1 {
      w833 = T2."Enabled" ("禁用")
      w834 = FALSE
      w791 = T2."Disabled and Grayed Out" ("禁用")
      w839 = FALSE
      w838 = TRUE ("校准时间到")
      n555 = disable-structure shown="禁用" {
        frame Disabled {
          n556 = call "显示对话框信息2"() -> ("OK"=w876:bool)  [unwired: 10 in, 1 out]
          n557 = case shown="真" w876 {
            frame False {
            }
            frame True {
              n558 = property on="选项卡控件" class="TabCtl (严格)"("Value"=T1."测试/Main/Principale" ("选项卡控件")) -> ()  [unwired: 2 in, 2 out]
            }
          }
        }
        frame Enabled {
        }
      }
      n559 = property on="Part No. B" class="Ring (严格)"("DisabledEnum"=w833) -> ()  [unwired: 2 in, 2 out]
      n560 = property on="Staff A" class="Ring (严格)"("DisabledEnum"=w833) -> ()  [unwired: 2 in, 2 out]
      n561 = property on="Staff B" class="Ring (严格)"("DisabledEnum"=w833) -> ()  [unwired: 2 in, 2 out]
      n562 = property on="Part No. A" class="Ring (严格)"("DisabledEnum"=w833) -> ()  [unwired: 2 in, 2 out]
      n563 = property on="A Cancel Validation" class="Bool"("DisabledEnum"=w791) -> ()  [unwired: 2 in, 2 out]
      n564 = property on="B Cancel Validation" class="Bool"("DisabledEnum"=w791) -> ()  [unwired: 2 in, 2 out]
      n565 = property on="B Cancel Validation" class="Bool"("Visible"=w834) -> ()  [unwired: 2 in, 2 out]
      n566 = property on="A Cancel Validation" class="Bool"("Visible"=w834) -> ()  [unwired: 2 in, 2 out]
      n567 = property on="选项卡控件" class="TabCtl (严格)"("Value"=T1."测试/Main/Principale" ("选项卡控件")) -> ()  [unwired: 2 in, 2 out]
      n568 = local write "B NG Sample Req.（1st)"(w839) -> ()
      n569 = local write "B OK Sample Req. (2nd)"(w839) -> ()
      n570 = local write "A OK Sample Req. (2nd)"(w839) -> ()
      n571 = local write "A NG Sample Req.（1st)"(w839) -> ()
      n572 = for {
        N: 1000 -> [_]
        shift-right: [w858] -> _
        shift-left: _ -> [_]
        tunnel: [w857] -> w831 mode=indexing
        i -> [w859]
        n573 = Add(x=1, y=w859) -> (x+y=w858:i32)
        n574 = Number To Decimal String(number=w858) -> (decimal integer string=w857:string)  [unwired: 1 in]
      }
      n575 = local write "B Cal. Time"(w838) -> ()
      n576 = local write "A Cal. Time"(w838) -> ()
      n577 = Build Array("管理员", "作业员") -> (w837:string[])
      n578 = property on="参数设置/Setup/Coup monté" class="Tbl (严格)"("DisabledEnum"=w791) -> ()  [unwired: 2 in, 2 out]
      n579 = property on="打印标签路径A/Print label path A/Imprimer le chemin d’accès de l’étiquette A" class="Path"("DisabledEnum"=w791) -> ()  [unwired: 2 in, 2 out]
      n580 = property on="Calitration Period (Hours)" class="AbsTime (严格)"("DisabledEnum"=w791) -> ()  [unwired: 2 in, 2 out]
      n581 = property on="登录" class="Ring (严格)"("Strings []"=w837) -> ()  [unwired: 2 in, 2 out]
      n582 = property on="ATEQ F620 A (Restart Software to Active)" class="VISAName"("DisabledEnum"=w791) -> ()  [unwired: 2 in, 2 out]
      n583 = property on="ATEQ F620 B (Restart Software to Active)" class="VISAName"("DisabledEnum"=w791) -> ()  [unwired: 2 in, 2 out]
      n584 = Build Array("Heure", "Matricule", "Code QR", "#1 Pression", "#1 Fuite", "#2 Pression", "#2 Fuite", "Résultat", "N° de pièce" ("元素"), "Personnel") -> (w832:string[])
      n585 = property on="A List Search" class="Tbl (严格)"("Number of Rows"=u32 1000 ("行数"), "Number of Columns"=u32 10 ("列数"), "Row Headers[]"=w831, "Column Headers[]"=w832, "Height"=u32 840 ("大小:高度"), "Width"=u32 900 ("大小:宽度")) -> ("Number of Rows"=w805:u32, "Number of Columns"=w808:u32, "Value"=w803:string[][])  [unwired: 2 in, 2 out]
      n586 = property on="B List Search" class="Tbl (严格)"("Number of Rows"=u32 1000 ("行数"), "Number of Columns"=u32 10 ("列数"), "Row Headers[]"=w831, "Column Headers[]"=w832, "Height"=u32 840 ("大小:高度"), "Width"=u32 900 ("大小:宽度")) -> ("Number of Rows"=w826:u32, "Number of Columns"=w823:u32, "Value"=w828:string[][])  [unwired: 2 in, 2 out]
      n587 = Array Size(array=w803) -> (size(s)=w804:i32[])
      n588 = Array Size(array=w828) -> (size(s)=w827:i32[])
      n589 = Index Array(array=w804) -> (element #1=w806:i32, element #2=w807:i32)  [unwired: 2 in]
      n590 = Index Array(array=w827) -> (element #1=w825:i32, element #2=w824:i32)  [unwired: 2 in]
      n591 = Max & Min(x=w805, y=w806) -> (max(x,y)=w809:u32)  [unwired: 1 out]
      n592 = Max & Min(x=w808, y=w807) -> (max(x,y)=w810:u32)  [unwired: 1 out]
      n593 = Max & Min(x=w826, y=w825) -> (max(x,y)=w822:u32)  [unwired: 1 out]
      n594 = Max & Min(x=w823, y=w824) -> (max(x,y)=w821:u32)  [unwired: 1 out]
      n595 = for {
        N: w809 -> [_]
        tunnel: w810 -> [w845]
        tunnel: u32 16448250 -> [w844]
        tunnel: u32 13816530 -> [w843]
        i -> [w842]
        n596 = for {
          N: w845 -> [_]
          tunnel: w842 -> [w856]
          tunnel: w844 -> [w850]
          tunnel: w843 -> [w849]
          tunnel: w842 -> [w847]
          i -> [w855]
          n597 = Quotient & Remainder(x=w847, y=u32 2) -> (x-y*floor(x/y)=w853:u32)  [unwired: 1 out]
          n598 = Equal?(x=w853, y=u32 0) -> (x = y?=w851:bool)
          n599 = Select(t=w850, s=w851, f=w849) -> (s? t:f=w848:u32)
          n600 = Bundle(w856, w855) -> (w846:cluster{i32, i32})  [unwired: 1 in]
          n601 = property on="A List Search" class="Tbl (严格)"("Active Cell"=w846, "Cell BG Color"=w848) -> ()  [unwired: 2 in, 2 out]
        }
      }
      n602 = for {
        N: w822 -> [_]
        tunnel: w821 -> [w864]
        tunnel: u32 16448250 -> [w863]
        tunnel: u32 13816530 -> [w862]
        i -> [w861]
        n603 = for {
          N: w864 -> [_]
          tunnel: w861 -> [w875]
          tunnel: w863 -> [w869]
          tunnel: w862 -> [w868]
          tunnel: w861 -> [w866]
          i -> [w874]
          n604 = Quotient & Remainder(x=w866, y=u32 2) -> (x-y*floor(x/y)=w872:u32)  [unwired: 1 out]
          n605 = Equal?(x=w872, y=u32 0) -> (x = y?=w870:bool)
          n606 = Select(t=w869, s=w870, f=w868) -> (s? t:f=w867:u32)
          n607 = Bundle(w875, w874) -> (w865:cluster{i32, i32})  [unwired: 1 in]
          n608 = property on="B List Search" class="Tbl (严格)"("Active Cell"=w865, "Cell BG Color"=w867) -> ()  [unwired: 2 in, 2 out]
        }
      }
      n609 = Wait (ms)(milliseconds to wait=u32 5000 ("等待时间（毫秒）")) -> ()  [unwired: 1 out]
    }
    frame #2 {
      w879 = u16 0 ("合格次数")
      w878 = u16 0 ("合格次数")
      n610 = local write "检测次数B"(w879) -> ()
      n611 = local write "合格次数B"(w879) -> ()
      n612 = local write "合格次数A"(w878) -> ()
      n613 = local write "检测次数A"(w878) -> ()
    }
  }
  n614 = while {
    stop <- FALSE stop-if-true
    n615 = event shown="[1] \"保存确定\": 鼠标释放" {
      selector: _ -> [_ _]
      dyn-events: _ -> [_ _]
      timeout: _ -> [_ _]
      event Timeout {
        n616 = event-data() -> ()  [unwired: 1 in, 3 out]
      }
      event "保存确定": Mouse Up {
        w886 = "Setup" ("section")
        n617 = event-data() -> ()  [unwired: 1 in, 6 out]
        n618 = call <vilib>:"Open Config Data.vi"("create file if necessary (T)"=TRUE, "configuration file path"=path "D:/data/Setup.ini") -> ("error out"=w905:errorcluster, "refnum"=w902:T3)  [unwired: 7 in, 1 out]
        n619 = for {
          N: 50 -> [_]
          tunnel: w902 -> [w980]
          tunnel: [w976] -> w884
          tunnel: w905 -> [w975]
          tunnel: [w974] -> w883
          tunnel: [w968] -> w911 mode=indexing
          i -> [w973]
          n620 = property on="参数设置/Setup/Coup monté" class="Tbl (严格)"() -> ("Value"=w978:string[][])  [unwired: 2 in, 2 out]
          n621 = Increment(x=w973) -> (x+1=w971:i32)
          n622 = Number To Decimal String(number=w971) -> (decimal integer string=w970:string)  [unwired: 1 in]
          n623 = Concatenate Strings("产品型号" ("字符串"), w970) -> (w969:string)
          n624 = Index Array(array=w978, index (row)=w973, index (col)=0 ("Column")) -> (element=w968:string)
          n625 = call-poly <vilib>:"Write Key.vi"("section"="Setup", "error in (no error)"=w975, "value"=w968, "key"=w969, "refnum"=w980) -> ("error out"=w974:errorcluster, "refnum out"=w976:T3)  [unwired: 4 in, 1 out]
        }
        n626 = property on="Part No. A" class="Ring (严格)"("Strings []"=w911) -> ()  [unwired: 2 in, 2 out]
        n627 = property on="Part No. B" class="Ring (严格)"("Strings []"=w911) -> ()  [unwired: 2 in, 2 out]
        n628 = for {
          N: 50 -> [_]
          tunnel: w884 -> [w941]
          tunnel: [w937] -> w882
          tunnel: w883 -> [w936]
          tunnel: [w935] -> w881
          tunnel: [w929] -> _ mode=indexing
          i -> [w934]
          n629 = property on="参数设置/Setup/Coup monté" class="Tbl (严格)"() -> ("Value"=w939:string[][])  [unwired: 2 in, 2 out]
          n630 = Increment(x=w934) -> (x+1=w932:i32)
          n631 = Number To Decimal String(number=w932) -> (decimal integer string=w931:string)  [unwired: 1 in]
          n632 = Concatenate Strings("客户型号" ("字符串"), w931) -> (w930:string)
          n633 = Index Array(array=w939, index (row)=w934, index (col)=1 ("Column")) -> (element=w929:string)
          n634 = call-poly <vilib>:"Write Key.vi"("section"="Setup", "error in (no error)"=w936, "value"=w929, "key"=w930, "refnum"=w941) -> ("error out"=w935:errorcluster, "refnum out"=w937:T3)  [unwired: 4 in, 1 out]
        }
        n635 = for {
          N: 50 -> [_]
          tunnel: w882 -> [w967]
          tunnel: [w963] -> w908
          tunnel: [w962] -> w909
          tunnel: w881 -> [w955]
          i -> [w961]
          n636 = property on="参数设置/Setup/Coup monté" class="Tbl (严格)"() -> ("Value"=w965:string[][])  [unwired: 2 in, 2 out]
          n637 = Increment(x=w961) -> (x+1=w959:i32)
          n638 = Number To Decimal String(number=w959) -> (decimal integer string=w958:string)  [unwired: 1 in]
          n639 = Concatenate Strings("ATEQ程序号" ("字符串"), w958) -> (w957:string)
          n640 = Index Array(array=w965, index (row)=w961, index (col)=2 ("Column")) -> (element=w956:string)
          n641 = call-poly <vilib>:"Write Key.vi"("section"="Setup", "error in (no error)"=w955, "value"=w956, "key"=w957, "refnum"=w967) -> ("error out"=w962:errorcluster, "refnum out"=w963:T3)  [unwired: 4 in, 1 out]
        }
        n642 = for {
          N: 50 -> [_]
          tunnel: w908 -> [w954]
          tunnel: [w950] -> w920
          tunnel: w909 -> [w949]
          tunnel: [w948] -> w921
          tunnel: [w942] -> w910 mode=indexing
          i -> [w947]
          n643 = property on="参数设置/Setup/Coup monté" class="Tbl (严格)"() -> ("Value"=w952:string[][])  [unwired: 2 in, 2 out]
          n644 = Increment(x=w947) -> (x+1=w945:i32)
          n645 = Number To Decimal String(number=w945) -> (decimal integer string=w944:string)  [unwired: 1 in]
          n646 = Concatenate Strings("人员" ("字符串"), w944) -> (w943:string)
          n647 = Index Array(array=w952, index (row)=w947, index (col)=3 ("Column")) -> (element=w942:string)
          n648 = call-poly <vilib>:"Write Key.vi"("section"="Setup", "error in (no error)"=w949, "value"=w942, "key"=w943, "refnum"=w954) -> ("error out"=w948:errorcluster, "refnum out"=w950:T3)  [unwired: 4 in, 1 out]
        }
        n649 = property on="打印标签路径B/Print label path B/Imprimer le chemin d’accès de l’étiquette B" class="Path"() -> ("Label.Text"=w912:string)  [unwired: 2 in, 2 out]
        n650 = property on="打印标签路径B/Print label path B/Imprimer le chemin d’accès de l’étiquette B" class="Path"() -> ("Value"=w918:path)  [unwired: 2 in, 2 out]
        n651 = property on="ATEQ F620 A (Restart Software to Active)" class="VISAName"() -> ("Label.Text"=w915:string)  [unwired: 2 in, 2 out]
        n652 = property on="ATEQ F620 A (Restart Software to Active)" class="VISAName"() -> ("Value"=w917:refnum<visa-resource-name>)  [unwired: 2 in, 2 out]
        n653 = property on="打印标签路径A/Print label path A/Imprimer le chemin d’accès de l’étiquette A" class="Path"() -> ("Label.Text"=w913:string)  [unwired: 2 in, 2 out]
        n654 = property on="打印标签路径A/Print label path A/Imprimer le chemin d’accès de l’étiquette A" class="Path"() -> ("Value"=w919:path)  [unwired: 2 in, 2 out]
        n655 = property on="Staff A" class="Ring (严格)"("Strings []"=w910) -> ()  [unwired: 2 in, 2 out]
        n656 = property on="Staff B" class="Ring (严格)"("Strings []"=w910) -> ()  [unwired: 2 in, 2 out]
        n657 = property on="ATEQ F620 B (Restart Software to Active)" class="VISAName"() -> ("Label.Text"=w914:string)  [unwired: 2 in, 2 out]
        n658 = property on="ATEQ F620 B (Restart Software to Active)" class="VISAName"() -> ("Value"=w928:refnum<visa-resource-name>)  [unwired: 2 in, 2 out]
        n659 = call-poly <vilib>:"Write Key.vi"("section"="Setup", "error in (no error)"=w921, "value"=w917, "key"=w915, "refnum"=w920) -> ("error out"=w923:errorcluster, "refnum out"=w922:T3)  [unwired: 4 in, 1 out]
        n660 = call-poly <vilib>:"Write Key.vi"("section"=w886, "error in (no error)"=w923, "value"=w918, "key"=w912, "refnum"=w922) -> ("error out"=w925:errorcluster, "refnum out"=w924:T3)  [unwired: 4 in, 1 out]
        n661 = call-poly <vilib>:"Write Key.vi"("section"=w886, "error in (no error)"=w925, "value"=w919, "key"=w913, "refnum"=w924) -> ("error out"=w927:errorcluster, "refnum out"=w926:T3)  [unwired: 4 in, 1 out]
        n662 = property on="Calitration Period (Hours)" class="AbsTime (严格)"() -> ("Label.Text"=w892:string, "NumText.Text"=w891:string)  [unwired: 2 in, 2 out]
        n663 = call-poly <vilib>:"Write Key.vi"("section"=w886, "error in (no error)"=w927, "value"=w928, "key"=w914, "refnum"=w926) -> ("error out"=w896:errorcluster, "refnum out"=w900:T3)  [unwired: 4 in, 1 out]
        n664 = property on="2nd Shift" class="AbsTime (严格)"() -> ("Label.Text"=w890:string, "NumText.Text"=w889:string)  [unwired: 2 in, 2 out]
        n665 = call-poly <vilib>:"Write Key.vi"("section"=w886, "error in (no error)"=w896, "value"=w891, "key"=w892, "refnum"=w900) -> ("error out"=w895:errorcluster, "refnum out"=w899:T3)  [unwired: 4 in, 1 out]
        n666 = property on="3th Shift" class="AbsTime (严格)"() -> ("Label.Text"=w888:string, "NumText.Text"=w887:string)  [unwired: 2 in, 2 out]
        n667 = call-poly <vilib>:"Write Key.vi"("section"=w886, "error in (no error)"=w895, "value"=w889, "key"=w890, "refnum"=w899) -> ("error out"=w894:errorcluster, "refnum out"=w898:T3)  [unwired: 4 in, 1 out]
        n668 = call-poly <vilib>:"Write Key.vi"("section"=w886, "error in (no error)"=w894, "value"=w887, "key"=w888, "refnum"=w898) -> ("error out"=w893:errorcluster, "refnum out"=w897:T3)  [unwired: 4 in, 1 out]
        n669 = call <vilib>:"Close Config Data.vi"("error in (no error)"=w893, "refnum"=w897) -> ()  [unwired: 8 in, 2 out]
      }
    }
  }
  n670 = while {
    i -> [w982]
    stop <- FALSE stop-if-true
    n671 = local read "Single/Dual B"() -> (w985:bool)
    n672 = Wait (ms)(milliseconds to wait=u32 250 ("等待时间（毫秒）")) -> ()  [unwired: 1 out]
    n673 = case shown="真" "B启动信号" {
      frame False {
      }
      frame True {
        n674 = local write "2D Code_B"("") -> ()
      }
    }
    n675 = local read "B结果信号"() -> (w983:bool)
    n676 = case shown="1" "合格状态右" {
      tunnel: w983 -> [w989 _ w1370]
      tunnel: w985 -> [_ w997 _]
      tunnel: w985 -> [_ w996 _]
      frame 0 {
        n677 = case shown="真" w989 {
          frame False {
          }
          frame True {
            n678 = local write "合格状态右"(1.0 ("合格状态")) -> ()
          }
        }
      }
      frame 1 {
        n679 = local read "B NG Sample Req.（1st)"() -> (w992:bool)
        n680 = local read "B OK Sample Req. (2nd)"() -> (w993:bool)
        n681 = local read "B Cal. Time"() -> (w995:bool)
        n682 = Or(x=w992, y=w993) -> (x .or. y?=w994:bool)
        n683 = And(x=w995, y=w994) -> (x .and. y?=w991:bool)
        n684 = case shown="假" w991 {
          tunnel: w997 -> [w999 w1173]
          tunnel: w996 -> [w998 w1172]
          frame False {
            n685 = flat-sequence {
              tunnel: [w1006] -> w1004
              tunnel: [w1007] -> w1003
              tunnel: w999 -> [w1007]
              tunnel: w998 -> [w1006]
              tunnel: [w1009] -> w1002
              tunnel: [w1014] -> w1001
              tunnel: w1004 -> [w1014]
              tunnel: [w1013] -> w1000
              tunnel: w1003 -> [w1013]
              tunnel: w1002 -> [w1037]
              tunnel: w1001 -> [w1035]
              tunnel: w1000 -> [w1034]
              frame #0 {
                n686 = local read "检测次数B"() -> (w1005:u16)
                n687 = Increment(x=w1005) -> (x+1=w1008:u16)
                n688 = local write "检测次数B"(w1008) -> ()
              }
              frame #1 {
                n689 = local read "合格 2"() -> (w1010:bool)
                n690 = property on="PressureUnit 2" class="Ring (严格)"() -> ("Value"=w1016:u16)  [unwired: 2 in, 2 out]
                n691 = local read "结果压力 B"() -> (w1012:dbl)
                n692 = property on="LeakUnit 2" class="Ring (严格)"() -> ("Value"=w1015:u16)  [unwired: 2 in, 2 out]
                n693 = Wait (ms)(milliseconds to wait=u32 2000 ("等待时间（毫秒）")) -> ()  [unwired: 1 out]
                n694 = case shown="1000" w1015 {
                  frame 0, Default {
                  }
                  frame 1000 {
                    n695 = local write "泄漏单位 2"("cm3/min" ("压力单位")) -> ()
                  }
                  frame 2000 {
                    n696 = local write "泄漏单位 2"("ml/h" ("压力单位")) -> ()
                  }
                  frame 6000 {
                    "泄漏单位 2" <- "pa"
                  }
                  frame 7000 {
                    n697 = local write "泄漏单位 2"("pa") -> ()
                  }
                  frame 8000 {
                    n698 = local write "泄漏单位 2"("pa/s" ("泄漏单位")) -> ()
                  }
                  frame 9000 {
                    n699 = local write "泄漏单位 2"("pa/s" ("泄漏单位")) -> ()
                  }
                  frame 51000 {
                    n700 = local write "泄漏单位 2"("ml/min" ("压力单位")) -> ()
                  }
                }
                n701 = case shown="15000" w1016 {
                  frame 0, Default {
                  }
                  frame 11000 {
                    n702 = local write "压力单位 2"("Bar" ("压力单位")) -> ()
                  }
                  frame 12000 {
                    n703 = local write "压力单位 2"("Kpa" ("压力单位")) -> ()
                  }
                  frame 13000 {
                    n704 = local write "压力单位 2"("Psi" ("压力单位")) -> ()
                  }
                  frame 14000 {
                    n705 = local write "压力单位 2"("mbar" ("压力单位")) -> ()
                  }
                  frame 15000 {
                    n706 = local write "压力单位 2"("Mpa") -> ()
                  }
                }
                n707 = Not Equal To 0?(x=w1012) -> (x != 0?=w1011:bool)
                n708 = And(x=w1011, y=w1010) -> (x .and. y?=w1009:bool)
                n709 = case shown="假" w1009 {
                  frame False {
                    n710 = local write "结果 2"("NG" ("结果")) -> ()
                  }
                  frame True {
                    n711 = local read "合格次数B"() -> (w1032:u16)
                    n712 = local write "结果 2"("OK" ("结果")) -> ()
                    n713 = Increment(x=w1032) -> (x+1=w1033:u16)
                    n714 = local write "合格次数B"(w1033) -> ()
                  }
                }
              }
              frame #2 {
                n715 = local read "检测次数B"() -> (w1036:u16)
                n716 = case shown="1" w1036 {
                  tunnel: w1037 -> [_ w1045 w1124]
                  tunnel: w1035 -> [_ w1043 _]
                  tunnel: w1034 -> [_ w1042 _]
                  frame 0, Default {
                  }
                  frame 1 {
                    n717 = flat-sequence {
                      tunnel: [w1061] -> w1041
                      tunnel: w1045 -> [w1061]
                      tunnel: [w1048] -> w1039
                      tunnel: w1041 -> [w1067]
                      tunnel: [w1067] -> w1040
                      tunnel: w1039 -> [w1063]
                      tunnel: [w1063] -> w1038
                      tunnel: w1040 -> [w1083]
                      tunnel: [w1081] -> w1044
                      tunnel: w1043 -> [w1082]
                      tunnel: w1042 -> [w1081]
                      tunnel: w1038 -> [w1070]
                      tunnel: w1044 -> [w1122]
                      frame #0 {
                        w1056 = TRUE  # 忽略大小写？(F)
                        w1055 = TRUE  # 替换全部？(F)
                        w1054 = "0"  # 替换字符串("")
                        w1051 = i16 4  # 宽度(-)
                        n718 = call "数据库读取B.vi"() -> ("当天总数"=w1047:i32)  [unwired: 9 in, 2 out]
                        n719 = Increment(x=w1047) -> (x+1=w1046:i32)
                        n720 = Number To Decimal String "数值至十进制数字符串转换"(number=w1046, width (-)=w1051) -> (decimal integer string=w1052:string)
                        n721 = call <vilib>:"Space Constant.vi"() -> ("String"=w1053:string)
                        n722 = property on="参数设置/Setup/Coup monté" class="Tbl (严格)"() -> ("Value"=w1059:string[][])  [unwired: 2 in, 2 out]
                        n723 = Search and Replace String "搜索替换字符串"(replace all?=w1055, case sensitive?=w1056, input string=w1052, search string=w1053, replace string=w1054) -> (result string=w1049:string)  [unwired: 3 in, 3 out]
                        n724 = property on="Part No. B" class="Ring (严格)" props=["Strings []", "Value"]() -> ("Value"=w1058:u16)  [unwired: 2 in, 3 out]
                        n725 = Index Array "索引数组"(array=w1059, index (row)=w1058, index (col)=0 ("禁用的索引 (列)")) -> (element=w1048:string)
                        n726 = Write to Text File "写入文本文件"(file (use dialog)=path "d:/data/序列号B.txt" ("文件（使用对话框）"), text=w1049) -> ()  [unwired: 2 in, 3 out]
                        n727 = Write to Text File "写入文本文件"(file (use dialog)=path "d:/data/协众产品号B.txt" ("文件（使用对话框）"), text=w1048) -> ()  [unwired: 2 in, 3 out]
                      }
                      frame #1 {
                        n728 = call <vilib>:"System Exec.vi"("run minimized? (F)"=TRUE, "wait until completion? (T)"=TRUE, "command line"="d:\\miniconda3\\python.exe D:\\Data\\Barcode.py ") -> ("error out"=→"error out 4":errorcluster)  [unwired: 5 in, 3 out]
                      }
                      frame #2 {
                        n729 = case shown="真" w1083 {
                          tunnel: [w1105 w1111] -> w1084
                          tunnel: w1082 -> [w1104 w1110]
                          frame False {
                            n730 = case shown="真" w1104 {
                              tunnel: ["NG" ("结果") "NG" ("结果")] -> w1105
                              frame False {
                                w1106 = u16 0 ("合格次数")
                                n731 = local write "检测次数B"(w1106) -> ()
                                n732 = local write "合格次数B"(w1106) -> ()
                              }
                              frame True {
                                w1108 = u16 0 ("合格次数")
                                n733 = local write "检测次数B"(w1108) -> ()
                                n734 = local write "合格次数B"(w1108) -> ()
                              }
                            }
                          }
                          frame True {
                            n735 = case shown="假" w1110 {
                              tunnel: ["OK" ("结果") _] -> w1111
                              frame False {
                                n736 = local write "scan B"(TRUE ("Scan B")) -> ()
                                n737 = local write "2D Code_B"("") -> ()
                                n738 = Read from Text File(file (use dialog)=path "d:/data/打印路径B.txt" ("文件（使用对话框）")) -> (text=w1113:string)  [unwired: 3 in, 3 out]
                                n739 = Concatenate Strings("\"C:\\Program Files\\Seagull\\BarTender Suite\\bartend.exe\" " ("command line"), w1113, " /P/min=SystemTray" ("command line")) -> (w1116:string)
                                n740 = call <vilib>:"System Exec.vi"("run minimized? (F)"=TRUE, "wait until completion? (T)"=FALSE, "command line"=w1116) -> ()  [unwired: 5 in, 4 out]
                              }
                              frame True {
                              }
                            }
                          }
                        }
                        n741 = Read from Text File(file (use dialog)=path "d:/data/序列号B.txt" ("文件（使用对话框）")) -> (text=w1074:string)  [unwired: 3 in, 3 out]
                        n742 = case shown="假" w1083 {
                          tunnel: [w1097 w1102] -> w1069
                          tunnel: [w1094 w1103] -> w1068
                          frame False {
                            n743 = local read "实时漏率B"() -> (w1096:dbl)
                            n744 = Equal To 0?(x=w1096) -> (x = 0?=w1095:bool)
                            n745 = case shown="真" w1095 {
                              tunnel: [w1099 99999.0] -> w1097
                              tunnel: [w1098 w1100] -> w1094
                              frame False {
                                n746 = local read "结果压力 B"() -> (w1098:dbl)
                                n747 = local read "实时漏率B"() -> (w1099:dbl)
                              }
                              frame True {
                                n748 = local read "实时压力B"() -> (w1100:dbl)
                              }
                            }
                          }
                          frame True {
                            n749 = local read "结果压力 B"() -> (w1103:dbl)
                            n750 = local read "实时漏率B"() -> (w1102:dbl)
                          }
                        }
                        n751 = Read from Text File(file (use dialog)=path "d:/data/二维码B.txt" ("文件（使用对话框）")) -> (text=w1071:string)  [unwired: 3 in, 3 out]
                        n752 = Format Date/Time String "格式化日期/时间字符串"(time format string (%c)="%Y/%m/%d %H:%M:%S" ("时间格式字符串(%c)")) -> (date/time string=w1072:string)  [unwired: 2 in]
                        n753 = local read "泄漏单位 2"() -> (w1093:string)
                        n754 = local read "压力单位 2"() -> (w1092:string)
                        n755 = property on="Staff B" class="Ring (严格)"() -> ("Strings []"=w1080:string[], "Value"=w1079:u16)  [unwired: 2 in, 2 out]
                        n756 = Number To Fractional String(number=w1069, width (-)=i16 6 ("宽度(-)"), precision (6)=i16 3 ("精度(6)")) -> (F-format string=w1091:string)  [unwired: 1 in]
                        n757 = Number To Fractional String(number=w1068, width (-)=i16 7 ("宽度(-)"), precision (6)=i16 3 ("精度(6)")) -> (F-format string=w1090:string)  [unwired: 1 in]
                        n758 = Concatenate Strings(w1091, w1093) -> (w1077:string)
                        n759 = Index Array(array=w1080, index=w1079) -> (element=w1078:string)
                        n760 = Concatenate Strings(w1090, w1092) -> (w1085:string)
                        n761 = call "数据库保存子viB1.vi"("#1 Pressure"=w1085, "Part No."=w1070, "Result"=w1084, "2D Code"=w1071, "Person"=w1078, "#1 Leakage"=w1077, "Serial No."=w1074, "Time"=w1072) -> ()  [unwired: 4 in]
                      }
                      frame #3 {
                        n762 = case shown="假" w1122 {
                          frame False {
                            w1123 = u16 0 ("合格次数")
                            n763 = local write "检测次数B"(w1123) -> ()
                            n764 = local write "合格次数B"(w1123) -> ()
                          }
                          frame True {
                          }
                        }
                      }
                    }
                  }
                  frame 2 {
                    n765 = flat-sequence {
                      tunnel: w1124 -> [w1139]
                      frame #0 {
                        n766 = local read "合格次数B"() -> (w1132:u16)
                        n767 = Equal?(x=w1132, y=u16 2) -> (x = y?=w1130:bool)
                        n768 = case shown="真" w1130 {
                          tunnel: ["NG" "OK"] -> w1129
                          frame False {
                            n769 = local write "scan B"(TRUE ("Scan B")) -> ()
                            n770 = local write "2D Code_B"("") -> ()
                          }
                          frame True {
                            n771 = local write "scan B"(TRUE ("Scan B")) -> ()
                            n772 = local write "2D Code_B"("") -> ()
                            n773 = Read from Text File(file (use dialog)=path "d:/data/打印路径B.txt" ("文件（使用对话框）")) -> (text=w1158:string)  [unwired: 3 in, 3 out]
                            n774 = Concatenate Strings("\"C:\\Program Files\\Seagull\\BarTender Suite\\bartend.exe\" " ("command line"), w1158, " /P/min=SystemTray" ("command line")) -> (w1161:string)
                            n775 = call <vilib>:"System Exec.vi"("run minimized? (F)"=TRUE, "wait until completion? (T)"=FALSE, "command line"=w1161) -> ()  [unwired: 5 in, 4 out]
                          }
                        }
                        n776 = case shown="假" w1139 {
                          tunnel: [w1147 w1152] -> w1125
                          tunnel: [w1144 w1153] -> w1126
                          frame False {
                            n777 = local read "实时漏率B"() -> (w1146:dbl)
                            n778 = Equal To 0?(x=w1146) -> (x = 0?=w1145:bool)
                            n779 = case shown="假" w1145 {
                              tunnel: [w1149 99999.0] -> w1147
                              tunnel: [w1148 w1150] -> w1144
                              frame False {
                                n780 = local read "结果压力 B"() -> (w1148:dbl)
                                n781 = local read "实时漏率B"() -> (w1149:dbl)
                              }
                              frame True {
                                n782 = local read "实时压力B"() -> (w1150:dbl)
                              }
                            }
                          }
                          frame True {
                            n783 = local read "结果压力 B"() -> (w1153:dbl)
                            n784 = local read "实时漏率B"() -> (w1152:dbl)
                          }
                        }
                        n785 = local read "压力单位 2"() -> (w1142:string)
                        n786 = local read "泄漏单位 2"() -> (w1143:string)
                        n787 = Number To Fractional String(number=w1126, width (-)=i16 7 ("宽度(-)"), precision (6)=i16 3 ("精度(6)")) -> (F-format string=w1140:string)  [unwired: 1 in]
                        n788 = Number To Fractional String(number=w1125, width (-)=i16 6 ("宽度(-)"), precision (6)=i16 3 ("精度(6)")) -> (F-format string=w1141:string)  [unwired: 1 in]
                        n789 = Concatenate Strings(w1140, w1142) -> (w1134:string)
                        n790 = Concatenate Strings(w1141, w1143) -> (w1133:string)
                        n791 = Read from Text File(file (use dialog)=path "d:/data/序列号B.txt" ("文件（使用对话框）")) -> (text=w1127:string)  [unwired: 3 in, 3 out]
                        n792 = call "数据库插入子viB.vi"("result"=w1129, "2_Leakage"=w1133, "2_Pressure"=w1134, "Serial_No"=w1127) -> ()  [unwired: 8 in]
                      }
                      frame #1 {
                      }
                      frame #2 {
                        w1167 = u16 0 ("合格次数")
                        n793 = local write "检测次数B"(w1167) -> ()
                        n794 = local write "合格次数B"(w1167) -> ()
                      }
                    }
                  }
                }
              }
              frame #3 {
                n795 = call "数据库读取B.vi"() -> ("当日合格数"=w1168:i32, "当天总数"=w1169:i32, "Data"=w1170:string[][])  [unwired: 9 in]
                n796 = property on="B List" class="Tbl (严格)"("Value"=w1170) -> ()  [unwired: 2 in, 2 out]
                n797 = local write "Total Today B"(w1169) -> ()
                n798 = local write "OK Today B"(w1168) -> ()
              }
              frame #4 {
                n799 = local write "合格状态右"(2.0) -> ()
              }
            }
          }
          frame True {
            n800 = flat-sequence {
              tunnel: [w1180] -> w1178
              tunnel: [w1181] -> w1177
              tunnel: w1173 -> [w1181]
              tunnel: w1172 -> [w1180]
              tunnel: [w1183] -> w1176
              tunnel: [w1189] -> w1175
              tunnel: w1178 -> [w1189]
              tunnel: [w1188] -> w1174
              tunnel: w1177 -> [w1188]
              tunnel: w1176 -> [w1212]
              tunnel: w1175 -> [w1210]
              tunnel: w1174 -> [w1209]
              frame #0 {
                n801 = local read "检测次数B"() -> (w1179:u16)
                n802 = Increment(x=w1179) -> (x+1=w1182:u16)
                n803 = local write "检测次数B"(w1182) -> ()
              }
              frame #1 {
                n804 = local read "合格 2"() -> (w1184:bool)
                n805 = property on="PressureUnit 2" class="Ring (严格)"() -> ("Value"=w1191:u16)  [unwired: 2 in, 2 out]
                n806 = property on="LeakUnit 2" class="Ring (严格)"() -> ("Value"=w1190:u16)  [unwired: 2 in, 2 out]
                n807 = Wait (ms)(milliseconds to wait=u32 2000 ("等待时间（毫秒）")) -> ()  [unwired: 1 out]
                n808 = local read "结果压力 B"() -> (w1186:dbl)
                n809 = case shown="0, 默认" w1190 {
                  tunnel: [_ "cm3/min" ("压力单位") "ml/h" ("压力单位") "pa" "pa" "pa/s" ("泄漏单位") "pa/s" ("泄漏单位") "ml/min" ("压力单位")] -> w1187
                  frame 0, Default {
                  }
                  frame 1000 {
                  }
                  frame 2000 {
                  }
                  frame 6000 {
                  }
                  frame 7000 {
                  }
                  frame 8000 {
                  }
                  frame 9000 {
                  }
                  frame 51000 {
                  }
                }
                n810 = case shown="15000" w1191 {
                  frame 0, Default {
                  }
                  frame 11000 {
                    n811 = local write "压力单位 2"("Bar" ("压力单位")) -> ()
                  }
                  frame 12000 {
                    n812 = local write "压力单位 2"("Kpa" ("压力单位")) -> ()
                  }
                  frame 13000 {
                    n813 = local write "压力单位 2"("Psi" ("压力单位")) -> ()
                  }
                  frame 14000 {
                    n814 = local write "压力单位 2"("mbar" ("压力单位")) -> ()
                  }
                  frame 15000 {
                    n815 = local write "压力单位 2"("Mpa") -> ()
                  }
                }
                n816 = Not Equal To 0?(x=w1186) -> (x != 0?=w1185:bool)
                n817 = local write "泄漏单位 2"(w1187) -> ()
                n818 = And(x=w1185, y=w1184) -> (x .and. y?=w1183:bool)
                n819 = case shown="假" w1183 {
                  frame False {
                    n820 = local write "结果 2"("NG" ("结果")) -> ()
                  }
                  frame True {
                    n821 = local read "合格次数B"() -> (w1207:u16)
                    n822 = local write "结果 2"("OK" ("结果")) -> ()
                    n823 = Increment(x=w1207) -> (x+1=w1208:u16)
                    n824 = local write "合格次数B"(w1208) -> ()
                  }
                }
              }
              frame #2 {
                n825 = local read "检测次数B"() -> (w1211:u16)
                n826 = case shown="2" w1211 {
                  tunnel: w1212 -> [_ w1222 w1319]
                  tunnel: w1210 -> [_ w1220 _]
                  tunnel: w1209 -> [_ w1219 _]
                  frame 0, Default {
                  }
                  frame 1 {
                    n827 = flat-sequence {
                      tunnel: [w1238] -> w1218
                      tunnel: w1222 -> [w1238]
                      tunnel: [w1226] -> w1216
                      tunnel: [w1225] -> w1213
                      tunnel: w1218 -> [w1244]
                      tunnel: [w1244] -> w1217
                      tunnel: w1216 -> [w1243]
                      tunnel: [w1243] -> w1215
                      tunnel: [w1242] -> w1214
                      tunnel: w1213 -> [w1242]
                      tunnel: w1217 -> [w1258]
                      tunnel: [w1263] -> w1221
                      tunnel: w1220 -> [w1257]
                      tunnel: w1219 -> [w1263]
                      tunnel: w1215 -> [w1250]
                      tunnel: w1214 -> [w1247]
                      tunnel: w1221 -> [w1317]
                      frame #0 {
                        w1233 = TRUE  # 忽略大小写？(F)
                        w1232 = TRUE  # 替换全部？(F)
                        w1231 = "0"  # 替换字符串("")
                        w1228 = i16 4  # 宽度(-)
                        n828 = call "数据库读取B.vi"() -> ("当天总数"=w1224:i32)  [unwired: 9 in, 2 out]
                        n829 = Increment(x=w1224) -> (x+1=w1223:i32)
                        n830 = Number To Decimal String "数值至十进制数字符串转换"(number=w1223, width (-)=w1228) -> (decimal integer string=w1229:string)
                        n831 = call <vilib>:"Space Constant.vi"() -> ("String"=w1230:string)
                        n832 = property on="参数设置/Setup/Coup monté" class="Tbl (严格)"() -> ("Value"=w1236:string[][])  [unwired: 2 in, 2 out]
                        n833 = Search and Replace String "搜索替换字符串"(replace all?=w1232, case sensitive?=w1233, input string=w1229, search string=w1230, replace string=w1231) -> (result string=w1225:string)  [unwired: 3 in, 3 out]
                        n834 = property on="Part No. B" class="Ring (严格)" props=["Strings []", "Value"]() -> ("Value"=w1235:u16)  [unwired: 2 in, 3 out]
                        n835 = Index Array "索引数组"(array=w1236, index (row)=w1235, index (col)=0 ("禁用的索引 (列)")) -> (element=w1226:string)
                        n836 = Write to Text File "写入文本文件"(file (use dialog)=path "d:/data/序列号B.txt" ("文件（使用对话框）"), text=w1225) -> ()  [unwired: 2 in, 3 out]
                        n837 = Write to Text File "写入文本文件"(file (use dialog)=path "d:/data/协众产品号B.txt" ("文件（使用对话框）"), text=w1226) -> ()  [unwired: 2 in, 3 out]
                      }
                      frame #1 {
                        n838 = call <vilib>:"System Exec.vi"("run minimized? (F)"=TRUE, "wait until completion? (T)"=TRUE, "command line"="\"d:\\miniconda3\\python.exe\" D:\\Data\\Barcode_Cal.py ") -> ()  [unwired: 5 in, 4 out]
                      }
                      frame #2 {
                        n839 = case shown="真" w1258 {
                          tunnel: [w1274 w1294] -> w1259
                          tunnel: w1257 -> [w1273 w1293]
                          frame False {
                            n840 = case shown="假" w1273 {
                              tunnel: ["NG" ("结果") "NG" ("结果")] -> w1274
                              frame False {
                                w1281 = u16 0 ("合格次数")
                                n841 = local write "scan B"(TRUE ("Scan A")) -> ()
                                n842 = local write "2D Code_B"("") -> ()
                                n843 = local write "检测次数B"(w1281) -> ()
                                n844 = local write "合格次数B"(w1281) -> ()
                                n845 = local write "B NG Sample Req.（1st)"(FALSE ("A NG Sample")) -> ()
                                n846 = Read from Text File(file (use dialog)=path "D:/data/Print_Cal_NG_B.txt" ("文件（使用对话框）")) -> (text=w1277:string)  [unwired: 3 in, 3 out]
                                n847 = call <vilib>:"System Exec.vi"("run minimized? (F)"=TRUE, "wait until completion? (T)"=FALSE, "command line"=w1277) -> ()  [unwired: 5 in, 4 out]
                              }
                              frame True {
                                w1291 = u16 0 ("合格次数")
                                n848 = local write "scan B"(TRUE ("Scan A")) -> ()
                                n849 = local write "2D Code_B"("") -> ()
                                n850 = local write "检测次数B"(w1291) -> ()
                                n851 = local write "合格次数B"(w1291) -> ()
                                n852 = local write "B NG Sample Req.（1st)"(FALSE ("A NG Sample")) -> ()
                                n853 = Read from Text File(file (use dialog)=path "D:/data/Print_Cal_OK_B.txt" ("文件（使用对话框）")) -> (text=w1284:string)  [unwired: 3 in, 3 out]
                                n854 = call <vilib>:"System Exec.vi"("run minimized? (F)"=TRUE, "wait until completion? (T)"=FALSE, "command line"=w1284) -> ()  [unwired: 5 in, 4 out]
                              }
                            }
                          }
                          frame True {
                            n855 = case shown="假" w1293 {
                              tunnel: ["OK" ("结果") _] -> w1294
                              frame False {
                                w1300 = u16 0 ("合格次数")
                                n856 = flat-sequence {
                                frame #0 {
                                n857 = local write "B OK Sample Req. (2nd)"(FALSE ("A NG Sample")) -> ()
                                }
                                frame #1 {
                                n858 = local read "B NG Sample Req.（1st)"() -> (w1306:bool)
                                n859 = local read "B OK Sample Req. (2nd)"() -> (w1305:bool)
                                n860 = Or(x=w1306, y=w1305) -> (x .or. y?=w1304:bool)
                                n861 = local write "B Cal. Time"(w1304) -> ()
                                }
                                }
                                n862 = local write "scan B"(TRUE ("Scan A")) -> ()
                                n863 = local write "2D Code_B"("") -> ()
                                n864 = local write "检测次数B"(w1300) -> ()
                                n865 = local write "合格次数B"(w1300) -> ()
                                n866 = Read from Text File(file (use dialog)=path "D:/data/Print_Cal_OK_B.txt" ("文件（使用对话框）")) -> (text=w1296:string)  [unwired: 3 in, 3 out]
                                n867 = call <vilib>:"System Exec.vi"("run minimized? (F)"=TRUE, "wait until completion? (T)"=FALSE, "command line"=w1296) -> ()  [unwired: 5 in, 4 out]
                              }
                              frame True {
                              }
                            }
                          }
                        }
                        n868 = case shown="真" w1258 {
                          tunnel: [w1310 w1315] -> w1245
                          tunnel: [w1307 w1316] -> w1246
                          frame False {
                            n869 = local read "实时漏率B"() -> (w1309:dbl)
                            n870 = Equal To 0?(x=w1309) -> (x = 0?=w1308:bool)
                            n871 = case shown="假" w1308 {
                              tunnel: [w1312 99999.0] -> w1310
                              tunnel: [w1311 w1313] -> w1307
                              frame False {
                                n872 = local read "结果压力 B"() -> (w1311:dbl)
                                n873 = local read "实时漏率B"() -> (w1312:dbl)
                              }
                              frame True {
                                n874 = local read "实时压力B"() -> (w1313:dbl)
                              }
                            }
                          }
                          frame True {
                            n875 = local read "结果压力 B"() -> (w1316:dbl)
                            n876 = local read "实时漏率B"() -> (w1315:dbl)
                          }
                        }
                        n877 = Read from Text File(file (use dialog)=path "d:/data/二维码B.txt" ("文件（使用对话框）")) -> (text=w1248:string)  [unwired: 3 in, 3 out]
                        n878 = local read "压力单位 2"() -> (w1271:string)
                        n879 = local read "泄漏单位 2"() -> (w1272:string)
                        n880 = property on="Staff B" class="Ring (严格)"() -> ("Strings []"=w1262:string[], "Value"=w1261:u16)  [unwired: 2 in, 2 out]
                        n881 = Number To Fractional String(number=w1246, width (-)=i16 6 ("宽度(-)"), precision (6)=i16 3 ("精度(6)")) -> (F-format string=w1269:string)  [unwired: 1 in]
                        n882 = Number To Fractional String(number=w1245, width (-)=i16 7 ("宽度(-)"), precision (6)=i16 3 ("精度(6)")) -> (F-format string=w1270:string)  [unwired: 1 in]
                        n883 = Index Array(array=w1262, index=w1261) -> (element=w1260:string)
                        n884 = Concatenate Strings(w1269, w1271) -> (w1253:string)
                        n885 = Concatenate Strings(w1270, w1272) -> (w1252:string)
                        n886 = Format Date/Time String(time format string (%c)="%Y/%m/%d %H:%M:%S" ("时间格式字符串(%c)")) -> (date/time string=w1254:string)  [unwired: 2 in]
                        n887 = call "数据库保存子viB1.vi"("#1 Pressure"=w1253, "Part No."=w1250, "Result"=w1259, "2D Code"=w1248, "Person"=w1260, "#1 Leakage"=w1252, "Serial No."=w1247, "Time"=w1254) -> ()  [unwired: 4 in]
                        n888 = call <vilib>:"Space Constant.vi"() -> ("String"=w1251:string)
                        n889 = Concatenate Strings(w1254, w1251, w1253, w1251, w1252) -> (w1255:string)
                        n890 = Write to Text File(file (use dialog)=path "d:/data/负压值B.txt" ("文件（使用对话框）"), text=w1255) -> ()  [unwired: 2 in, 3 out]
                      }
                      frame #3 {
                        n891 = case shown="假" w1317 {
                          frame False {
                            w1318 = u16 0 ("合格次数")
                            n892 = local write "检测次数B"(w1318) -> ()
                            n893 = local write "合格次数B"(w1318) -> ()
                          }
                          frame True {
                          }
                        }
                      }
                    }
                  }
                  frame 2 {
                    n894 = flat-sequence {
                      tunnel: w1319 -> [w1329]
                      frame #0 {
                        n895 = case shown="假" w1329 {
                          tunnel: [w1345 w1357] -> w1320
                          tunnel: [w1342 w1358] -> w1321
                          frame False {
                            n896 = local read "实时漏率B"() -> (w1344:dbl)
                            n897 = Equal To 0?(x=w1344) -> (x = 0?=w1343:bool)
                            n898 = case shown="假" w1343 {
                              tunnel: [w1347 99999.0] -> w1345
                              tunnel: [w1346 w1348] -> w1342
                              frame False {
                                n899 = local read "结果漏率 B"() -> (w1346:dbl)
                                n900 = local read "实时漏率B"() -> (w1347:dbl)
                              }
                              frame True {
                                n901 = local read "实时压力B"() -> (w1348:dbl)
                              }
                            }
                          }
                          frame True {
                            w1354 = FALSE ("校准时间到")
                            n902 = local write "scan B"(TRUE ("Scan A")) -> ()
                            n903 = local write "2D Code_B"("") -> ()
                            n904 = local write "B OK Sample Req. (2nd)"(w1354) -> ()
                            n905 = local write "B Cal. Time"(w1354) -> ()
                            n906 = Read from Text File(file (use dialog)=path "D:/data/Print_Cal_OK_B.txt" ("文件（使用对话框）")) -> (text=w1350:string)  [unwired: 3 in, 3 out]
                            n907 = call <vilib>:"System Exec.vi"("run minimized? (F)"=TRUE, "wait until completion? (T)"=FALSE, "command line"=w1350) -> ()  [unwired: 5 in, 4 out]
                            n908 = local read "结果压力 B"() -> (w1358:dbl)
                            n909 = local read "实时漏率B"() -> (w1357:dbl)
                          }
                        }
                        n910 = local read "合格次数B"() -> (w1335:u16)
                        n911 = Equal?(x=w1335, y=u16 2) -> (x = y?=w1333:bool)
                        n912 = case shown="假" w1333 {
                          tunnel: ["NG" "OK"] -> w1332
                          frame False {
                          }
                          frame True {
                          }
                        }
                        n913 = local read "压力单位 2"() -> (w1325:string)
                        n914 = local read "泄漏单位 2"() -> (w1324:string)
                        n915 = Number To Fractional String(number=w1321, width (-)=i16 6 ("宽度(-)"), precision (6)=i16 3 ("精度(6)")) -> (F-format string=w1341:string)  [unwired: 1 in]
                        n916 = Number To Fractional String(number=w1320, width (-)=i16 7 ("宽度(-)"), precision (6)=i16 3 ("精度(6)")) -> (F-format string=w1340:string)  [unwired: 1 in]
                        n917 = Concatenate Strings(w1341, w1325) -> (w1323:string)
                        n918 = Concatenate Strings(w1340, w1324) -> (w1322:string)
                        n919 = Read from Text File(file (use dialog)=path "d:/data/序列号B.txt" ("文件（使用对话框）")) -> (text=w1330:string)  [unwired: 3 in, 3 out]
                        n920 = call "数据库插入子viB.vi"("result"=w1332, "2_Leakage"=w1322, "2_Pressure"=w1323, "Serial_No"=w1330) -> ()  [unwired: 8 in]
                        n921 = call <vilib>:"Space Constant.vi"() -> ("String"=w1327:string)
                        n922 = Concatenate Strings(w1323, w1327, w1322) -> (w1328:string)
                        n923 = Write to Text File "写入文本文件"(file (use dialog)=path "d:/data/正压值B.txt" ("文件（使用对话框）"), text=w1328) -> ()  [unwired: 2 in, 3 out]
                      }
                      frame #1 {
                        n924 = Wait (ms)(milliseconds to wait=u32 2000 ("等待时间（毫秒）")) -> ()  [unwired: 1 out]
                      }
                      frame #2 {
                        w1364 = u16 0 ("合格次数")
                        n925 = local write "合格次数B"(w1364) -> ()
                        n926 = local write "检测次数B"(w1364) -> ()
                        n927 = Write to Text File "写入文本文件"(file (use dialog)=path "d:/data/正压值B.txt" ("文件（使用对话框）"), text="") -> ()  [unwired: 2 in, 3 out]
                      }
                    }
                  }
                }
              }
              frame #3 {
                n928 = call "数据库读取B.vi"() -> ("当日合格数"=w1365:i32, "当天总数"=w1366:i32, "Data"=w1367:string[][])  [unwired: 9 in]
                n929 = property on="B List" class="Tbl (严格)"("Value"=w1367) -> ()  [unwired: 2 in, 2 out]
                n930 = local write "Total Today B"(w1366) -> ()
                n931 = local write "OK Today B"(w1365) -> ()
              }
              frame #4 {
                n932 = local write "合格状态右"(2.0) -> ()
              }
            }
          }
        }
      }
      frame 2, Default {
        n933 = flat-sequence {
          tunnel: w1370 -> [w1372]
          tunnel: [w1372] -> w1369
          tunnel: w1369 -> [w1373]
          frame #0 {
            n934 = Wait (ms)(milliseconds to wait=u32 3000 ("等待时间（毫秒）")) -> ()  [unwired: 1 out]
          }
          frame #1 {
            n935 = case shown="假" w1373 {
              frame False {
                n936 = local write "合格状态右"(0.0 ("合格状态")) -> ()
              }
              frame True {
              }
            }
          }
        }
      }
    }
    "数字不跳动，表示软件死机B" <- w982
  }
  n937 = while {
    i -> [w1376]
    stop <- FALSE stop-if-true
    n938 = local read "Single/Dual A"() -> (w1379:bool)
    n939 = Wait (ms)(milliseconds to wait=u32 250 ("等待时间（毫秒）")) -> ()  [unwired: 1 out]
    n940 = case shown="真" "A启动信号" {
      frame False {
      }
      frame True {
        n941 = local write "2D Code_A"("") -> ()
      }
    }
    n942 = local read "A结果信号"() -> (w1377:bool)
    n943 = case shown="1" "合格状态左" {
      tunnel: w1377 -> [w1383 _ w1781]
      tunnel: w1379 -> [_ w1391 _]
      tunnel: w1379 -> [_ w1390 _]
      frame 0 {
        n944 = case shown="真" w1383 {
          frame False {
          }
          frame True {
            n945 = local write "合格状态左"(1.0 ("合格状态")) -> ()
          }
        }
      }
      frame 1 {
        n946 = local read "A NG Sample Req.（1st)"() -> (w1389:bool)
        n947 = local read "A OK Sample Req. (2nd)"() -> (w1388:bool)
        n948 = local read "A Cal. Time"() -> (w1386:bool)
        n949 = Or(x=w1389, y=w1388) -> (x .or. y?=w1387:bool)
        n950 = And(x=w1386, y=w1387) -> (x .and. y?=w1385:bool)
        n951 = case shown="假" w1385 {
          tunnel: w1391 -> [w1393 w1580]
          tunnel: w1390 -> [w1392 w1579]
          frame False {
            n952 = flat-sequence {
              tunnel: [w1400] -> w1398
              tunnel: [w1401] -> w1397
              tunnel: w1393 -> [w1401]
              tunnel: w1392 -> [w1400]
              tunnel: [w1403] -> w1396
              tunnel: [w1408] -> w1395
              tunnel: w1398 -> [w1408]
              tunnel: [w1407] -> w1394
              tunnel: w1397 -> [w1407]
              tunnel: w1396 -> [w1431]
              tunnel: w1395 -> [w1429]
              tunnel: w1394 -> [w1428]
              frame #0 {
                n953 = local read "检测次数A"() -> (w1399:u16)
                n954 = Increment(x=w1399) -> (x+1=w1402:u16)
                n955 = local write "检测次数A"(w1402) -> ()
              }
              frame #1 {
                n956 = property on="LeakUnit" class="Ring (严格)"() -> ("Value"=w1409:u16)  [unwired: 2 in, 2 out]
                n957 = property on="PressureUnit" class="Ring (严格)"() -> ("Value"=w1410:u16)  [unwired: 2 in, 2 out]
                n958 = local read "合格"() -> (w1404:bool)
                n959 = case shown="6000" w1409 {
                  frame 0, Default {
                  }
                  frame 1000 {
                    n960 = local write "泄漏单位"("cm3/min" ("压力单位")) -> ()
                  }
                  frame 2000 {
                    n961 = local write "泄漏单位"("ml/h" ("压力单位")) -> ()
                  }
                  frame 6000 {
                    n962 = local write "泄漏单位"("pa") -> ()
                  }
                  frame 7000 {
                    n963 = local write "泄漏单位"("pa") -> ()
                  }
                  frame 8000 {
                    n964 = local write "泄漏单位"("pa/s" ("泄漏单位")) -> ()
                  }
                  frame 9000 {
                    n965 = local write "泄漏单位"("pa/s" ("泄漏单位")) -> ()
                  }
                  frame 51000 {
                    n966 = local write "泄漏单位"("ml/min" ("压力单位")) -> ()
                  }
                }
                n967 = Wait (ms)(milliseconds to wait=u32 2000 ("等待时间（毫秒）")) -> ()  [unwired: 1 out]
                n968 = case shown="15000" w1410 {
                  frame 0, Default {
                  }
                  frame 11000 {
                    n969 = local write "压力单位"("Bar" ("压力单位")) -> ()
                  }
                  frame 12000 {
                    n970 = local write "压力单位"("Kpa" ("压力单位")) -> ()
                  }
                  frame 13000 {
                    n971 = local write "压力单位"("Psi" ("压力单位")) -> ()
                  }
                  frame 14000 {
                    n972 = local write "压力单位"("mbar" ("压力单位")) -> ()
                  }
                  frame 15000 {
                    n973 = local write "压力单位"("Mpa") -> ()
                  }
                }
                n974 = local read "结果压力"() -> (w1406:dbl)
                n975 = Not Equal To 0?(x=w1406) -> (x != 0?=w1405:bool)
                n976 = And(x=w1404, y=w1405) -> (x .and. y?=w1403:bool)
                n977 = case shown="真" w1403 {
                  frame False {
                    n978 = local write "结果"("NG" ("结果")) -> ()
                  }
                  frame True {
                    n979 = local read "合格次数A"() -> (w1426:u16)
                    n980 = local write "结果"("OK" ("结果")) -> ()
                    n981 = Increment(x=w1426) -> (x+1=w1427:u16)
                    n982 = local write "合格次数A"(w1427) -> ()
                  }
                }
              }
              frame #2 {
                n983 = local read "检测次数A"() -> (w1430:u16)
                n984 = case shown="2" w1430 {
                  tunnel: w1431 -> [_ w1444 w1531]
                  tunnel: w1429 -> [_ w1443 _]
                  tunnel: w1428 -> [_ w1442 _]
                  frame 0, Default {
                  }
                  frame 1 {
                    n985 = flat-sequence {
                      tunnel: [w1460] -> w1435
                      tunnel: w1444 -> [w1460]
                      tunnel: [w1447] -> w1433
                      tunnel: w1435 -> [w1463]
                      tunnel: [w1463] -> w1434
                      tunnel: w1433 -> [w1462]
                      tunnel: [w1462] -> w1432
                      tunnel: w1434 -> [w1470]
                      tunnel: [w1470] -> w1439
                      tunnel: [w1466] -> w1437
                      tunnel: w1432 -> [w1466]
                      tunnel: w1439 -> [w1473]
                      tunnel: [w1473] -> w1438
                      tunnel: w1437 -> [w1472]
                      tunnel: [w1472] -> w1436
                      tunnel: w1438 -> [w1486]
                      tunnel: [w1484] -> w1441
                      tunnel: w1443 -> [w1485]
                      tunnel: w1442 -> [w1484]
                      tunnel: w1436 -> [w1476]
                      tunnel: w1441 -> [w1528]
                      tunnel: [w1528] -> w1440
                      tunnel: w1440 -> [w1529]
                      frame #0 {
                        w1455 = TRUE  # 忽略大小写？(F)
                        w1454 = TRUE  # 替换全部？(F)
                        w1453 = "0"  # 替换字符串("")
                        w1450 = i16 4  # 宽度(-)
                        n986 = call "数据库读取.vi"() -> ("当天总数"=w1446:i32)  [unwired: 9 in, 2 out]
                        n987 = Increment(x=w1446) -> (x+1=w1445:i32)
                        n988 = Number To Decimal String "数值至十进制数字符串转换"(number=w1445, width (-)=w1450) -> (decimal integer string=w1451:string)
                        n989 = property on="参数设置/Setup/Coup monté" class="Tbl (严格)"() -> ("Value"=w1458:string[][])  [unwired: 2 in, 2 out]
                        n990 = call <vilib>:"Space Constant.vi"() -> ("String"=w1452:string)
                        n991 = property on="Part No. A" class="Ring (严格)" props=["Strings []", "Value"]() -> ("Value"=w1457:u16)  [unwired: 2 in, 3 out]
                        n992 = Search and Replace String "搜索替换字符串"(replace all?=w1454, case sensitive?=w1455, input string=w1451, search string=w1452, replace string=w1453) -> (result string=w1448:string)  [unwired: 3 in, 3 out]
                        n993 = Index Array "索引数组"(array=w1458, index (row)=w1457, index (col)=0 ("禁用的索引 (列)")) -> (element=w1447:string)
                        n994 = Write to Text File "写入文本文件"(file (use dialog)=path "d:/data/序列号A.txt" ("文件（使用对话框）"), text=w1448) -> ()  [unwired: 2 in, 3 out]
                        n995 = Write to Text File "写入文本文件"(file (use dialog)=path "d:/data/协众产品号A.txt" ("文件（使用对话框）"), text=w1447) -> ()  [unwired: 2 in, 3 out]
                      }
                      frame #1 {
                        n996 = Wait (ms)(milliseconds to wait=u32 200 ("等待时间（毫秒）")) -> ()  [unwired: 1 out]
                      }
                      frame #2 {
                        n997 = Wait (ms)(milliseconds to wait=u32 500 ("等待时间（毫秒）")) -> ()  [unwired: 1 out]
                        n998 = call <vilib>:"System Exec.vi"("run minimized? (F)"=TRUE, "wait until completion? (T)"=FALSE, "command line"="d:\\miniconda3\\python.exe D:\\Data\\Barcode.py ") -> ("error out"=→"error out":errorcluster)  [unwired: 5 in, 3 out]
                      }
                      frame #3 {
                        n999 = Wait (ms)(milliseconds to wait=u32 100 ("等待时间（毫秒）")) -> ()  [unwired: 1 out]
                      }
                      frame #4 {
                        w1491 = i16 3  # 精度(6)
                        w1490 = i16 6  # 宽度(-)
                        w1493 = i16 3  # 精度(6)
                        w1492 = i16 7  # 宽度(-)
                        w1489 = "%Y/%m/%d %H:%M:%S"  # 时间格式字符串(%c)
                        n1000 = case shown="真" w1486 {
                          tunnel: [w1511 w1516] -> w1487
                          tunnel: w1485 -> [w1510 w1515]
                          frame False {
                            n1001 = case shown="真" w1510 {
                              tunnel: ["NG" ("结果") "NG" ("结果")] -> w1511
                              frame False {
                              }
                              frame True {
                                w1513 = u16 0 ("合格次数")
                                n1002 = local write "检测次数A"(w1513) -> ()
                                n1003 = local write "合格次数A"(w1513) -> ()
                              }
                            }
                          }
                          frame True {
                            n1004 = case shown="假" w1515 {
                              tunnel: ["OK" ("结果") _] -> w1516
                              frame False {
                                n1005 = local write "scan A"(TRUE ("Scan A")) -> ()
                                n1006 = local write "2D Code_A"("") -> ()
                                n1007 = Read from Text File(file (use dialog)=path "d:/data/打印路径A.txt" ("文件（使用对话框）")) -> (text=w1518:string)  [unwired: 3 in, 3 out]
                                n1008 = Concatenate Strings("\"C:\\Program Files\\Seagull\\BarTender Suite\\bartend.exe\" " ("command line"), w1518, " /P/min=SystemTray" ("command line")) -> (w1522:string)
                                n1009 = Wait (ms)(milliseconds to wait=u32 1000 ("等待时间（毫秒）")) -> ()  [unwired: 1 out]
                                n1010 = call <vilib>:"System Exec.vi"("run minimized? (F)"=TRUE, "wait until completion? (T)"=FALSE, "command line"=w1522) -> ()  [unwired: 5 in, 4 out]
                              }
                              frame True {
                              }
                            }
                          }
                        }
                        n1011 = case shown="假" w1486 {
                          tunnel: [w1503 w1508] -> w1475
                          tunnel: [w1500 w1509] -> w1474
                          frame False {
                            n1012 = local read "实时漏率A"() -> (w1502:dbl)
                            n1013 = Equal To 0? "等于0？"(x=w1502) -> (x = 0?=w1501:bool)
                            n1014 = case "条件结构" shown="假" w1501 {
                              tunnel: [w1504 99999.0] -> w1503
                              tunnel: [w1505 w1506] -> w1500
                              frame False {
                                n1015 = local read "实时漏率A"() -> (w1504:dbl)
                                n1016 = local read "结果压力"() -> (w1505:dbl)
                              }
                              frame True {
                                n1017 = local read "实时压力A"() -> (w1506:dbl)
                              }
                            }
                          }
                          frame True {
                            n1018 = local read "实时漏率A"() -> (w1508:dbl)
                            n1019 = local read "结果压力"() -> (w1509:dbl)
                          }
                        }
                        n1020 = Number To Fractional String "数值至小数字符串转换"(number=w1475, width (-)=w1490, precision (6)=w1491) -> (F-format string=w1495:string)  [unwired: 1 in]
                        n1021 = Number To Fractional String "数值至小数字符串转换"(number=w1474, width (-)=w1492, precision (6)=w1493) -> (F-format string=w1494:string)  [unwired: 1 in]
                        n1022 = local read "泄漏单位"() -> (w1497:string)
                        n1023 = local read "压力单位"() -> (w1496:string)
                        n1024 = Format Date/Time String "格式化日期/时间字符串"(time format string (%c)=w1489) -> (date/time string=w1498:string)  [unwired: 2 in]
                        n1025 = Concatenate Strings "连接字符串"(w1495, w1497) -> (w1499:string)
                        n1026 = property on="Staff A" class="Ring (严格)"() -> ("Strings []"=w1483:string[], "Value"=w1482:u16)  [unwired: 2 in, 2 out]
                        n1027 = Concatenate Strings "连接字符串"(w1494, w1496) -> (w1488:string)
                        n1028 = Index Array "索引数组"(array=w1483, index=w1482) -> (element=w1481:string)
                        n1029 = Read from Text File(file (use dialog)=path "d:/data/序列号A.txt" ("文件（使用对话框）")) -> (text=w1480:string)  [unwired: 3 in, 3 out]
                        n1030 = Read from Text File(file (use dialog)=path "d:/data/二维码A.txt" ("文件（使用对话框）")) -> (text=w1477:string)  [unwired: 3 in, 3 out]
                        n1031 = call "数据库保存子vi.vi"("#1 Pressure"=w1488, "Part No."=w1476, "Result"=w1487, "2D Code"=w1477, "Person"=w1481, "#1 Leakage"=w1499, "Serial No."=w1480, "Time"=w1498) -> ()  [unwired: 4 in]
                      }
                      frame #5 {
                      }
                      frame #6 {
                        n1032 = case shown="假" w1529 {
                          frame False {
                            w1530 = u16 0 ("合格次数")
                            n1033 = local write "检测次数A"(w1530) -> ()
                            n1034 = local write "合格次数A"(w1530) -> ()
                          }
                          frame True {
                          }
                        }
                      }
                    }
                  }
                  frame 2 {
                    n1035 = flat-sequence {
                      tunnel: w1531 -> [w1546]
                      frame #0 {
                        w1535 = path "d:/data/序列号A.txt"  # 文件（使用对话框）
                        w1538 = u16 2  # y
                        w1543 = i16 3  # 精度(6)
                        w1542 = i16 6  # 宽度(-)
                        w1545 = i16 3  # 精度(6)
                        w1544 = i16 7  # 宽度(-)
                        n1036 = case shown="真" w1546 {
                          tunnel: [w1554 w1568] -> w1533
                          tunnel: [w1551 w1569] -> w1532
                          frame False {
                            n1037 = local read "实时漏率A"() -> (w1553:dbl)
                            n1038 = Equal To 0?(x=w1553) -> (x = 0?=w1552:bool)
                            n1039 = case shown="真" w1552 {
                              tunnel: [w1555 99999.0] -> w1554
                              tunnel: [w1556 w1557] -> w1551
                              frame False {
                                n1040 = local read "实时漏率A"() -> (w1555:dbl)
                                n1041 = local read "结果压力"() -> (w1556:dbl)
                              }
                              frame True {
                                n1042 = local read "实时压力A"() -> (w1557:dbl)
                              }
                            }
                          }
                          frame True {
                            n1043 = local write "scan A"(TRUE ("Scan A")) -> ()
                            n1044 = local write "2D Code_A"("") -> ()
                            n1045 = Read from Text File(file (use dialog)=path "d:/data/打印路径A.txt" ("文件（使用对话框）")) -> (text=w1559:string)  [unwired: 3 in, 3 out]
                            n1046 = Concatenate Strings("\"C:\\Program Files\\Seagull\\BarTender Suite\\bartend.exe\" " ("command line"), w1559, " /P/min=SystemTray" ("command line")) -> (w1563:string)
                            n1047 = local read "实时漏率A"() -> (w1568:dbl)
                            n1048 = local read "结果压力"() -> (w1569:dbl)
                            n1049 = call <vilib>:"System Exec.vi"("run minimized? (F)"=TRUE, "wait until completion? (T)"=FALSE, "command line"=w1563) -> ()  [unwired: 5 in, 4 out]
                          }
                        }
                        n1050 = local read "合格次数A"() -> (w1539:u16)
                        n1051 = Number To Fractional String "数值至小数字符串转换"(number=w1532, width (-)=w1544, precision (6)=w1545) -> (F-format string=w1547:string)  [unwired: 1 in]
                        n1052 = Number To Fractional String "数值至小数字符串转换"(number=w1533, width (-)=w1542, precision (6)=w1543) -> (F-format string=w1548:string)  [unwired: 1 in]
                        n1053 = Equal? "等于？"(x=w1539, y=w1538) -> (x = y?=w1537:bool)
                        n1054 = local read "压力单位"() -> (w1549:string)
                        n1055 = local read "泄漏单位"() -> (w1550:string)
                        n1056 = case "条件结构" shown="真" w1537 {
                          tunnel: ["NG" "OK"] -> w1536
                          frame False {
                          }
                          frame True {
                          }
                        }
                        n1057 = Read from Text File "读取文本文件"(file (use dialog)=w1535) -> (text=w1534:string)  [unwired: 3 in, 3 out]
                        n1058 = Concatenate Strings "连接字符串"(w1547, w1549) -> (w1541:string)
                        n1059 = Concatenate Strings "连接字符串"(w1548, w1550) -> (w1540:string)
                        n1060 = call "数据库插入子vi.vi"("result"=w1536, "2_Leakage"=w1540, "2_Pressure"=w1541, "Serial_No"=w1534) -> ()  [unwired: 8 in]
                      }
                      frame #1 {
                        w1574 = u16 0 ("合格次数")
                        n1061 = local write "检测次数A"(w1574) -> ()
                        n1062 = local write "合格次数A"(w1574) -> ()
                        n1063 = Write to Text File "写入文本文件"(file (use dialog)=path "d:/data/正压值A.txt" ("文件（使用对话框）"), text="") -> ()  [unwired: 2 in, 3 out]
                      }
                    }
                  }
                }
              }
              frame #3 {
                n1064 = call "数据库读取.vi"() -> ("当日合格数"=w1575:i32, "当天总数"=w1576:i32, "Data"=w1577:string[][])  [unwired: 9 in]
                n1065 = property on="A List" class="Tbl (严格)"("Value"=w1577) -> ()  [unwired: 2 in, 2 out]
                n1066 = local write "Total Today A"(w1576) -> ()
                n1067 = local write "OK Today A"(w1575) -> ()
              }
              frame #4 {
                n1068 = local write "合格状态左"(2.0) -> ()
              }
            }
          }
          frame True {
            n1069 = flat-sequence {
              tunnel: [w1587] -> w1585
              tunnel: [w1588] -> w1584
              tunnel: w1580 -> [w1588]
              tunnel: w1579 -> [w1587]
              tunnel: [w1590] -> w1583
              tunnel: [w1594] -> w1582
              tunnel: w1585 -> [w1594]
              tunnel: [w1595] -> w1581
              tunnel: w1584 -> [w1595]
              tunnel: w1583 -> [w1618]
              tunnel: w1582 -> [w1616]
              tunnel: w1581 -> [w1615]
              frame #0 {
                n1070 = local read "检测次数A"() -> (w1586:u16)
                n1071 = Increment(x=w1586) -> (x+1=w1589:u16)
                n1072 = local write "检测次数A"(w1589) -> ()
              }
              frame #1 {
                n1073 = local read "结果压力"() -> (w1593:dbl)
                n1074 = property on="LeakUnit" class="Ring (严格)"() -> ("Value"=w1596:u16)  [unwired: 2 in, 2 out]
                n1075 = local read "合格"() -> (w1591:bool)
                n1076 = property on="PressureUnit" class="Ring (严格)"() -> ("Value"=w1597:u16)  [unwired: 2 in, 2 out]
                n1077 = Wait (ms)(milliseconds to wait=u32 2000 ("等待时间（毫秒）")) -> ()  [unwired: 1 out]
                n1078 = case shown="6000" w1596 {
                  frame 0, Default {
                  }
                  frame 1000 {
                    n1079 = local write "泄漏单位"("cm3/min" ("压力单位")) -> ()
                  }
                  frame 2000 {
                    n1080 = local write "泄漏单位"("ml/h" ("压力单位")) -> ()
                  }
                  frame 6000 {
                    n1081 = local write "泄漏单位"("pa") -> ()
                  }
                  frame 7000 {
                    n1082 = local write "泄漏单位"("pa") -> ()
                  }
                  frame 8000 {
                    n1083 = local write "泄漏单位"("pa/s" ("泄漏单位")) -> ()
                  }
                  frame 9000 {
                    n1084 = local write "泄漏单位"("pa/s" ("泄漏单位")) -> ()
                  }
                  frame 51000 {
                    n1085 = local write "泄漏单位"("ml/min" ("压力单位")) -> ()
                  }
                }
                n1086 = case shown="15000" w1597 {
                  frame 0, Default {
                  }
                  frame 11000 {
                    n1087 = local write "压力单位"("Bar" ("压力单位")) -> ()
                  }
                  frame 12000 {
                    n1088 = local write "压力单位"("Kpa" ("压力单位")) -> ()
                  }
                  frame 13000 {
                    n1089 = local write "压力单位"("Psi" ("压力单位")) -> ()
                  }
                  frame 14000 {
                    n1090 = local write "压力单位"("mbar" ("压力单位")) -> ()
                  }
                  frame 15000 {
                    n1091 = local write "压力单位"("Mpa") -> ()
                  }
                }
                n1092 = Not Equal To 0?(x=w1593) -> (x != 0?=w1592:bool)
                n1093 = And(x=w1591, y=w1592) -> (x .and. y?=w1590:bool)
                n1094 = case shown="真" w1590 {
                  frame False {
                    n1095 = local write "结果"("NG" ("结果")) -> ()
                  }
                  frame True {
                    n1096 = local read "合格次数A"() -> (w1613:u16)
                    n1097 = local write "结果"("OK" ("结果")) -> ()
                    n1098 = Increment(x=w1613) -> (x+1=w1614:u16)
                    n1099 = local write "合格次数A"(w1614) -> ()
                  }
                }
              }
              frame #2 {
                n1100 = local read "检测次数A"() -> (w1617:u16)
                n1101 = case shown="2" w1617 {
                  tunnel: w1618 -> [_ w1631 w1730]
                  tunnel: w1616 -> [_ w1629 _]
                  tunnel: w1615 -> [_ w1628 _]
                  frame 0, Default {
                  }
                  frame 1 {
                    n1102 = flat-sequence {
                      tunnel: [w1647] -> w1624
                      tunnel: w1631 -> [w1647]
                      tunnel: [w1636] -> w1622
                      tunnel: [w1632] -> w1620
                      tunnel: w1624 -> [w1650]
                      tunnel: [w1650] -> w1623
                      tunnel: w1622 -> [w1649]
                      tunnel: [w1649] -> w1621
                      tunnel: w1620 -> [w1648]
                      tunnel: [w1648] -> w1619
                      tunnel: w1623 -> [w1656]
                      tunnel: [w1656] -> w1627
                      tunnel: [w1652] -> w1626
                      tunnel: w1621 -> [w1652]
                      tunnel: [w1651] -> w1625
                      tunnel: w1619 -> [w1651]
                      tunnel: w1627 -> [w1674]
                      tunnel: [w1672] -> w1630
                      tunnel: w1629 -> [w1673]
                      tunnel: w1628 -> [w1672]
                      tunnel: w1626 -> [w1661]
                      tunnel: w1625 -> [w1659]
                      tunnel: w1630 -> [w1728]
                      frame #0 {
                        w1641 = TRUE  # 忽略大小写？(F)
                        w1642 = TRUE  # 替换全部？(F)
                        w1643 = "0"  # 替换字符串("")
                        w1646 = i16 4  # 宽度(-)
                        n1103 = call "数据库读取.vi"() -> ("当天总数"=w1634:i32)  [unwired: 9 in, 2 out]
                        n1104 = Increment(x=w1634) -> (x+1=w1633:i32)
                        n1105 = Number To Decimal String "数值至十进制数字符串转换"(number=w1633, width (-)=w1646) -> (decimal integer string=w1645:string)
                        n1106 = call <vilib>:"Space Constant.vi"() -> ("String"=w1644:string)
                        n1107 = property on="参数设置/Setup/Coup monté" class="Tbl (严格)"() -> ("Value"=w1638:string[][])  [unwired: 2 in, 2 out]
                        n1108 = Search and Replace String "搜索替换字符串"(replace all?=w1642, case sensitive?=w1641, input string=w1645, search string=w1644, replace string=w1643) -> (result string=w1632:string)  [unwired: 3 in, 3 out]
                        n1109 = property on="Part No. A" class="Ring (严格)" props=["Strings []", "Value"]() -> ("Value"=w1639:u16)  [unwired: 2 in, 3 out]
                        n1110 = Index Array "索引数组"(array=w1638, index (row)=w1639, index (col)=0 ("禁用的索引 (列)")) -> (element=w1636:string)
                        n1111 = Write to Text File "写入文本文件"(file (use dialog)=path "d:/data/序列号A.txt" ("文件（使用对话框）"), text=w1632) -> ()  [unwired: 2 in, 3 out]
                        n1112 = Write to Text File "写入文本文件"(file (use dialog)=path "d:/data/协众产品号A.txt" ("文件（使用对话框）"), text=w1636) -> ()  [unwired: 2 in, 3 out]
                      }
                      frame #1 {
                      }
                      frame #2 {
                        n1113 = call <vilib>:"System Exec.vi"("run minimized? (F)"=TRUE, "wait until completion? (T)"=TRUE, "command line"="\"d:\\miniconda3\\python.exe\" D:\\Data\\Barcode_Cal.py ") -> ()  [unwired: 5 in, 4 out]
                      }
                      frame #3 {
                        w1678 = i16 3  # 精度(6)
                        w1677 = i16 6  # 宽度(-)
                        w1680 = i16 3  # 精度(6)
                        w1679 = i16 7  # 宽度(-)
                        w1676 = "%Y/%m/%d %H:%M:%S"  # 时间格式字符串(%c)
                        n1114 = case shown="真" w1674 {
                          tunnel: [w1688 w1693] -> w1657
                          tunnel: [w1685 w1694] -> w1658
                          frame False {
                            n1115 = local read "实时漏率A"() -> (w1687:dbl)
                            n1116 = Equal To 0? "等于0？"(x=w1687) -> (x = 0?=w1686:bool)
                            n1117 = case "条件结构" shown="假" w1686 {
                              tunnel: [w1690 99999.0] -> w1688
                              tunnel: [w1689 w1691] -> w1685
                              frame False {
                                n1118 = local read "实时漏率A"() -> (w1690:dbl)
                                n1119 = local read "结果压力"() -> (w1689:dbl)
                              }
                              frame True {
                                n1120 = local read "实时压力A"() -> (w1691:dbl)
                              }
                            }
                          }
                          frame True {
                            n1121 = local read "实时漏率A"() -> (w1693:dbl)
                            n1122 = local read "结果压力"() -> (w1694:dbl)
                          }
                        }
                        n1123 = case shown="真" w1674 {
                          tunnel: [w1696 w1715] -> w1675
                          tunnel: w1673 -> [w1695 w1714]
                          frame False {
                            n1124 = case shown="假" w1695 {
                              tunnel: ["NG" ("结果") "NG" ("结果")] -> w1696
                              frame False {
                                w1702 = u16 0 ("合格次数")
                                n1125 = local write "scan A"(TRUE ("Scan A")) -> ()
                                n1126 = local write "2D Code_A"("") -> ()
                                n1127 = local write "检测次数A"(w1702) -> ()
                                n1128 = local write "合格次数A"(w1702) -> ()
                                n1129 = local write "A NG Sample Req.（1st)"(FALSE ("A NG Sample")) -> ()
                                n1130 = Read from Text File(file (use dialog)=path "D:/data/Print_Cal_NG_A.txt" ("文件（使用对话框）")) -> (text=w1698:string)  [unwired: 3 in, 3 out]
                                n1131 = call <vilib>:"System Exec.vi"("run minimized? (F)"=TRUE, "wait until completion? (T)"=FALSE, "command line"=w1698) -> ()  [unwired: 5 in, 4 out]
                              }
                              frame True {
                                w1712 = u16 0 ("合格次数")
                                n1132 = local write "scan A"(TRUE ("Scan A")) -> ()
                                n1133 = local write "检测次数A"(w1712) -> ()
                                n1134 = local write "合格次数A"(w1712) -> ()
                                n1135 = local write "A NG Sample Req.（1st)"(FALSE ("A NG Sample")) -> ()
                                n1136 = Read from Text File(file (use dialog)=path "D:/data/Print_Cal_NG_A.txt" ("文件（使用对话框）")) -> (text=w1706:string)  [unwired: 3 in, 3 out]
                                n1137 = call <vilib>:"System Exec.vi"("run minimized? (F)"=TRUE, "wait until completion? (T)"=FALSE, "command line"=w1706) -> ()  [unwired: 5 in, 4 out]
                              }
                            }
                          }
                          frame True {
                            n1138 = case shown="假" w1714 {
                              tunnel: ["OK" ("结果") _] -> w1715
                              frame False {
                                w1720 = u16 0 ("合格次数")
                                n1139 = flat-sequence {
                                frame #0 {
                                n1140 = local write "A OK Sample Req. (2nd)"(FALSE ("A NG Sample")) -> ()
                                }
                                frame #1 {
                                n1141 = local read "A NG Sample Req.（1st)"() -> (w1727:bool)
                                n1142 = local read "A OK Sample Req. (2nd)"() -> (w1726:bool)
                                n1143 = Or(x=w1727, y=w1726) -> (x .or. y?=w1725:bool)
                                n1144 = local write "A Cal. Time"(w1725) -> ()
                                }
                                }
                                n1145 = local write "scan A"(TRUE ("Scan A")) -> ()
                                n1146 = local write "2D Code_A"("") -> ()
                                n1147 = local write "检测次数A"(w1720) -> ()
                                n1148 = local write "合格次数A"(w1720) -> ()
                                n1149 = Read from Text File(file (use dialog)=path "D:/data/Print_Cal_OK_A.txt" ("文件（使用对话框）")) -> (text=w1716:string)  [unwired: 3 in, 3 out]
                                n1150 = call <vilib>:"System Exec.vi"("run minimized? (F)"=TRUE, "wait until completion? (T)"=FALSE, "command line"=w1716) -> ()  [unwired: 5 in, 4 out]
                              }
                              frame True {
                              }
                            }
                          }
                        }
                        n1151 = Number To Fractional String "数值至小数字符串转换"(number=w1658, width (-)=w1679, precision (6)=w1680) -> (F-format string=w1681:string)  [unwired: 1 in]
                        n1152 = Number To Fractional String "数值至小数字符串转换"(number=w1657, width (-)=w1677, precision (6)=w1678) -> (F-format string=w1682:string)  [unwired: 1 in]
                        n1153 = local read "压力单位"() -> (w1683:string)
                        n1154 = local read "泄漏单位"() -> (w1684:string)
                        n1155 = Format Date/Time String "格式化日期/时间字符串"(time format string (%c)=w1676) -> (date/time string=w1667:string)  [unwired: 2 in]
                        n1156 = Read from Text File(file (use dialog)=path "d:/data/二维码A.txt" ("文件（使用对话框）")) -> (text=w1660:string)  [unwired: 3 in, 3 out]
                        n1157 = Concatenate Strings "连接字符串"(w1681, w1683) -> (w1665:string)
                        n1158 = Concatenate Strings "连接字符串"(w1682, w1684) -> (w1666:string)
                        n1159 = property on="Staff A" class="Ring (严格)"() -> ("Strings []"=w1671:string[], "Value"=w1670:u16)  [unwired: 2 in, 2 out]
                        n1160 = Index Array "索引数组"(array=w1671, index=w1670) -> (element=w1669:string)
                        n1161 = call "数据库保存子vi.vi"("#1 Pressure"=w1665, "Part No."=w1661, "Result"=w1675, "2D Code"=w1660, "Person"=w1669, "#1 Leakage"=w1666, "Serial No."=w1659, "Time"=w1667) -> ()  [unwired: 4 in]
                        n1162 = call <vilib>:"Space Constant.vi"() -> ("String"=w1664:string)
                        n1163 = Concatenate Strings(w1667, w1664, w1665, w1664, w1666) -> (w1663:string)
                        n1164 = Write to Text File "写入文本文件"(file (use dialog)=path "d:/data/负压值A.txt" ("文件（使用对话框）"), text=w1663) -> ()  [unwired: 2 in, 3 out]
                      }
                      frame #4 {
                        n1165 = case shown="假" w1728 {
                          frame False {
                            w1729 = u16 0 ("合格次数")
                            n1166 = local write "检测次数A"(w1729) -> ()
                            n1167 = local write "合格次数A"(w1729) -> ()
                          }
                          frame True {
                          }
                        }
                      }
                    }
                  }
                  frame 2 {
                    n1168 = flat-sequence {
                      tunnel: w1730 -> [w1748]
                      frame #0 {
                        w1739 = path "d:/data/序列号A.txt"  # 文件（使用对话框）
                        w1742 = u16 2  # y
                        w1745 = i16 3  # 精度(6)
                        w1744 = i16 6  # 宽度(-)
                        w1747 = i16 3  # 精度(6)
                        w1746 = i16 7  # 宽度(-)
                        n1169 = case shown="真" w1748 {
                          tunnel: [w1756 w1768] -> w1731
                          tunnel: [w1753 w1769] -> w1732
                          frame False {
                            n1170 = local read "实时漏率A"() -> (w1755:dbl)
                            n1171 = Equal To 0?(x=w1755) -> (x = 0?=w1754:bool)
                            n1172 = case shown="假" w1754 {
                              tunnel: [w1758 99999.0] -> w1756
                              tunnel: [w1757 w1759] -> w1753
                              frame False {
                                n1173 = local read "结果压力"() -> (w1757:dbl)
                                n1174 = local read "实时漏率A"() -> (w1758:dbl)
                              }
                              frame True {
                                n1175 = local read "实时压力A"() -> (w1759:dbl)
                              }
                            }
                          }
                          frame True {
                            w1765 = FALSE ("校准时间到")
                            n1176 = local write "scan A"(TRUE ("Scan A")) -> ()
                            n1177 = local write "2D Code_A"("") -> ()
                            n1178 = local write "A OK Sample Req. (2nd)"(w1765) -> ()
                            n1179 = local write "A Cal. Time"(w1765) -> ()
                            n1180 = Read from Text File(file (use dialog)=path "D:/data/Print_Cal_OK_A.txt" ("文件（使用对话框）")) -> (text=w1761:string)  [unwired: 3 in, 3 out]
                            n1181 = call <vilib>:"System Exec.vi"("run minimized? (F)"=TRUE, "wait until completion? (T)"=FALSE, "command line"=w1761) -> ()  [unwired: 5 in, 4 out]
                            n1182 = local read "实时漏率A"() -> (w1768:dbl)
                            n1183 = local read "结果压力"() -> (w1769:dbl)
                          }
                        }
                        n1184 = local read "合格次数A"() -> (w1743:u16)
                        n1185 = Number To Fractional String "数值至小数字符串转换"(number=w1732, width (-)=w1746, precision (6)=w1747) -> (F-format string=w1749:string)  [unwired: 1 in]
                        n1186 = Number To Fractional String "数值至小数字符串转换"(number=w1731, width (-)=w1744, precision (6)=w1745) -> (F-format string=w1750:string)  [unwired: 1 in]
                        n1187 = Equal? "等于？"(x=w1743, y=w1742) -> (x = y?=w1741:bool)
                        n1188 = local read "压力单位"() -> (w1751:string)
                        n1189 = local read "泄漏单位"() -> (w1752:string)
                        n1190 = case "条件结构" shown="真" w1741 {
                          tunnel: ["NG" "OK"] -> w1740
                          frame False {
                          }
                          frame True {
                          }
                        }
                        n1191 = Concatenate Strings "连接字符串"(w1749, w1751) -> (w1734:string)
                        n1192 = Concatenate Strings "连接字符串"(w1750, w1752) -> (w1733:string)
                        n1193 = Read from Text File "读取文本文件"(file (use dialog)=w1739) -> (text=w1738:string)  [unwired: 3 in, 3 out]
                        n1194 = call "数据库插入子vi.vi"("result"=w1740, "2_Leakage"=w1733, "2_Pressure"=w1734, "Serial_No"=w1738) -> ()  [unwired: 8 in]
                        n1195 = call <vilib>:"Space Constant.vi"() -> ("String"=w1736:string)
                        n1196 = Concatenate Strings(w1734, w1736, w1733) -> (w1735:string)
                        n1197 = Write to Text File "写入文本文件"(file (use dialog)=path "d:/data/正压值A.txt" ("文件（使用对话框）"), text=w1735) -> ()  [unwired: 2 in, 3 out]
                      }
                      frame #1 {
                        n1198 = Wait (ms)(milliseconds to wait=u32 2000 ("等待时间（毫秒）")) -> ()  [unwired: 1 out]
                      }
                      frame #2 {
                        w1775 = u16 0 ("合格次数")
                        n1199 = local write "检测次数A"(w1775) -> ()
                        n1200 = local write "合格次数A"(w1775) -> ()
                        n1201 = Write to Text File "写入文本文件"(file (use dialog)=path "d:/data/正压值A.txt" ("文件（使用对话框）"), text="") -> ()  [unwired: 2 in, 3 out]
                      }
                    }
                  }
                }
              }
              frame #3 {
                n1202 = call "数据库读取.vi"() -> ("当日合格数"=w1776:i32, "当天总数"=w1777:i32, "Data"=w1778:string[][])  [unwired: 9 in]
                n1203 = property on="A List" class="Tbl (严格)"("Value"=w1778) -> ()  [unwired: 2 in, 2 out]
                n1204 = local write "Total Today A"(w1777) -> ()
                n1205 = local write "OK Today A"(w1776) -> ()
              }
              frame #4 {
                n1206 = local write "合格状态左"(2.0) -> ()
              }
            }
          }
        }
      }
      frame 2, Default {
        n1207 = flat-sequence {
          tunnel: w1781 -> [w1783]
          tunnel: [w1783] -> w1780
          tunnel: w1780 -> [w1784]
          frame #0 {
            n1208 = Wait (ms)(milliseconds to wait=u32 3000 ("等待时间（毫秒）")) -> ()  [unwired: 1 out]
          }
          frame #1 {
            n1209 = case shown="假" w1784 {
              frame False {
                n1210 = local write "合格状态左"(0.0 ("合格状态")) -> ()
              }
              frame True {
              }
            }
          }
        }
      }
    }
    "数字不跳动，表示软件死机 A" <- w1376
  }
  n1211 = flat-sequence {
    frame #0 {
      n1212 = local write "扫码在线过程"(2.0 ("扫码在线过程")) -> ()
    }
    frame #1 {
      n1213 = while {
        stop <- FALSE stop-if-true
        n1214 = Wait (ms)(milliseconds to wait=u32 10 ("等待时间（毫秒）")) -> ()  [unwired: 1 out]
        n1215 = case shown="假" "A复位" {
          frame False {
          }
          frame True {
            w1806 = u16 0 ("合格次数")
            n1216 = local write "scan A"(FALSE ("右工位扫码合格")) -> ()
            n1217 = local write "合格次数A"(w1806) -> ()
            n1218 = local write "检测次数A"(w1806) -> ()
            n1219 = local write "合格状态左"(w1806) -> ()
          }
        }
        n1220 = case shown="假" "B复位" {
          frame False {
          }
          frame True {
            w1804 = u16 0 ("合格次数")
            n1221 = local write "scan B"(FALSE ("右工位扫码合格")) -> ()
            n1222 = local write "合格状态右"(w1804) -> ()
            n1223 = local write "检测次数B"(w1804) -> ()
            n1224 = local write "合格次数B"(w1804) -> ()
          }
        }
        n1225 = local read "B自动/手动_Automatic/Manual_Automatique/Manual"() -> (w1792:bool)
        n1226 = local read "A自动/手动_Automatic/Manual_Automatique/Manual"() -> (w1793:bool)
        n1227 = case shown="假" w1792 {
          frame True {
            w1798 = T2."Enabled" ("禁用")
            n1228 = property on="B封堵_Blocking_Bloquant：后退_Back_Arrière/前进_forward_avant" class="Bool (严格)"("DisabledEnum"=w1798) -> ()  [unwired: 2 in, 2 out]
            n1229 = property on="B盖章_Stamp_Timbre：后退_Back_Arrière/前进_forward_avant" class="Bool (严格)"("DisabledEnum"=w1798) -> ()  [unwired: 2 in, 2 out]
            n1230 = property on="B夹紧_Clamping_Serrage：后退_Back_Arrière/前进_forward_avant" class="Bool (严格)"("DisabledEnum"=w1798) -> ()  [unwired: 2 in, 2 out]
            n1231 = property on="B移载_Transfer_Transfert：后退_Back_Arrière/前进_forward_avant" class="Bool (严格)"("DisabledEnum"=w1798) -> ()  [unwired: 2 in, 2 out]
          }
          frame False {
            w1799 = FALSE ("右工位扫码合格")
            w1800 = T2."Disabled and Grayed Out" ("禁用")
            n1232 = property on="B盖章_Stamp_Timbre：后退_Back_Arrière/前进_forward_avant" class="Bool (严格)"("DisabledEnum"=w1800, "Value"=w1799) -> ()  [unwired: 2 in, 2 out]
            n1233 = property on="B夹紧_Clamping_Serrage：后退_Back_Arrière/前进_forward_avant" class="Bool (严格)"("DisabledEnum"=w1800, "Value"=w1799) -> ()  [unwired: 2 in, 2 out]
            n1234 = property on="B移载_Transfer_Transfert：后退_Back_Arrière/前进_forward_avant" class="Bool (严格)"("DisabledEnum"=w1800, "Value"=w1799) -> ()  [unwired: 2 in, 2 out]
            n1235 = property on="B封堵_Blocking_Bloquant：后退_Back_Arrière/前进_forward_avant" class="Bool (严格)"("DisabledEnum"=w1800, "Value"=w1799) -> ()  [unwired: 2 in, 2 out]
          }
        }
        n1236 = case shown="假" w1793 {
          frame True {
            w1801 = T2."Enabled" ("禁用")
            n1237 = property on="A盖章_Stamp_Timbre：后退_Back_Arrière/前进_forward_avant" class="Bool (严格)"("DisabledEnum"=w1801) -> ()  [unwired: 2 in, 2 out]
            n1238 = property on="A夹紧_Clamping_Serrage：后退_Back_Arrière/前进_forward_avant" class="Bool (严格)"("DisabledEnum"=w1801) -> ()  [unwired: 2 in, 2 out]
            n1239 = property on="A移载_Transfer_Transfert：后退_Back_Arrière/前进_forward_avant" class="Bool (严格)"("DisabledEnum"=w1801) -> ()  [unwired: 2 in, 2 out]
            n1240 = property on="A封堵_Blocking_Bloquant：后退_Back_Arrière/前进_forward_avant" class="Bool (严格)"("DisabledEnum"=w1801) -> ()  [unwired: 2 in, 2 out]
          }
          frame False {
            w1802 = FALSE ("右工位扫码合格")
            w1803 = T2."Disabled and Grayed Out" ("禁用")
            n1241 = property on="A盖章_Stamp_Timbre：后退_Back_Arrière/前进_forward_avant" class="Bool (严格)"("DisabledEnum"=w1803, "Value"=w1802) -> ()  [unwired: 2 in, 2 out]
            n1242 = property on="A夹紧_Clamping_Serrage：后退_Back_Arrière/前进_forward_avant" class="Bool (严格)"("DisabledEnum"=w1803, "Value"=w1802) -> ()  [unwired: 2 in, 2 out]
            n1243 = property on="A移载_Transfer_Transfert：后退_Back_Arrière/前进_forward_avant" class="Bool (严格)"("DisabledEnum"=w1803, "Value"=w1802) -> ()  [unwired: 2 in, 2 out]
            n1244 = property on="A封堵_Blocking_Bloquant：后退_Back_Arrière/前进_forward_avant" class="Bool (严格)"("DisabledEnum"=w1803, "Value"=w1802) -> ()  [unwired: 2 in, 2 out]
          }
        }
      }
      n1245 = while {
        shift-right: [w1810] -> _
        shift-left: T4."Open" -> [w1816]
        shift-right: [w1814] -> w1789
        shift-left: _ -> [w1809]
        tunnel: "错误输入（无错误）" -> [w1813]
        tunnel: [w1812] -> w1788
        stop <- w1815 stop-if-true
        n1246 = Wait (ms)(milliseconds to wait=u32 100 ("等待时间（毫秒）")) -> ()  [unwired: 1 out]
        n1247 = case shown="假" "扫描枪重连" {
          tunnel: w1816 -> [w1827 _]
          tunnel: [w1826 _] -> w1815
          tunnel: [w1825 w2006] -> w1814
          tunnel: w1813 -> [w1824 w2004]
          tunnel: [w1823 w2005] -> w1812
          tunnel: [w1822 T4."Write LON"] -> w1810
          tunnel: w1809 -> [w1821 _]
          frame False {
            n1248 = case shown="\"Read\"" w1827 {
              tunnel: [w1836 T4."Loop" T4."Loop" w1865 w1882 T4."Loop" T4."Exit" w1997] -> w1822
              tunnel: [_ _ _ _ _ _ TRUE FALSE] -> w1826
              tunnel: [w1834 w1840 w1863 w1869 w1881 w1983 w1990 w2001] -> w1825
              tunnel: w1821 -> [w1834 _ w1863 w1869 w1887 w1986 w1990 w2001]
              tunnel: w1824 -> [w1835 w1844 w1862 w1868 w1891 w1987 w1989 w2000]
              tunnel: [w1835 w1843 w1861 w1867 w1880 w1985 w1988 w2000] -> w1823
              frame "Init", Default {
                n1249 = Unbundle By Name(w1835) -> ("status"=w1837:bool)
                n1250 = case shown="假" w1837 {
                  tunnel: [T4."Loop" T4."Exit"] -> w1836
                  frame False {
                  }
                  frame True {
                  }
                }
              }
              frame "Open" {
                n1251 = case shown="\"Client\"" enum16{"Server", "Client"}."Client" ("类型") {
                  tunnel: "192.168.2.2" ("IP") -> [_ w1856]
                  tunnel: w1844 -> [w1848 w1855]
                  tunnel: [w1847 w1854] -> w1843
                  tunnel: u16 9004 ("Port") -> [w1850 w1853]
                  tunnel: [w1849 w1851] -> w1840
                  frame "Server", Default {
                    n1252 = call <vilib>:"TCP Listen.vi"("error in (no error)"=w1848, "port"=w1850) -> ("error out"=w1847:errorcluster, "connection ID"=w1849:refnum<k5>)  [unwired: 5 in, 3 out]
                  }
                  frame "Client" {
                    n1253 = TCP Open Connection(address=w1856, remote port or service name=w1853, timeout ms (60000)=1000 ("超时毫秒(60000)"), error in (no error)=w1855) -> (connection ID=w1851:refnum<k5>, error out=w1854:errorcluster)  [unwired: 1 in]
                  }
                }
              }
              frame "Write LOFF" {
                n1254 = Concatenate Strings("LOFF" ("写"), "\r") -> (w1859:string)
                n1255 = TCP Write(connection ID=w1863, data in=w1859, error in (no error)=w1862, 9:100 ("超时毫秒(25000)")) -> (error out=w1861:errorcluster)  [unwired: 2 out]
              }
              frame "Write LON" {
                n1256 = flat-sequence {
                  tunnel: [w1875] -> w1866
                  tunnel: w1869 -> [w1877]
                  tunnel: w1868 -> [w1876]
                  tunnel: [w1879] -> w1867
                  tunnel: w1866 -> [w1879]
                  tunnel: [T4."Read"] -> w1865
                  frame #0 {
                    n1257 = Wait (ms)(milliseconds to wait=u32 100 ("等待时间（毫秒）")) -> ()  [unwired: 1 out]
                    n1258 = Concatenate Strings("LON" ("写"), "\r") -> (w1873:string)
                    n1259 = TCP Write(connection ID=w1877, data in=w1873, error in (no error)=w1876, 9:100 ("超时毫秒(25000)")) -> (error out=w1875:errorcluster)  [unwired: 2 out]
                  }
                  frame #1 {
                  }
                }
              }
              frame "Read" {
                n1260 = TCP Read(connection ID=w1887, bytes to read=100 ("读取的字节"), error in (no error)=w1891, 7:T5."Immediate" ("模式（标准）"), 9:100 ("超时毫秒(25000)")) -> (connection ID out=w1881:refnum<k5>, data out=w1886:string, error out=w1880:errorcluster)
                n1261 = String Length(string=w1886) -> (length=w1885:i32)
                n1262 = Greater?(x=w1885, y=10) -> (0:w1883:bool)
                n1263 = case shown="真" w1883 {
                  tunnel: w1886 -> [_ w1898]
                  tunnel: [T4."Write LON" w1897] -> w1882
                  tunnel: w1880 -> [_ w1896]
                  tunnel: w1881 -> [_ w1895]
                  tunnel: w1881 -> [_ w1894]
                  tunnel: w1880 -> [_ w1893]
                  frame False {
                  }
                  frame True {
                    n1264 = flat-sequence {
                      tunnel: w1898 -> [w1909]
                      tunnel: w1896 -> [w1908]
                      tunnel: w1895 -> [w1907]
                      tunnel: w1894 -> [w1906]
                      tunnel: w1893 -> [w1905]
                      tunnel: [T4."Loop"] -> w1897
                      frame #0 {
                        n1265 = local read "A NG Sample Req.（1st)"() -> (w1903:bool)
                        n1266 = local read "A OK Sample Req. (2nd)"() -> (w1902:bool)
                        n1267 = local read "B OK Sample Req. (2nd)"() -> (w1899:bool)
                        n1268 = local read "B NG Sample Req.（1st)"() -> (w1900:bool)
                        n1269 = Or "或"(x=w1903, y=w1902) -> (x .or. y?=w1904:bool)
                        n1270 = Or(x=w1899, y=w1900) -> (x .or. y?=w1901:bool)
                        n1271 = case shown="真" w1904 {
                          tunnel: w1909 -> [w1949 w1965]
                          tunnel: w1908 -> [w1948 w1967]
                          tunnel: w1907 -> [w1947 w1966]
                          frame False {
                            n1272 = call "扫码查询.vi"("2D_Code"=w1949) -> ("Match"=w1946:i32)  [unwired: 9 in, 1 out]
                            n1273 = case shown="1" w1946 {
                              tunnel: w1949 -> [_ w1952]
                              tunnel: w1948 -> [_ w1951]
                              tunnel: w1947 -> [_ w1950]
                              frame 0, Default {
                              }
                              frame 1 {
                                n1274 = flat-sequence {
                                tunnel: w1952 -> [w1953]
                                tunnel: w1951 -> [w1957]
                                tunnel: w1950 -> [w1956]
                                frame #0 {
                                n1275 = local write "2D Code_A"(w1953) -> ()
                                n1276 = call "已贴标签A.vi"("2D_Code"=w1953) -> ()  [unwired: 11 in]
                                "Scan OK A" <- TRUE ("右工位扫码合格")
                                }
                                frame #1 {
                                n1277 = Wait (ms)(milliseconds to wait=u32 1000 ("等待时间（毫秒）")) -> ()  [unwired: 1 out]
                                }
                                frame #2 {
                                n1278 = local write "scan A"(FALSE ("右工位扫码合格")) -> ()
                                n1279 = local write "Scan OK A"(FALSE ("Scan OK A")) -> ()
                                n1280 = Concatenate Strings("LOFF" ("写"), "\r") -> (w1960:string)
                                n1281 = TCP Write(connection ID=w1956, data in=w1960, error in (no error)=w1957, 9:100 ("超时毫秒(25000)")) -> ()  [unwired: 3 out]
                                }
                                }
                              }
                            }
                          }
                          frame True {
                            n1282 = call "扫码查询.vi"("2D_Code"=w1965) -> ("Match"=w1964:i32)  [unwired: 9 in, 1 out]
                            n1283 = case shown="1" w1964 {
                              tunnel: w1965 -> [_ w1968]
                              tunnel: w1967 -> [_ w1970]
                              tunnel: w1966 -> [_ w1969]
                              frame 0, Default {
                              }
                              frame 1 {
                                n1284 = flat-sequence {
                                tunnel: w1968 -> [w1972]
                                tunnel: w1970 -> [w1976]
                                tunnel: w1969 -> [w1975]
                                frame #0 {
                                n1285 = call "已贴标签A.vi"("2D_Code"=w1972) -> ()  [unwired: 11 in]
                                n1286 = local write "2D Code_A"(w1972) -> ()
                                n1287 = local write "Scan OK A"(TRUE ("右工位扫码合格")) -> ()
                                }
                                frame #1 {
                                n1288 = Wait (ms)(milliseconds to wait=u32 1000 ("等待时间（毫秒）")) -> ()  [unwired: 1 out]
                                }
                                frame #2 {
                                n1289 = local write "scan A"(FALSE ("右工位扫码合格")) -> ()
                                n1290 = local write "Scan OK A"(FALSE ("Scan OK A")) -> ()
                                n1291 = Concatenate Strings("LOFF" ("写"), "\r") -> (w1979:string)
                                n1292 = TCP Write(connection ID=w1975, data in=w1979, error in (no error)=w1976, 9:100 ("超时毫秒(25000)")) -> ()  [unwired: 3 out]
                                }
                                frame #3 {
                                }
                                }
                              }
                            }
                          }
                        }
                        n1293 = case shown="真" w1901 {
                          tunnel: w1909 -> [w1911 w1929]
                          tunnel: w1906 -> [w1913 w1931]
                          tunnel: w1905 -> [w1912 w1930]
                          frame False {
                            n1294 = call "扫码查询B.vi"("2D_Code"=w1911) -> ("Match"=w1910:i32)  [unwired: 9 in, 1 out]
                            n1295 = case shown="1" w1910 {
                              tunnel: w1911 -> [_ w1916]
                              tunnel: w1913 -> [_ w1915]
                              tunnel: w1912 -> [_ w1914]
                              frame 0, Default {
                              }
                              frame 1 {
                                n1296 = flat-sequence {
                                tunnel: w1916 -> [w1917]
                                tunnel: w1915 -> [w1921]
                                tunnel: w1914 -> [w1920]
                                frame #0 {
                                n1297 = call "已贴标签B.vi"("2D_Code"=w1917) -> ()  [unwired: 11 in]
                                n1298 = local write "2D Code_B"(w1917) -> ()
                                "Scan OK B" <- TRUE ("右工位扫码合格")
                                }
                                frame #1 {
                                n1299 = Wait (ms)(milliseconds to wait=u32 1000 ("等待时间（毫秒）")) -> ()  [unwired: 1 out]
                                }
                                frame #2 {
                                n1300 = local write "Scan OK B"(FALSE ("Scan OK B")) -> ()
                                n1301 = local write "scan B"(FALSE ("右工位扫码合格")) -> ()
                                n1302 = Concatenate Strings("LOFF" ("写"), "\r") -> (w1924:string)
                                n1303 = TCP Write(connection ID=w1921, data in=w1924, error in (no error)=w1920, 9:100 ("超时毫秒(25000)")) -> ()  [unwired: 3 out]
                                }
                                }
                              }
                            }
                          }
                          frame True {
                            n1304 = call "扫码查询B.vi"("2D_Code"=w1929) -> ("Match"=w1928:i32)  [unwired: 9 in, 1 out]
                            n1305 = case shown="1" w1928 {
                              tunnel: w1929 -> [_ w1932]
                              tunnel: w1930 -> [_ w1934]
                              tunnel: w1931 -> [_ w1933]
                              frame 0, Default {
                              }
                              frame 1 {
                                n1306 = flat-sequence {
                                tunnel: w1932 -> [w1935]
                                tunnel: w1934 -> [w1940]
                                tunnel: w1933 -> [w1939]
                                frame #0 {
                                n1307 = call "已贴标签B.vi"("2D_Code"=w1935) -> ()  [unwired: 11 in]
                                n1308 = local write "2D Code_B"(w1935) -> ()
                                n1309 = local write "Scan OK B"(TRUE ("右工位扫码合格")) -> ()
                                }
                                frame #1 {
                                n1310 = Wait (ms)(milliseconds to wait=u32 1000 ("等待时间（毫秒）")) -> ()  [unwired: 1 out]
                                }
                                frame #2 {
                                n1311 = local write "scan B"(FALSE ("右工位扫码合格")) -> ()
                                n1312 = local write "Scan OK B"(FALSE ("Scan OK A")) -> ()
                                n1313 = Concatenate Strings("LOFF" ("写"), "\r") -> (w1943:string)
                                n1314 = TCP Write(connection ID=w1939, data in=w1943, error in (no error)=w1940, 9:100 ("超时毫秒(25000)")) -> ()  [unwired: 3 out]
                                }
                                frame #3 {
                                }
                                }
                              }
                            }
                          }
                        }
                      }
                      frame #1 {
                      }
                    }
                  }
                }
              }
              frame "Close" {
                n1315 = TCP Close Connection(connection ID=w1986, error in (no error)=w1987) -> (connection ID out=w1983:refnum<k5>, error out=w1985:errorcluster)  [unwired: 1 in]
              }
              frame "Exit" {
                n1316 = TCP Close Connection(connection ID=w1990, error in (no error)=w1989) -> (error out=w1988:errorcluster)  [unwired: 1 in, 1 out]
              }
              frame "Loop" {
                n1317 = local read "scan A"() -> (w1994:bool)
                n1318 = local read "scan B"() -> (w1993:bool)
                n1319 = Not(x=w1994) -> (.not. x?=w1995:bool)
                n1320 = Not(x=w1993) -> (.not. x?=w1996:bool)
                n1321 = And(x=w1995, y=w1996) -> (x .and. y?=w1998:bool)
                n1322 = case shown="真" w1998 {
                  tunnel: [T4."Write LON" T4."Write LOFF"] -> w1997
                  frame False {
                  }
                  frame True {
                  }
                }
              }
            }
            n1323 = Type Cast(type=0, x=w1821) -> (*(type *) &x=w1819:i32)
            n1324 = Not Equal To 0?(x=w1819) -> (x != 0?=w1817:bool)
            "Scanner" <- w1817
            "Scanner" <- w1817
            n1325 = case shown="2" "扫码在线过程" {
              tunnel: w1817 -> [_ w1830 w1832]
              frame 1 {
                n1326 = local write "扫码在线过程"(2.0 ("扫码在线过程")) -> ()
                n1327 = One Button Dialog(message="扫描枪离线，先关闭此软件，请使用AutoID Network Navigator (CHS)进行初始化后再打开此软件。\nThe Scanner is offline, close this window. Please use AutoID Network Navigator (CHS) to initialize and then reopen this window.\nLe scanner est hors ligne, fermez cette fenêtre. Utilisez AutoID Network Navigator (CHS) pour initialiser, puis rouvrir cette fenêtre." ("消息")) -> ()  [unwired: 1 in, 1 out]
              }
              frame 0, Default {
                n1328 = case shown="真" w1830 {
                  frame False {
                    n1329 = local write "扫码在线过程"(1.0 ("扫码在线过程")) -> ()
                  }
                  frame True {
                  }
                }
              }
              frame 2 {
                n1330 = case shown="真" w1832 {
                  frame False {
                  }
                  frame True {
                    n1331 = local write "扫码在线过程"(0.0 ("扫码在线过程")) -> ()
                  }
                }
              }
            }
          }
          frame True {
            n1332 = case shown="\"Client\"" enum16{"Server", "Client"}."Client" ("类型") {
              tunnel: "192.168.2.2" ("IP") -> [_ w2020]
              tunnel: w2004 -> [w2012 w2019]
              tunnel: [w2011 w2018] -> w2005
              tunnel: u16 9004 ("Port") -> [w2014 w2017]
              tunnel: [w2013 w2015] -> w2006
              frame "Server", Default {
                n1333 = call <vilib>:"TCP Listen.vi"("error in (no error)"=w2012, "port"=w2014) -> ("error out"=w2011:errorcluster, "connection ID"=w2013:refnum<k5>)  [unwired: 5 in, 3 out]
              }
              frame "Client" {
                n1334 = TCP Open Connection(address=w2020, remote port or service name=w2017, timeout ms (60000)=1000 ("超时毫秒(60000)"), error in (no error)=w2019) -> (connection ID=w2015:refnum<k5>, error out=w2018:errorcluster)  [unwired: 1 in]
              }
            }
          }
        }
      }
      n1335 = TCP Close Connection(connection ID=w1789, error in (no error)=w1788) -> (error out=→"错误输出":errorcluster)  [unwired: 1 in, 1 out]
    }
  }
  n1336 = flat-sequence {
    tunnel: [w2026] -> w31
    tunnel: [w2025] -> w30
    tunnel: w31 -> [w2033]
    tunnel: w30 -> [w2032]
    tunnel: [w2031] -> w29
    tunnel: [w2030] -> w28
    tunnel: [w2040] -> w27
    tunnel: [w2039] -> w26
    tunnel: w29 -> [w2038]
    tunnel: w28 -> [w2037]
    tunnel: w27 -> [w2065]
    tunnel: w26 -> [w2056]
    tunnel: [w2060] -> w25
    tunnel: [w2061] -> w24
    tunnel: w25 -> [w2073]
    tunnel: w24 -> [w2072]
    tunnel: [w2071] -> w23
    tunnel: [w2070] -> w22
    tunnel: w23 -> [w2101]
    tunnel: w22 -> [w2097]
    tunnel: [w2100] -> w21
    tunnel: [w2099] -> w20
    tunnel: w21 -> [w2122]
    tunnel: w20 -> [w2121]
    tunnel: [w2119] -> w15
    tunnel: [w2118] -> w14
    tunnel: [w2144] -> w19
    tunnel: [w2143] -> w18
    tunnel: w15 -> [w2141]
    tunnel: w14 -> [w2140]
    tunnel: w19 -> [w2151]
    tunnel: w18 -> [w2150]
    tunnel: [w2149] -> w17
    tunnel: [w2148] -> w16
    tunnel: w17 -> [w2155]
    tunnel: w16 -> [w2154]
    frame #0 {
      n1337 = property on="ATEQ F620 A (Restart Software to Active)" class="VISAName"() -> ("Label.Text"=w2028:string)  [unwired: 2 in, 2 out]
      n1338 = call <vilib>:"Open Config Data.vi"("create file if necessary (T)"=TRUE, "configuration file path"=path "D:/data/Setup.ini") -> ("error out"=w2021:errorcluster, "refnum"=w2022:T3)  [unwired: 7 in, 1 out]
      n1339 = call-poly <vilib>:"Read Key.vi"("section"="Setup", "error in (no error)"=w2021, "key"=w2028, "refnum"=w2022) -> ("error out"=w2025:errorcluster, "value"=w2027:string, "refnum out"=w2026:T3)  [unwired: 4 in, 1 out]
      n1340 = property on="ATEQ F620 A (Restart Software to Active)" class="VISAName"("Value"=w2027) -> ()  [unwired: 2 in, 2 out]
    }
    frame #1 {
      n1341 = property on="ATEQ F620 B (Restart Software to Active)" class="VISAName"() -> ("Label.Text"=w2035:string)  [unwired: 2 in, 2 out]
      n1342 = call-poly <vilib>:"Read Key.vi"("section"="Setup", "error in (no error)"=w2032, "key"=w2035, "refnum"=w2033) -> ("error out"=w2030:errorcluster, "value"=w2036:string, "refnum out"=w2031:T3)  [unwired: 4 in, 1 out]
      n1343 = property on="ATEQ F620 B (Restart Software to Active)" class="VISAName"("Value"=w2036) -> ()  [unwired: 2 in, 2 out]
    }
    frame #2 {
      n1344 = for {
        N: 25 -> [_]
        tunnel: w2038 -> [w2055]
        tunnel: [w2053] -> w2040
        tunnel: w2037 -> [w2052]
        tunnel: [w2051] -> w2039
        i -> [w2045]
        n1345 = Increment(x=w2045) -> (x+1=w2047:i32)
        n1346 = Number To Decimal String(number=w2047) -> (decimal integer string=w2049:string)  [unwired: 1 in]
        n1347 = Concatenate Strings("ATEQ程序号" ("字符串"), w2049) -> (w2048:string)
        n1348 = call-poly <vilib>:"Read Key.vi"("section"="Setup", "error in (no error)"=w2052, "key"=w2048, "refnum"=w2055) -> ("error out"=w2051:errorcluster, "value"=w2042:string, "refnum out"=w2053:T3)  [unwired: 4 in, 1 out]
        n1349 = Replace Array Subset(array="参数设置/Setup/Coup monté", new element=w2042, index (row)=w2045, index (col)=2 ("索引 (列)")) -> (w2044:string[][])
        n1350 = local write "参数设置/Setup/Coup monté"(w2044) -> ()
      }
    }
    frame #3 {
      w2069 = "Setup" ("section")
      n1351 = property on="Calitration Period (Hours)" class="AbsTime (严格)"() -> ("Label.Text"=w2068:string)  [unwired: 2 in, 2 out]
      n1352 = property on="2nd Shift" class="AbsTime (严格)"() -> ("Label.Text"=w2067:string)  [unwired: 2 in, 2 out]
      n1353 = call-poly <vilib>:"Read Key.vi"("section"=w2069, "error in (no error)"=w2056, "key"=w2068, "refnum"=w2065) -> ("error out"=w2062:errorcluster, "value"=w2059:string, "refnum out"=w2064:T3)  [unwired: 4 in, 1 out]
      n1354 = property on="3th Shift" class="AbsTime (严格)"() -> ("Label.Text"=w2066:string)  [unwired: 2 in, 2 out]
      n1355 = property on="Calitration Period (Hours)" class="AbsTime (严格)"("NumText.Text"=w2059) -> ()  [unwired: 2 in, 2 out]
      n1356 = call-poly <vilib>:"Read Key.vi"("section"=w2069, "error in (no error)"=w2062, "key"=w2067, "refnum"=w2064) -> ("error out"=w2061:errorcluster, "value"=w2058:string, "refnum out"=w2063:T3)  [unwired: 4 in, 1 out]
      n1357 = property on="2nd Shift" class="AbsTime (严格)"("NumText.Text"=w2058) -> ()  [unwired: 2 in, 2 out]
      n1358 = call-poly <vilib>:"Read Key.vi"("section"=w2069, "key"=w2066, "refnum"=w2063) -> ("value"=w2057:string, "refnum out"=w2060:T3)  [unwired: 5 in, 2 out]
      n1359 = property on="3th Shift" class="AbsTime (严格)"("NumText.Text"=w2057) -> ()  [unwired: 2 in, 2 out]
    }
    frame #4 {
      n1360 = for {
        N: 25 -> [_]
        tunnel: w2073 -> [w2088]
        tunnel: [w2086] -> w2070
        tunnel: w2072 -> [w2085]
        tunnel: [w2084] -> w2071
        i -> [w2078]
        w2077 = 1 ("索引 (列)")
        n1361 = Increment(x=w2078) -> (x+1=w2082:i32)
        n1362 = Number To Decimal String(number=w2082) -> (decimal integer string=w2081:string)  [unwired: 1 in]
        n1363 = local read "参数设置/Setup/Coup monté"() -> (w2076:string[][])
        n1364 = Concatenate Strings("客户型号" ("字符串"), w2081) -> (w2080:string)
        n1365 = call-poly <vilib>:"Read Key.vi"("section"="Setup", "error in (no error)"=w2085, "key"=w2080, "refnum"=w2088) -> ("error out"=w2084:errorcluster, "value"=w2079:string, "refnum out"=w2086:T3)  [unwired: 4 in, 1 out]
        n1366 = Replace Array Subset(array=w2076, new element=w2079, index (row)=w2078, index (col)=w2077) -> (w2075:string[][])
        n1367 = Index Array(array=w2075, index (row)=w2078, index (col)=w2077) -> ()  [unwired: 1 out]
        n1368 = local write "参数设置/Setup/Coup monté"(w2075) -> ()
      }
    }
    frame #5 {
      n1369 = for {
        N: 25 -> [_]
        tunnel: w2097 -> [w2117]
        tunnel: [w2115] -> w2100
        tunnel: w2101 -> [w2114]
        tunnel: [w2113] -> w2099
        tunnel: [w2105] -> w2098 mode=indexing
        i -> [w2107]
        w2106 = 0 ("索引 (列)")
        n1370 = Increment(x=w2107) -> (x+1=w2111:i32)
        n1371 = Number To Decimal String(number=w2111) -> (decimal integer string=w2110:string)  [unwired: 1 in]
        n1372 = local read "参数设置/Setup/Coup monté"() -> (w2104:string[][])
        n1373 = Concatenate Strings("产品型号" ("字符串"), w2110) -> (w2109:string)
        n1374 = call-poly <vilib>:"Read Key.vi"("section"="Setup", "error in (no error)"=w2114, "key"=w2109, "refnum"=w2117) -> ("error out"=w2113:errorcluster, "value"=w2108:string, "refnum out"=w2115:T3)  [unwired: 4 in, 1 out]
        n1375 = Replace Array Subset(array=w2104, new element=w2108, index (row)=w2107, index (col)=w2106) -> (w2103:string[][])
        n1376 = Index Array(array=w2103, index (row)=w2107, index (col)=w2106) -> (element=w2105:string)
        n1377 = local write "参数设置/Setup/Coup monté"(w2103) -> ()
      }
      n1378 = property on="Part No. A" class="Ring (严格)"("Strings []"=w2098) -> ("Strings []"=w2094:string[], "Value"=w2093:u16)  [unwired: 2 in, 2 out]
      n1379 = property on="Part No. B" class="Ring (严格)"("Strings []"=w2098) -> ("Strings []"=w2091:string[], "Value"=w2090:u16)  [unwired: 2 in, 2 out]
      n1380 = Index Array(array=w2094, index=w2093) -> (element=w2092:string)
      n1381 = Index Array(array=w2091, index=w2090) -> (element=w2089:string)
      n1382 = Write to Text File(file (use dialog)=path "D:/data/协众产品号A.txt" ("文件（使用对话框）"), text=w2092) -> ()  [unwired: 2 in, 3 out]
      n1383 = Write to Text File(file (use dialog)=path "D:/data/协众产品号B.txt" ("文件（使用对话框）"), text=w2089) -> ()  [unwired: 2 in, 3 out]
    }
    frame #6 {
      n1384 = for {
        N: 25 -> [_]
        tunnel: w2122 -> [w2139]
        tunnel: w2121 -> [w2137]
        tunnel: [w2129] -> w2120 mode=indexing
        tunnel: [w2125] -> w2119
        tunnel: [w2124] -> w2118
        i -> [w2131]
        w2130 = 3 ("索引 (列)")
        n1385 = Wait (ms)(milliseconds to wait=u32 500 ("等待时间（毫秒）")) -> ()  [unwired: 1 out]
        n1386 = Increment(x=w2131) -> (x+1=w2135:i32)
        n1387 = Number To Decimal String(number=w2135) -> (decimal integer string=w2134:string)  [unwired: 1 in]
        n1388 = local read "参数设置/Setup/Coup monté"() -> (w2128:string[][])
        n1389 = Concatenate Strings("人员" ("字符串"), w2134) -> (w2133:string)
        n1390 = call-poly <vilib>:"Read Key.vi"("section"="Setup", "error in (no error)"=w2137, "key"=w2133, "refnum"=w2139) -> ("error out"=w2124:errorcluster, "value"=w2132:string, "refnum out"=w2125:T3)  [unwired: 4 in, 1 out]
        n1391 = Replace Array Subset(array=w2128, new element=w2132, index (row)=w2131, index (col)=w2130) -> (w2127:string[][])
        n1392 = Index Array(array=w2127, index (row)=w2131, index (col)=w2130) -> (element=w2129:string)
        n1393 = local write "参数设置/Setup/Coup monté"(w2127) -> ()
      }
      n1394 = property on="Staff A" class="Ring (严格)"("Strings []"=w2120) -> ()  [unwired: 2 in, 2 out]
      n1395 = property on="Staff B" class="Ring (严格)"("Strings []"=w2120) -> ()  [unwired: 2 in, 2 out]
    }
    frame #7 {
      n1396 = property on="打印标签路径A/Print label path A/Imprimer le chemin d’accès de l’étiquette A" class="Path"() -> ("Label.Text"=w2145:string)  [unwired: 2 in, 2 out]
      n1397 = call-poly <vilib>:"Read Key.vi"("section"="Setup", "error in (no error)"=w2140, "key"=w2145, "refnum"=w2141) -> ("error out"=w2143:errorcluster, "value"=w2142:path, "refnum out"=w2144:T3)  [unwired: 4 in, 1 out]
      n1398 = property on="打印标签路径A/Print label path A/Imprimer le chemin d’accès de l’étiquette A" class="Path"("Value"=w2142) -> ()  [unwired: 2 in, 2 out]
    }
    frame #8 {
      n1399 = property on="打印标签路径B/Print label path B/Imprimer le chemin d’accès de l’étiquette B" class="Path"() -> ("Label.Text"=w2153:string)  [unwired: 2 in, 2 out]
      n1400 = call-poly <vilib>:"Read Key.vi"("section"="Setup", "error in (no error)"=w2150, "key"=w2153, "refnum"=w2151) -> ("error out"=w2148:errorcluster, "value"=w2147:path, "refnum out"=w2149:T3)  [unwired: 4 in, 1 out]
      n1401 = property on="打印标签路径B/Print label path B/Imprimer le chemin d’accès de l’étiquette B" class="Path"("Value"=w2147) -> ()  [unwired: 2 in, 2 out]
    }
    frame #9 {
      n1402 = call <vilib>:"Close Config Data.vi"("error in (no error)"=w2154, "refnum"=w2155) -> ()  [unwired: 8 in, 2 out]
    }
  }
